vi "Multichannel Lockin--DELETINGSTATES.vi"() -> ()   [LabVIEW 2019, in "Instrument.Lockin.lvclass"]
uses:
  Instrument.Lockin/Instrument.Lockin.lvclass
  <vilib>/Utility/error.llb/DialogType.ctl
  <vilib>/measure/NI_MAPro.lvlib
  <vilib>/Utility/config.llb/NI_LVConfig.lvlib
  <vilib>/JKI/JKI SMO/SMO/SMO.lvclass
  <userlib>/LevyLab/Instrument Framework/SMOs/RemoteControl/RemoteControl.lvclass
  <userlib>/LevyLab/Instrument Framework/SMOs/RemoteControl/Typedefs/Message--Cluster.ctl
  <userlib>/LevyLab/Instrument Framework/SMOs/RemoteControl/Typedefs/PrivateEvents--RemoteControl.Configure.ctl
  Instrument.DAQ/Typedefs/Results--Cluster.ctl
  Instrument.DAQ/Instrument.DAQ.lvclass
  Instrument.DAQ/Typedefs/Set State-enum.ctl
  <vilib>/JKI/JKI SMO/SMO/Typedefs/Reserve State--Enum.ctl
  <vilib>/JKI/JKI SMO/SMO/Typedefs/Public Events.ctl
  <vilib>/JKI/JKI SMO/SMO/Typedefs/SMOState --Enum.ctl
  Instrument.DAQ/Typedefs/DAQ.Sample Mode--Ring.ctl
  Instrument.DAQ/Typedefs/Sweep.Configuration--Cluster.ctl
  Instrument UI.Lockin/Instrument UI.Lockin.lvclass
  Instrument.DAQ/Typedefs/PublicEvents--DAQ.getSweepWaveforms.ctl
  Instrument.DAQ/Typedefs/PrivateEvents--DAQ.setCalibration.ctl
  Instrument.DAQ/Typedefs/Sweep.Pattern--Enum.ctl
  Instrument.DAQ/Typedefs/Sweep.Channel--Cluster.ctl
  Instrument.DAQ/Typedefs/DAQ.Sampling--Cluster.ctl
  Instrument UI.Lockin/private/Set Legend (WFChart).vi
  Instrument UI.Lockin/private/Set Legend (WFGraph).vi
  Instrument UI.Lockin/private/Set Legend (WDTWFGraph).vi
  Instrument UI.Lockin/private/Set All Plot Visibility (WFGraph).vi
  Instrument UI.Lockin/private/Set All Plot Visibility (WFChart).vi
  <vilib>/Platform/browser.llb/Open URL in Default Browser (string).vi
  <userlib>/LevyLab/Instrument Framework/SMOs/Instrument/Instrument.lvclass
  Instrument UI.Lockin/private/Set Plot Visibility (WFGraph).vi
  Instrument UI.Lockin/private/Set Plot Visibility (WFChart).vi
  <userlib>/LevyLab/Instrument Framework/SMOs/Logger.Error/Logger.Error.lvclass
  C:/Program Files (x86)/National Instruments/LabVIEW 2019/vi.lib/JKI/JKI SMO/SMO/SMO.lvclass
  Instrument UI.Lockin/private/Set All Plot Visibility (XYGraph).vi
  Instrument UI.Lockin/private/Set Plot Visibility (XYGraph).vi
  <userlib>/_OpenG.lib/error/error.llb/Filter Error Codes (Array)__ogtk.vi
  <vilib>/Waveform/WDTOps.llb/WDT Waveform Duration DBL.vi
  Instrument.DAQ/Typedefs/Sweep.Channel--Cluster--Array.ctl
  <vilib>/measure/maspectr.llb/FFT Power Spectrum and PSD for N Chan.vi
  Instrument.DAQ/Typedefs/DAQ.Config.AI.Coupling--enum.ctl
  Instrument.DAQ/Typedefs/DAQ.Config.AI.Range--enum.ctl
  Instrument.DAQ/Typedefs/DAQ.Config.AO.Range--enum.ctl
  Instrument.DAQ/Typedefs/AO.Channel.Function--Enum.ctl
  Instrument.DAQ/Typedefs/DAQ.Calibration--Cluster.ctl
  Instrument.DAQ/Typedefs/DAQ.Type--enum.ctl
  Instrument UI.Lockin/Typedefs/Display-Enum.ctl
  Instrument.DAQ/Typedefs/Simulation Mode--enum.ctl
  Instrument.Lockin/Typedefs/Lockin.Auto Sample Mode--Enum.ctl
  Instrument.DAQ/Typedefs/DAQ.Configuration--Cluster.ctl
  Instrument.DAQ/Typedefs/REF.Channel--Cluster.ctl
  Instrument.Lockin/Typedefs/Results Type--Enum.ctl
panel:
  out "Results Plot Names":string[](array[string])
  out "Version":string="vDevelopment" caption="V"
  in  "Tab Control 4":T1(tab)
  in  "Disable all AI Ref":bool
  in  "Enable only AI Ref1":bool
  in  "Reset Phase":bool
  in  "AI Channels":T2(array[cluster]) {"References" items=["", "1"]}
  in  "AO freq link":dbl=13.0 format="%.3p"
  in  "AO Amp Limit":dbl=0.009999999 format="%.3p"
  in  "Limit Amplitudes":bool
  in  "Link Frequencies":bool
  in  "LP f (Hz)":dbl=100.0 format="%.3p"
  in  "Line":bool
  in  "Lowpass":bool
  in  "AO Channels":T4(array[cluster]) {"Phase" format="%.3g"; "Frequency" min=0.0001 max=10000.0 format="%.3g"; "Offset" format="%.3p"; "Amplitude" min=0.0 max=10.0 format="%.3p"}
  in  "REF Channels":T5[](array[typedef]) {"Roll-Off" min=1; "TC" min=0.0001 format="%#_3p"; "Phase" format="%.3g"; "Frequency" min=0.0001 max=10000.0 format="%.3g"; "Channel" min=1}
  in  "DAQ Config":T6[](array[typedef]) {"AI.Coupling" items=["AC"=10045, "DC"=10050, "GND"=10066]}
  in  "auto DAQ":bool
  in  "Max Fs Refresh Rate (Hz)":dbl=10.0 format="%#_13g"
  in  "Sampling Mode":T10
  in  "Sampling":T11={"Fs"=10000.0, "#s"=1000}
  in  "DAQ Type":T12=enum."PXI 446x"
  in  "Auto x*F1":dbl=5000.0 format="%#_13g"
  in  "Load Configuration":bool
  in  "Save Configuration":bool
  in  "AI Simulation mode":T13=enum."AI = noise*AO"
  in  "decimating factor":i32=1
  in  "Remove":bool
  in  "Measure":bool
  in  "Channels: Sweep":T15(array[cluster]) {"Channel" items=["AO1"=1, "AO2"=2, "AO3"=3, "AO4"=4, "AO5"=5, "AO6"=6, "AO7"=7, "AO8"=8]; "Start" format="%#_6p"; "End" format="%#_6p"}
  in  "Stop Sweep":bool caption="Stop"
  in  "Sweep Time (s)":dbl=20.0 format="%#_1f"
  in  "Start Sweep":bool caption="Start"
  in  "Initial Wait (s)":dbl=1.0
  out "Sweep Timer (s)":dbl caption="Timer (s)"
  in  "Return to Start?":bool
  out "Sampling Status":string="Good"
  in  "Output Gain":cluster{"AI.Ch":string, "Gain":dbl}[](array[cluster])=[{"AI.Ch"="AO1", "Gain"=1.0}, {"AI.Ch"="AO2", "Gain"=1.0}, {"AI.Ch"="AO3", "Gain"=1.0}, {"AI.Ch"="AO4", "Gain"=1.0}, {"AI.Ch"="AO5", "Gain"=1.0}, {"AI.Ch"="AO6", "Gain"=1.0}, {"AI.Ch"="AO7", "Gain"=1.0}, {"AI.Ch"="AO8", "Gain"=1.0}, {"AI.Ch"="AO9", "Gain"=1.0}, {"AI.Ch"="AO10", "Gain"=1.0}, {"AI.Ch"="AO11", "Gain"=1.0}, {"AI.Ch"="AO12", "Gain"=1.0}, {"AI.Ch"="AO13", "Gain"=1.0}, {"AI.Ch"="AO14", "Gain"=1.0}, {"AI.Ch"="AO15", "Gain"=1.0}, {"AI.Ch"="AO16", "Gain"=1.0}]
  in  "Input Gain":cluster{"AI.Ch":string, "Gain":dbl}[](array[cluster])=[{"AI.Ch"="AI1", "Gain"=1.0}, {"AI.Ch"="AI2", "Gain"=1.0}, {"AI.Ch"="AI3", "Gain"=1.0}, {"AI.Ch"="AI4", "Gain"=1.0}, {"AI.Ch"="AI5", "Gain"=1.0}, {"AI.Ch"="AI6", "Gain"=1.0}, {"AI.Ch"="AI7", "Gain"=1.0}, {"AI.Ch"="AI8", "Gain"=1.0}, {"AI.Ch"="AI9", "Gain"=1.0}, {"AI.Ch"="AI10", "Gain"=1.0}, {"AI.Ch"="AI11", "Gain"=1.0}, {"AI.Ch"="AI12", "Gain"=1.0}, {"AI.Ch"="AI13", "Gain"=1.0}, {"AI.Ch"="AI14", "Gain"=1.0}, {"AI.Ch"="AI15", "Gain"=1.0}, {"AI.Ch"="AI16", "Gain"=1.0}]
  out "State History":string=" Exit\r Data: Cleanup\r Events: Unregister\r UI: Cleanup\r UI: Disable Buttons\r Configuration: Write\r Error Logger: Destroy\r Lockin SMO: Stop\r Remote SMO: Stop\r Macro: Exit\r UI: Update Sweep Timer\r UI: Update Lockin Graphs\r UI: Update Waveform Graphs\r 4461: OUT\r UI: Update Sweep Timer\r UI: Update Lockin Graphs\r UI: Update Waveform Graphs\r 4461: OUT\r UI: Update Sweep Timer\r UI: Update Lockin Graphs\r UI: Update Waveform Graphs\r 4461: OUT"
  out "Refresh time (ms)":u32=103
  out "LockinDAQ SMO State":T16=enum."Stopped" caption="SMO State"
  out "RC SMO State":T16=enum."Stopped" caption="SMO State"
  in  "Update":bool
  in  "Enable Output":bool caption="Enable"
  in  "Output Channel":i32=1 min=1
  out "Output (V)":dbl
  in  "AI Channel":i32=1
  in  "Reference Channel":i32=1
  in  "Type":T17
  in  "Allowed remote system":string
  in  "Get Calibration":bool
  out "Cal Info":T18[](array[typedef]) {"SelfCal.LastDate/Time" format="%<%I:%M %p\n%m/%d/%Y>T"}
  in  "Self Calibrate":bool
  in  "Tab Control 3":enum32{"Page 1"}(tab)
  out "X":dbl=0.0014996100939563214 caption="X (V)" format="%#_3p"
  out "Y":dbl=-29.79492153733761 caption="Y (V)" format="%#_3p"
  in  "Channel":i32(ring)=1
  out "R":dbl=0.0014996100939563214 caption="R (V)" format="%#_3p"
  out "Theta":dbl=-29.79492153733761 caption="Theta (°)" format="%#_3p"
  in  "Display":T19=enum."R and Theta" caption="Enum"
  in  "Close":bool
  out "Status":string="Shutdown"
  in  "Pause":bool
  in  "Reset":bool
  in  "Start":bool
  in  "Help":bool
  in  "Trigger":bool
  in  "Tab Control 2":T20(tab)
  in  "AI Graph All":bool
  in  "AI Graph None":bool
  in  "Y Axis (Output)":enum16{"Analog Output", "Reference"}(ring) caption="Enum 3"
  in  "Y Axis (Input)":enum16{"Device", "ADC"}(ring) caption="Enum 3"
  in  "Decimate":enum16{"1", "10", "100", "1000"}(ring) caption="Enum 3"
  in  "X Axis":enum16{"Time", "Samples"}(ring) caption="Enum 3"
  out "AI Graph":waveform(dbl)[](graph)
  out "AO Graph":waveform(dbl)[](graph)
  in  "AO Graph All":bool
  in  "AO Graph None":bool
  in  "Y/Theta Range":dbl caption="Axis Range" format="%#_6p"
  in  "X/R Range":dbl caption="Axis Range" format="%#_6p"
  out "Lockin 2":waveform(dbl)[](graph) caption="Lockin Display 2"
  out "Lockin 1":waveform(dbl)[](graph)
  in  "Lockin 1 None":bool
  in  "Lockin 1 All":bool
  out "Results":string[][](table)
  out "XY Graph":cluster{"Wavenumber":dbl[], "Data":dbl[]}[](graph)
  in  "Numeric":dbl caption="Axis Range" format="%#_6p"
  out "Sweep Results Y":waveform(dbl)[](graph)
  out "Sweep Results X":waveform(dbl)[](graph)
  out "Sweep Results AI":waveform(dbl)[](graph)
  out "Sweep Results AO":waveform(dbl)[](graph)
  in  "# averages":u32=10 min=1
  in  "weighting mode":enum16{"Linear", "Exponential"}(ring)=enum."Exponential"
  in  "averaging mode":T21(ring)=enum."RMS averaging"
  in  "window":u16(ring) items=["Rectangle", "Hanning"]
  in  "export mode":u16(ring)=1 items=["Power Spectrum", "Power Spectral Density"]
  in  "restart":bool
  out "done?":bool=TRUE
  out "PS Chart":dbl[][](graph)
  out "PS WFGraph":cluster{"f0":dbl, "df":dbl, "magnitude":dbl[]}[](graph)
  out "averages":dbl=180.0
  # "Output"
  # "Input"
  # ">> DEVICE >>"
  # "Amp (V)"
  # "(*)"
  # "Ch"
  # "DC (V)"
  # "f (Hz)"
  # "Phase (°)"
  # "Function"
  # "Sweep"
  # "(*)"
  # "Ch"
  # "Ref1   2     3    4"
  # "Input: Pre-Filter"
  # "Output Settings"
  # "Reference"
  # "Reference Settings"
  # "Ch"
  # "f (Hz)"
  # "Phase (°)"
  # "TC (s)"
  # "Order"
  # "DAQ Channels"
  # "AI"
  # "Device"
  # "AO"
  # "Input: Offset"
  # "Ch"
  # "Range"
  # "Ch"
  # "Range"
  # "Coupling"
  # "Other Configuration"
  # "Sampling"
  # "Changing settings in this box will automatically\nreset the lockin and restart acquisition"
  # "Sweep"
  # "Channel"
  # "Start"
  # "End"
  # "Pattern"
  # "Status"
  # "Channel"
  # "Channel"
  # "Input Gain"
  # "Output Gain"
  # "Auxiliary Output"
  # "Configuration"
  # "- Use to control an auxiliiary card such as a multifunction DAQ (6115, 6120, etc)"
  # "Forward Lockin Input --> Lockin Output"
  # "- Choose an input lockin channel and value (X,Y, etc) and it will be written as a DC value to an output channel of your choosing.\n- Output is scaled by the input amplifier gain."
  # "Calibration"
  # "Self Cal\nLast Time"
  # "Self Cal\nLast Temp"
  # "Temp\nNow"
  # "Cal\nDue"
  # "Device"
  # "AI Graph"
  # "AO/Reference Graph"
  # "Lockin Results 1"
  # "Lockin Results 2"
  # "Lockin Results 2"
  # "Sweep Results"
  # "Sweep AO/AI"
  # "Power Spectra"
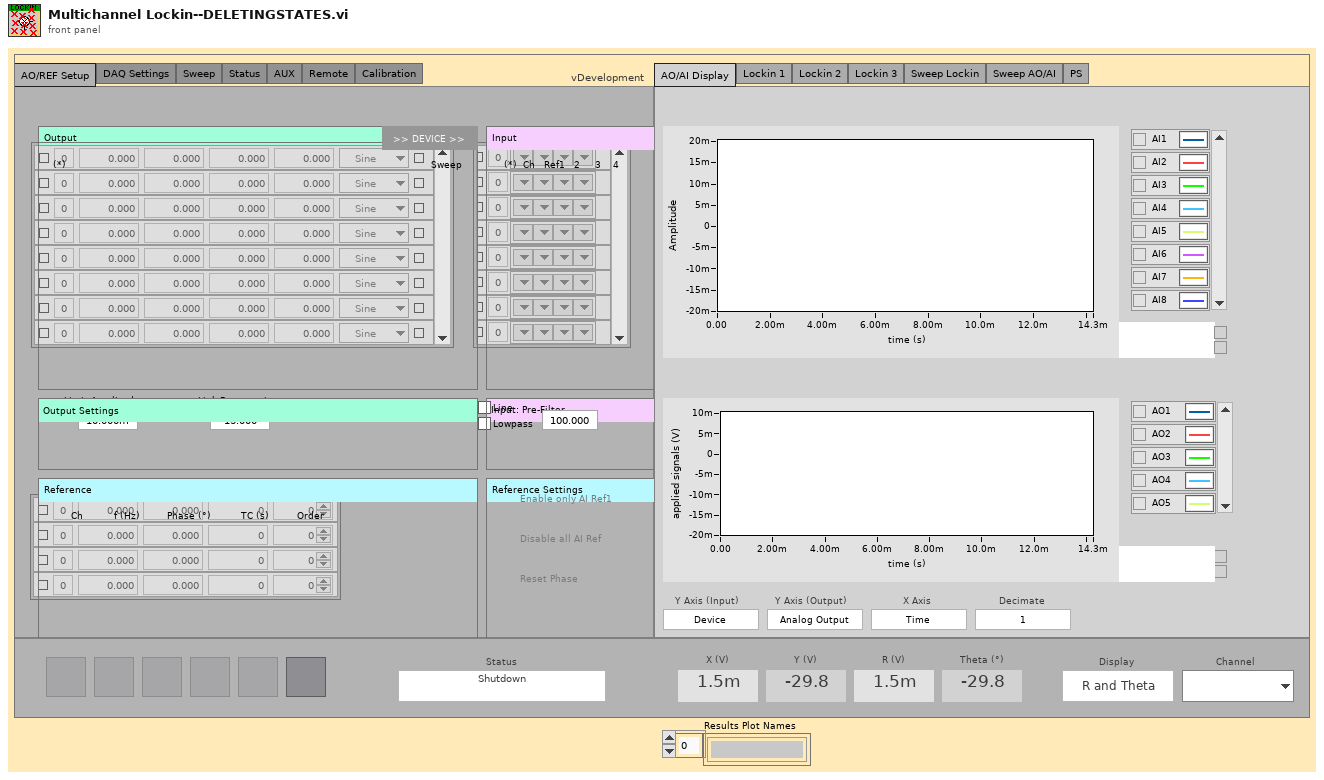
[diagram p1: front panel]
types:
  T1 = enum32{"AO/REF Setup", "DAQ Settings", "Sweep", "Status", "AUX", "Remote", "Calibration"}
  T2 = cluster{"Enable?":bool, "Channel":i32, "References":u16[]}[]
  T3 = typedef "Instrument.DAQ.lvclass/AO.Channel.Function--Enum.ctl" = enum16{"Sine", "Triangle", "Square"}
  T4 = cluster{"Enable?":bool, "Channel":i32, "Amplitude":dbl, "Offset":dbl, "Frequency":dbl, "Phase":dbl, "Function":T3, "Sweeping?":bool}[]
  T5 = typedef "Instrument.DAQ.lvclass/REF.Channel--Cluster.ctl" = cluster{"Enable?":bool, "Channel":i32, "Frequency":dbl, "Phase":dbl, "TC":dbl, "Roll-Off":i32}
  T6 = typedef "Instrument.DAQ.lvclass/DAQ.Configuration--Cluster.ctl" = cluster{"Device":string, "AO.Ch":string, "AO.Range":T7, "AI.Ch":string, "AI.Range":T8, "AI.Coupling":T9}
  T7 = typedef "Instrument.DAQ.lvclass/DAQ.Config.AO.Range--enum.ctl" = enum16{"±0.1", "±1.0", "±10.0"}
  T8 = typedef "Instrument.DAQ.lvclass/DAQ.Config.AI.Range--enum.ctl" = enum16{"±0.316", "±1.00", "±3.16", "±10.0", "±31.6", "±42.4"}
  T9 = typedef "Instrument.DAQ.lvclass/DAQ.Config.AI.Coupling--enum.ctl" = u16
  T10 = typedef "Instrument.Lockin.lvclass/Lockin.Auto Sample Mode--Enum.ctl" = enum16{"Manual", "Auto Fs", "Max Fs"}
  T11 = typedef "Instrument.DAQ.lvclass/DAQ.Sampling--Cluster.ctl" = cluster{"Fs":dbl, "#s":i32}
  T12 = typedef "Instrument.DAQ.lvclass/DAQ.Type--enum.ctl" = enum16{"None", "USB 4431", "PXI 446x"}
  T13 = typedef "Instrument.DAQ.lvclass/Simulation Mode--enum.ctl" = enum16{"AI = HW simulated", "AI = noise*AO", "AI = waveguide"}
  T14 = typedef "Instrument.DAQ.lvclass/Sweep.Pattern--Enum.ctl" = enum16{"Ramp /", "Ramp /\\", "Smooth Ramp _/", "Smooth Ramp _/\\_", "Frequency"}
  T15 = cluster{"Enable?":bool, "Channel":u16, "Start":dbl, "End":dbl, "Pattern":T14}[]
  T16 = typedef "SMO.lvclass/SMOState --Enum.ctl" = enum16{"unknown", "Created", "Started", "Stopped"}
  T17 = typedef "Instrument.Lockin.lvclass/Results Type--Enum.ctl" = enum16{"X", "Y", "R", "Theta", "Mean"}
  T18 = typedef "Instrument.DAQ.lvclass/DAQ.Calibration--Cluster.ctl" = cluster{"Active Device":string, "SelfCal.LastDate/Time":dbl, "SelfCal.LastTemp":dbl, "DevTemp":dbl, "calibration due?":bool}
  T19 = typedef "Instrument UI.Lockin.lvclass/Display-Enum.ctl" = enum16{"X and Y", "R and Theta", "Mean"}
  T20 = enum32{"AO/AI Display", "Lockin 1", "Lockin 2", "Lockin 3", "Sweep Lockin", "Sweep AO/AI", "PS"}
  T21 = enum16{"No averaging", "Vector averaging", "RMS averaging", "Peak hold"}
  T22 = typedef "Instrument.DAQ.lvclass/Set State-enum.ctl" = enum16{"start", "stop", "reset", "start sweep", "stop sweep"}
  T23 = typedef "Instrument.DAQ.lvclass/PrivateEvents--DAQ.setCalibration.ctl" = enum16{"Check", "Calibrate"}
  T24 = typedef "Instrument.DAQ.lvclass/Sweep.Configuration--Cluster.ctl" = cluster{"Sweep Time (s)":dbl, "Initial Wait (s)":dbl, "Return to Start":bool, "Channels":T25}
  T25 = typedef "Instrument.DAQ.lvclass/Sweep.Channel--Cluster--Array.ctl" = T26[]
  T26 = typedef "Instrument.DAQ.lvclass/Sweep.Channel--Cluster.ctl" = cluster{"Enable?":bool, "Channel":u16, "Start":dbl, "End":dbl, "Pattern":T14}
  T27 = enum32{"invalid app kind", "Development System", "Run Time System", "Student Edition", "Embedded LabVIEW", "Evaluation", "Custom"}
  T28 = enum32{"AO/REF Setup", "DAQ Settings", "Sweep", "Status", "AUX", "Remote", "Calibration", "Save"}
  T29 = enum8{"Enabled", "Disabled", "Disabled and Grayed Out"}
  T30 = enum32{"Invalid", "Standard", "Closed", "Hidden", "Minimized", "Maximized"}
  T31 = cluster{"averaging mode":enum16{"No averaging", "Vector averaging", "RMS averaging", "Peak hold"}, "weighting mode":enum16{"Linear", "Exponential"}, "number of averages":u32}
  T32 = typedef "Instrument.DAQ.lvclass/Get State-enum.ctl" = enum16{"idle", "created", "started", "stopped", "sweeping"}
  T33 = typedef "RemoteControl.lvclass/PrivateEvents--RemoteControl.Configure.ctl" = cluster{"address":string, "Port":u16, "AllowedRemote":string, "Commands":string[], "timeout":i32}
  T34 = typedef "RemoteControl.lvclass/Message--Cluster.ctl" = cluster{"Command":string, "Data":variant, "ID":string}
  T35 = typedef "Instrument.DAQ.lvclass/PublicEvents--DAQ.getSweepWaveforms.ctl" = cluster{"Sweep AO":waveform(dbl)[], "Sweep AI":waveform(dbl)[], "Sweep Results X":waveform(dbl)[], "Sweep Results Y":waveform(dbl)[]}
  T36 = cluster{"Core":cluster{"Current VI Reference":refnum<vi>, "Close Panel on Exit?":bool}, "to":i32, "Lockin":refnum<class "Instrument.Lockin.lvclass">, "RemoteControl":refnum<class "RemoteControl.lvclass">, "Lockin.DAQ":refnum<class "Instrument.DAQ.lvclass">, "Logger.Error":refnum<class "Logger.Error.lvclass">, "RemoteControl.Configure":T33, "Message":T34, "HandledMessage":T34, "SweepWaveforms":T35}
  T37 = typedef "Instrument.DAQ.lvclass/State-enum.ctl" = enum16{"idle", "created", "started", "stopped", "sweeping"}
  T38 = typedef "Instrument.DAQ.lvclass/REF.Channel--Cluster--Array.ctl" = T5[]
  T39 = typedef "Instrument.DAQ.lvclass/DAQ Configuration--Cluster--Array.ctl" = T40[]
  T40 = typedef "Instrument.DAQ.lvclass/DAQ Configuration--Cluster.ctl" = cluster{"Device":string, "AO.Ch":string, "AO.Range":T41, "AI.Ch":string, "AI.Range":T42, "AI.Coupling":T43}
  T41 = typedef "Instrument.DAQ.lvclass/446xAO-enum.ctl" = enum16{"±0.1", "±1.0", "±10.0"}
  T42 = typedef "Instrument.DAQ.lvclass/446xAI-enum.ctl" = enum16{"±0.316", "±1.00", "±3.16", "±10.0", "±31.6", "±42.4"}
  T43 = typedef "Instrument.DAQ.lvclass/AI.coupling-enum.ctl" = u16
  T44 = typedef "Instrument.DAQ.lvclass/DAQ.Config.AO--Cluster--Array.ctl" = T45[]
  T45 = typedef "Instrument.DAQ.lvclass/DAQ.Config.AO--Cluster.ctl" = cluster{"Channels":tag, "Range":T7, "output terminal configuration":i32, "Type":T12}
  T46 = typedef "Instrument.DAQ.lvclass/DAQ.Config.AI--Cluster--Array.ctl" = T47[]
  T47 = typedef "Instrument.DAQ.lvclass/DAQ.Config.AI--Cluster.ctl" = cluster{"Channels":tag, "Coupling":T9, "Range":T8, "input terminal configuration":i32, "Type":T12}
  T48 = typedef "Instrument.DAQ.lvclass/DAQ.Sample Mode--Ring.ctl" = i32
  T49 = typedef "DialogType.ctl" = u16
  T50 = typedef "Instrument.DAQ.lvclass/Results--Cluster.ctl" = cluster{"Time Stamp":timestamp, "Results (Dictionary)":cluster{"key":string, "value":dbl}[]}
  T51 = cluster{"Current VI Reference":refnum<vi>, "Close Panel on Exit?":bool}
  T52 = typedef "Instrument.DAQ.lvclass/AO.Channel--Cluster--Array.ctl" = T53[]
  T53 = typedef "Instrument.DAQ.lvclass/AO.Channel--Cluster.ctl" = cluster{"Enable?":bool, "Channel":i32, "Amplitude":dbl, "Offset":dbl, "Frequency":dbl, "Phase":dbl, "Function":T3, "Sweeping?":bool}
  T54 = typedef "SMO.lvclass/Public Events.ctl" = cluster{"Error":refnum<user-event>, "State":refnum<user-event>, "Reserve State":refnum<user-event>}
  T55 = typedef "RemoteControl.lvclass/PublicEvents--Cluster.ctl" = cluster{"SendMessageFromProcess":refnum<user-event>}
  T56 = typedef "Instrument.DAQ.lvclass/PublicEvents--Cluster.ctl" = cluster{"getAIChannels":refnum<user-event>, "getAOChannels":refnum<user-event>, "getREFChannels":refnum<user-event>, "getWaveforms":refnum<user-event>, "getResults":refnum<user-event>, "getSweepWaveforms":refnum<user-event>, "getCalibration":refnum<user-event>, "getDAQState":refnum<user-event>, "getDAQconfig":refnum<user-event>}
  T57 = typedef "Instrument.DAQ.lvclass/AI.Channel--Cluster--Array.ctl" = T58[]
  T58 = typedef "Instrument.DAQ.lvclass/AI.Channel--Cluster.ctl" = cluster{"Enable?":bool, "Channel":i32, "References":i32[]}
  T59 = typedef "Instrument.DAQ.lvclass/Configuration.Prefilter--Cluster.ctl" = cluster{"60 Hz":bool, "Low Pass":bool, "Low Pass Cutoff (Hz)":dbl}
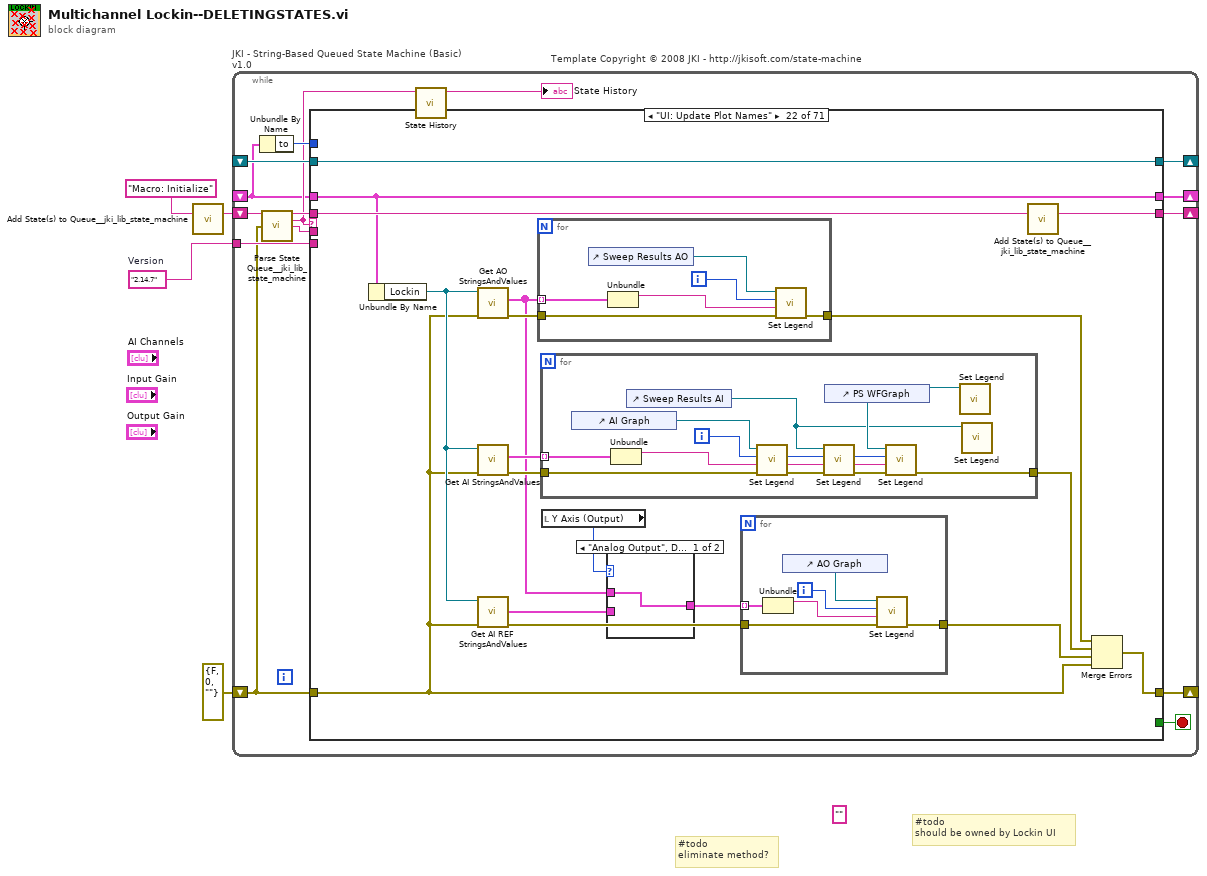
[diagram p0: block diagram]
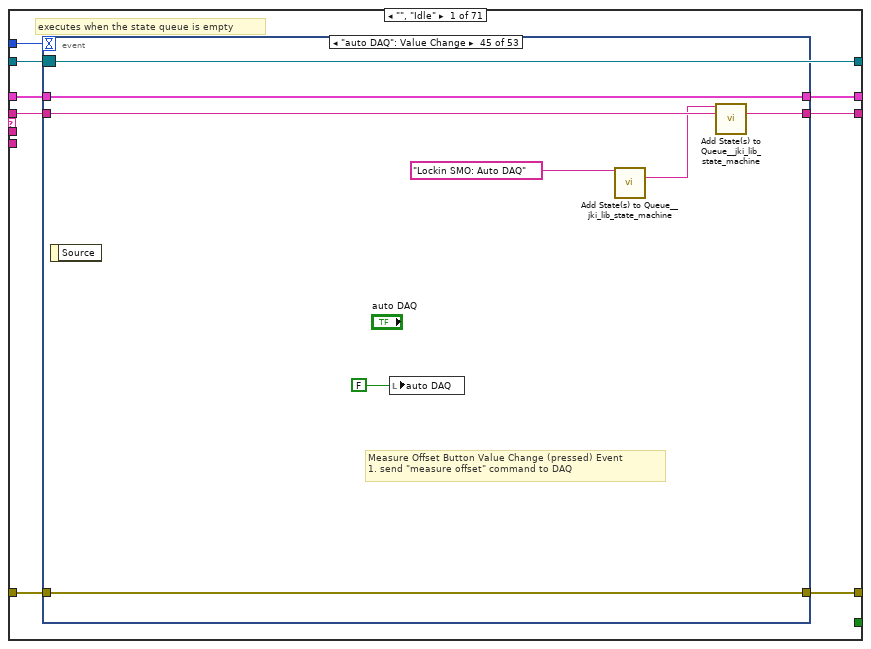
[diagram p2: hidden frame]
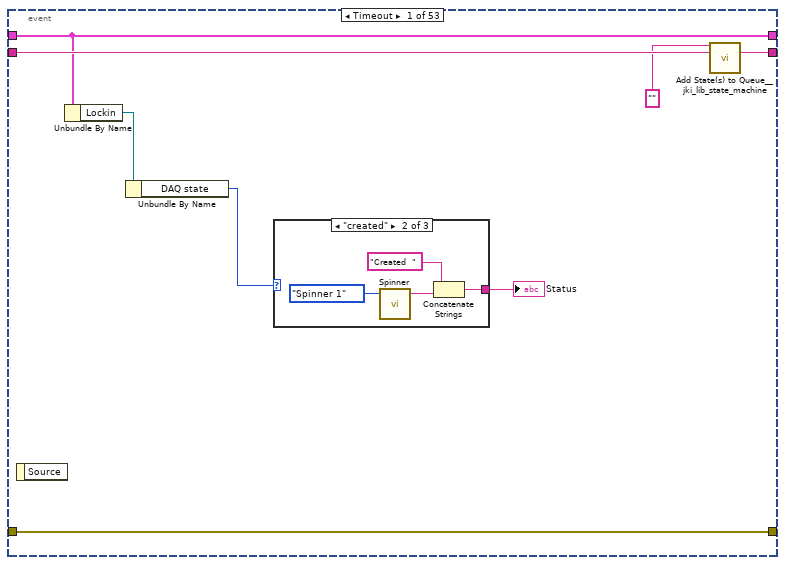
[diagram p3: hidden frame]
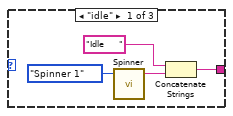
[diagram p4: hidden frame]
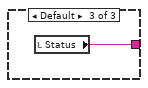
[diagram p5: hidden frame]
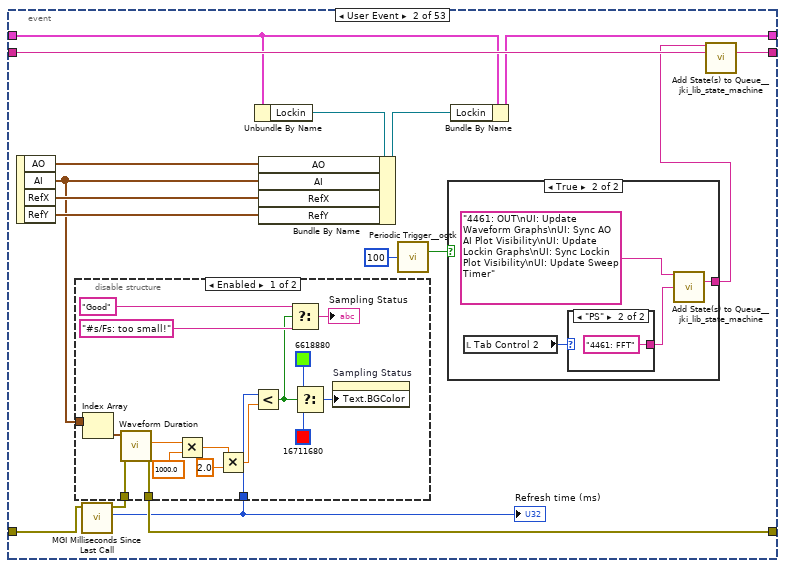
[diagram p6: hidden frame]
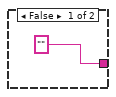
[diagram p7: hidden frame]
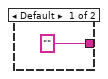
[diagram p8: hidden frame]
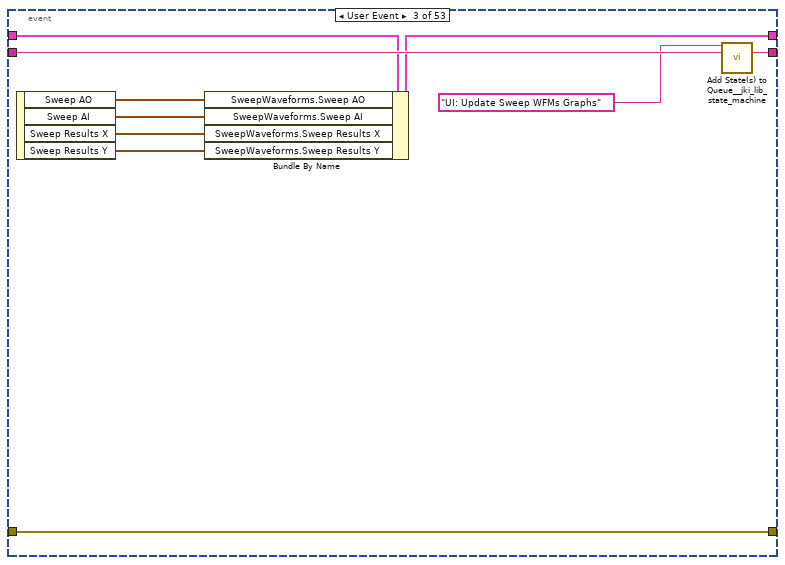
[diagram p10: hidden frame]
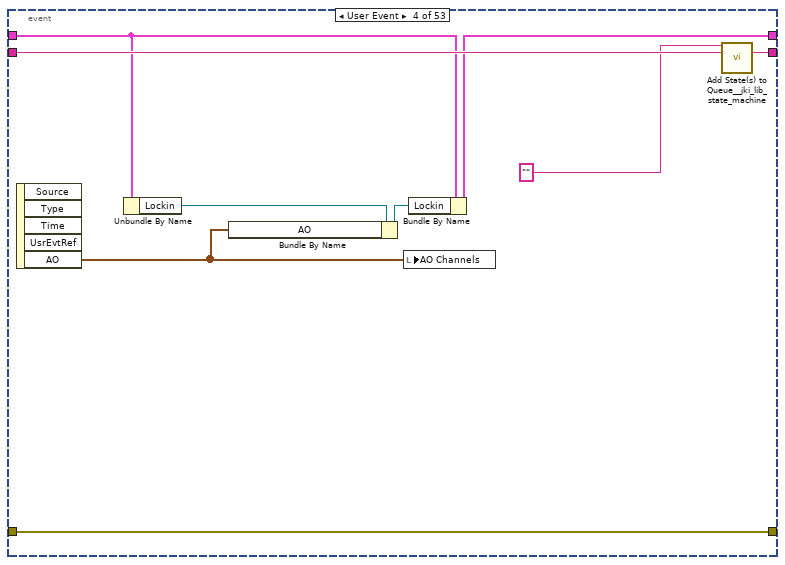
[diagram p11: hidden frame]
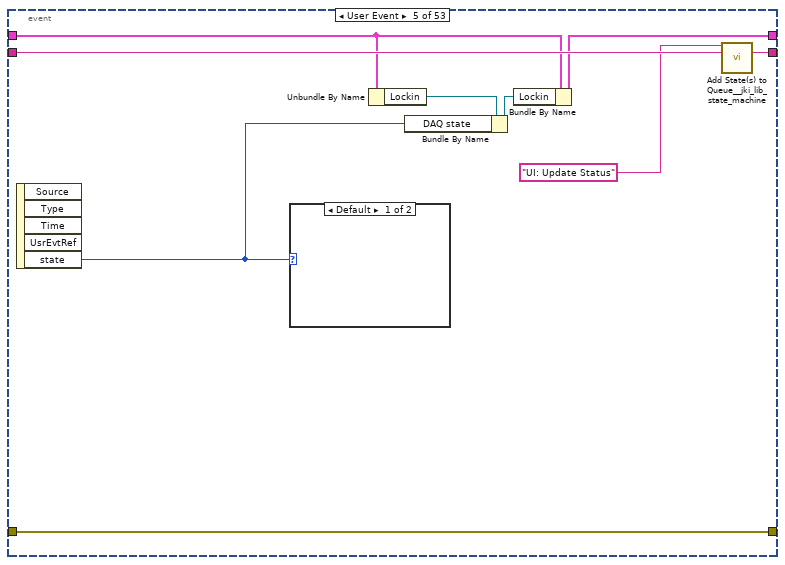
[diagram p12: hidden frame]
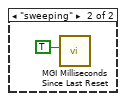
[diagram p13: hidden frame]
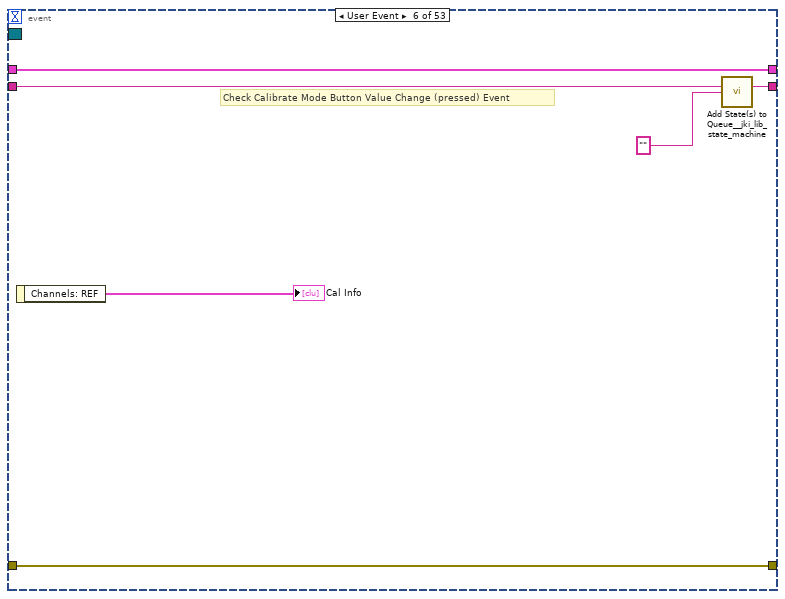
[diagram p14: hidden frame]
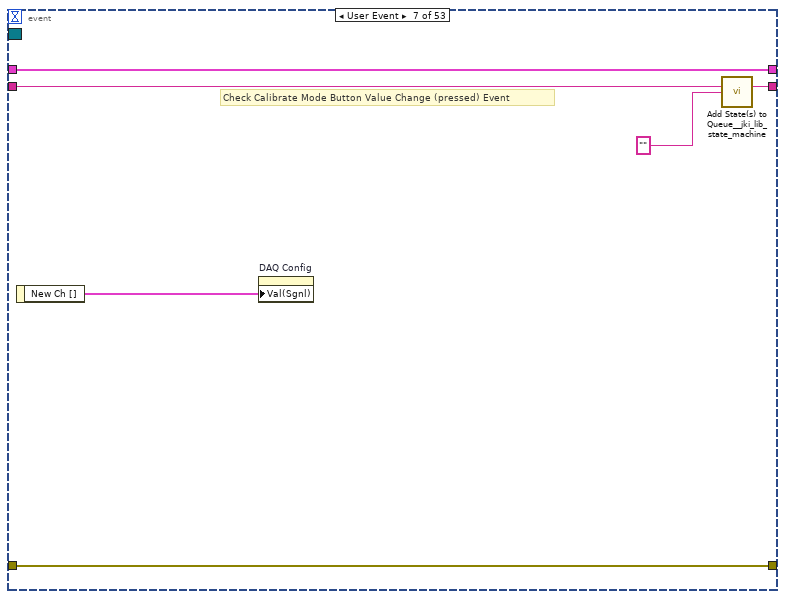
[diagram p15: hidden frame]
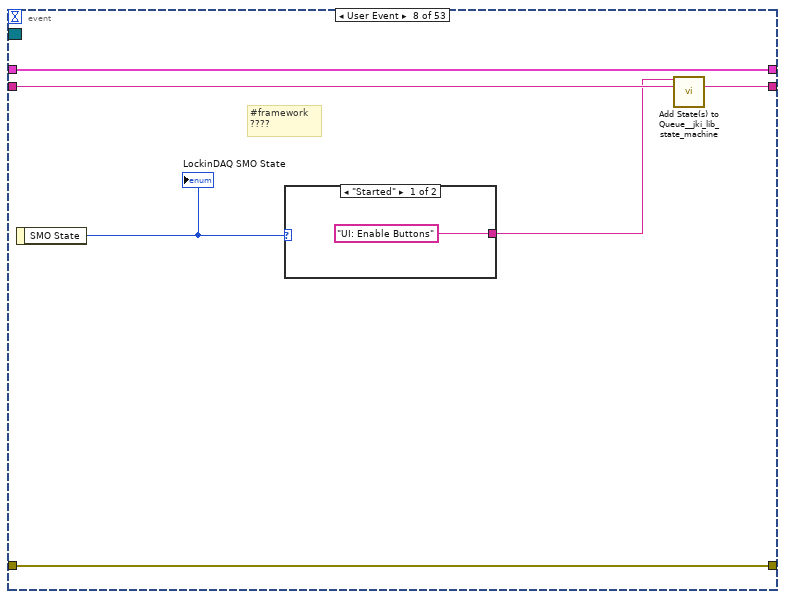
[diagram p16: hidden frame]
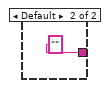
[diagram p17: hidden frame]
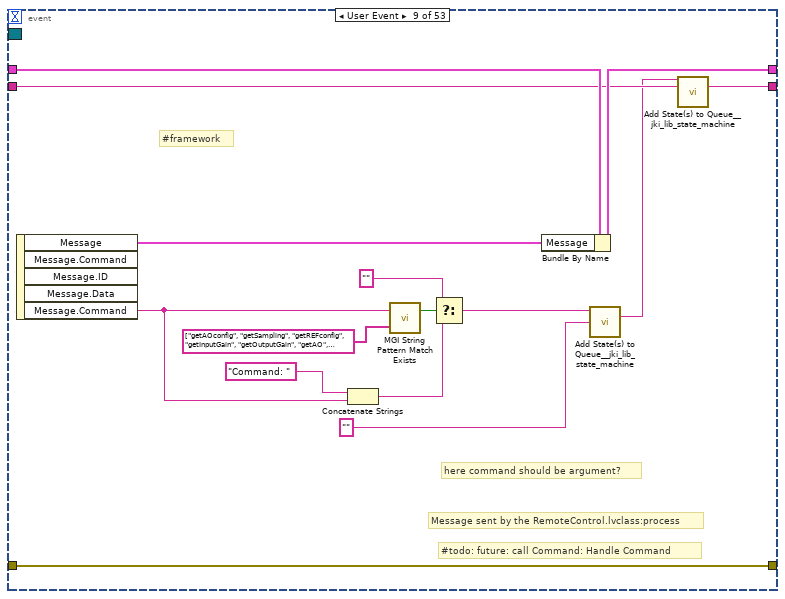
[diagram p18: hidden frame]
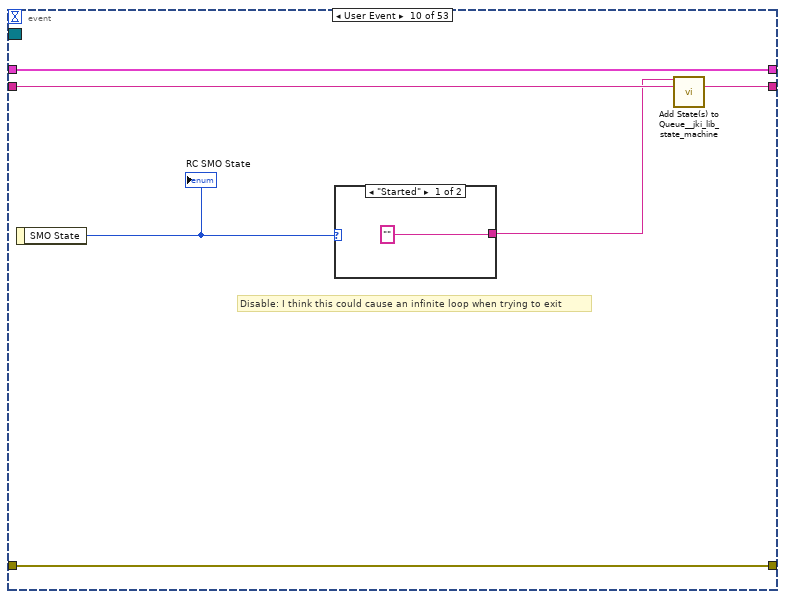
[diagram p19: hidden frame]
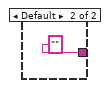
[diagram p20: hidden frame]
diagram:
  (unwired) "" ("State(s) in Front (\"\")")
  w2 = "2.14.7"  # Version
  # "#todo\nshould be owned by Lockin UI"
  # "#todo\neliminate method?"
  # "Template Copyright © 2008 JKI - http://jkisoft.com/state-machine"
  n1 = call <vilib>:"Add State(s) to Queue__jki_lib_state_machine.vi"("State(s) in (\"\")"="Macro: Initialize") -> ("States Out"=w4:string)  [unwired: 14 in]
  n2 = while "JKI - String-Based Queued State Machine (Basic) v1.0" {
    shift-right: [w11] -> _
    shift-left: _ -> [w5]
    shift-right: [w8] -> _
    shift-left: errorcluster {"status"=FALSE, "code"=0, "source"=""} ("error out") -> [w6]
    shift-right: [w18] -> _
    shift-left: w4 -> [w15]
    shift-right: [w12] -> _
    shift-left: _ -> [w13]
    tunnel: w2 -> [w7]
    stop <- w17 stop-if-true
    n3 = Unbundle By Name(w5) -> ("to"=w14:i32)
    n4 = call <vilib>:"Parse State Queue__jki_lib_state_machine.vi"("State Queue"=w15, "Error In (no error)"=w6) -> ("Remaining States"=w16:string, "Current State"=w9:string, "Arguments"=w19:string)  [unwired: 11 in]
    n5 = case shown="\"UI: Update Plot Names\"" w9 {
      selector: w9 -> [_ _ w594 _ _ _ _ _ _ _ _ _ _ _ _ _ _ _ _ _ _ _ _ _ _ _ _ _ _ _ _ _ _ _ _ _ _ _ _ _ _ _ _ _ _ _ _ _ _ _ _ _ _ _ _ _ _ _ _ _ _ _ _ _ _ _ _ _ _ _ _]
      tunnel: w19 -> [_ _ _ _ _ _ _ _ _ _ _ _ _ _ _ _ _ _ w780 _ _ _ _ _ _ _ w1000 w1014 w1033 _ _ _ _ _ _ _ _ _ w1195 w1205 _ _ _ _ _ _ _ _ w1334 _ _ w1374 _ _ _ _ _ _ _ w1461 _ _ _ _ _ _ _ _ _ _ _]
      tunnel: [w26 w590 w597 w615 w628 w640 w645 w660 w681 w688 w693 w718 w724 w729 w745 w756 w767 w778 w791 w811 w829 w850 w892 w949 w978 w991 w1004 w1017 w1036 w1067 w1097 w1110 w1121 w1129 w1145 w1152 w1160 w1180 w1196 w1208 w1240 w1245 w1252 w1257 w1265 w1303 w1325 w1330 w1340 w1360 w1369 w1381 w1392 w1409 w1421 w1430 w1439 w1448 w1457 w1468 w1475 w1482 w1489 w1496 w1501 w1515 w1543 w1583 w1592 w1597 w1602] -> w18
      tunnel: [_ _ _ _ _ TRUE _ _ _ _ _ _ _ _ _ _ _ _ _ _ _ _ _ _ _ _ _ _ _ _ _ _ _ _ _ _ _ _ _ _ _ _ _ _ _ _ _ _ _ _ _ _ _ _ _ _ _ _ _ _ _ _ _ _ _ _ _ _ _ _ _] -> w17
      tunnel: w14 -> [w21 _ _ _ _ _ _ _ _ _ _ _ _ _ _ _ _ _ _ _ _ _ _ _ _ _ _ _ _ _ _ _ _ _ _ _ _ _ _ _ _ _ _ _ _ _ _ _ _ _ _ _ _ _ _ _ _ _ _ _ _ _ _ _ _ _ _ _ _ _ _]
      tunnel: w16 -> [w27 w591 w598 w616 w629 w641 w646 w661 w682 w689 w694 w719 w725 w730 w746 w757 w768 w779 w792 w812 w830 w851 w893 w950 w979 w992 w1005 w1018 w1037 w1068 w1098 w1111 w1122 w1130 w1146 w1153 w1161 w1181 w1197 w1209 w1241 w1246 w1247 w1258 w1266 w1304 w1326 w1331 w1341 w1361 w1370 w1382 w1393 w1410 w1422 w1431 w1440 w1449 w1458 w1469 w1476 w1483 w1490 w1497 w1502 w1516 w1542 w1579 w1593 w1598 w1603]
      tunnel: w13 -> [w20 w588 w593 w604 w624 w637 w643 w658 w680 w687 w691 _ w721 w726 w743 w755 w766 w777 w790 w810 w828 w849 w890 w948 w975 w988 w1002 w1015 w1034 w1066 w1096 w1108 w1118 w1126 w1143 w1150 w1158 w1177 w1193 w1202 w1238 w1242 w1250 w1254 w1264 w1301 w1318 w1327 w1339 w1359 w1368 w1380 w1391 w1408 w1420 w1429 w1438 w1447 w1456 w1467 w1474 w1481 w1488 w1495 w1498 w1514 w1541 w1580 w1589 w1594 w1599]
      tunnel: [w20 w588 w593 w604 w624 w637 w643 w658 w680 w687 w691 w717 w721 w726 w743 w755 w766 w777 w790 w810 w828 w849 w890 w948 w975 w988 w1002 w1015 w1034 w1066 w1096 w1108 w1118 w1126 w1143 w1150 w1158 w1177 w1193 w1202 w1238 w1242 w1250 w1254 w1264 w1301 w1318 w1327 w1339 w1359 w1368 w1380 w1391 w1408 w1420 w1429 w1438 w1447 w1456 w1467 w1474 w1481 w1488 w1495 w1498 w1514 w1541 w1580 w1589 w1594 w1599] -> w12
      tunnel: [w23 w587 w596 w614 w621 w636 w642 w655 w667 w684 w690 w716 w723 w727 w744 w754 w765 w776 w789 w809 w827 w837 w891 w944 w976 w989 w1003 w1016 w1035 w1058 w1095 w1109 w1119 w1127 w1142 w1149 w1156 w1178 w1194 w1204 w1239 w1243 w1248 w1255 w1260 w1289 w1319 w1328 w1332 w1353 w1363 w1372 w1385 w1400 w1416 w1427 w1432 w1445 w1452 w1466 w1473 w1480 w1484 w1492 w1499 w1507 w1537 w1577 w1590 w1595 w1600] -> w11
      tunnel: [w25 w589 w600 w613 w622 w639 w644 w653 w663 w683 w692 w697 w720 w728 w742 w747 w758 w770 w787 w798 w814 w847 w881 w945 w977 w990 w995 w1008 w1021 w1046 w1083 w1104 w1120 w1128 w1144 w1151 w1159 w1179 w1191 w1203 w1236 w1244 w1251 w1256 w1259 w1302 w1324 w1329 w1336 w1356 w1365 w1377 w1388 w1401 w1418 w1424 w1436 w1441 w1450 w1463 w1470 w1477 w1485 w1491 w1500 w1503 w1538 w1560 w1591 w1596 w1601] -> w8
      tunnel: w7 -> [_ _ _ _ _ _ _ _ _ _ _ _ _ _ w733 _ _ _ _ _ _ _ _ _ _ _ _ _ _ _ _ _ _ _ _ _ _ _ _ _ _ _ _ _ _ _ _ _ _ _ _ _ _ _ _ _ _ _ _ _ _ _ _ _ _ _ _ _ _ _ _]
      tunnel: w6 -> [w24 w589 w599 w613 w618 w639 w644 w653 w670 w685 w692 w696 w720 w728 w740 w750 w761 w772 w782 w806 w824 w834 w882 w940 w977 w990 w999 w1013 w1031 w1050 w1090 w1105 w1120 w1128 w1144 w1151 w1159 w1179 w1192 w1207 w1236 w1244 w1251 w1256 w1262 w1302 w1324 w1329 w1337 w1357 w1366 w1378 w1389 w1406 w1415 w1425 w1433 w1443 w1451 w1464 w1471 w1478 w1486 w1493 w1500 w1503 w1536 w1565 w1591 w1596 w1601]
      tunnel: w5 -> [w22 w587 w596 w607 w621 w636 w642 _ w668 w684 w690 w716 w723 w727 w744 w753 w764 w775 w788 w808 w826 w837 w891 w944 w976 w989 w1003 w1016 w1035 w1058 w1095 w1109 w1119 w1127 w1142 w1149 w1156 w1178 w1194 w1204 w1239 w1243 w1248 w1255 w1260 w1289 w1319 w1328 w1332 w1353 w1363 w1372 w1385 w1400 w1416 w1427 w1432 w1445 w1452 w1466 w1473 w1480 w1484 w1492 w1499 w1508 w1537 w1577 w1590 w1595 w1600]
      frame "", "Idle" {
        # "executes when the state queue is empty"
        n6 = event shown="[44] \"auto DAQ\": Value Change" {
          selector: w20 -> [_ _ _ _ _ _ _ _ _ _ _ _ _ _ _ _ _ _ _ _ _ _ _ _ _ _ _ _ _ _ _ _ _ _ _ _ _ w398 _ _ _ _ _ _ _ _ _ _ _ _ _ _ _]
          dyn-events: _ -> [_ _ _ _ _ _ _ _ _ _ _ _ _ _ _ _ _ _ _ _ _ _ _ _ _ _ _ _ _ _ _ _ _ _ _ _ _ _ _ _ _ _ _ _ _ _ _ _ _ _ _ _ _]
          timeout: w21 -> [_ _ _ _ _ _ _ _ _ _ _ _ _ _ _ _ _ _ _ _ _ _ _ _ _ _ _ _ _ _ _ _ _ _ _ _ _ _ _ _ _ _ _ _ _ _ _ _ _ _ _ _ _]
          tunnel: w27 -> [w35 w61 w96 w105 w114 w121 w127 w133 w148 w155 w162 w175 w180 w190 w196 w204 w213 w228 w255 w270 w283 w285 w298 w307 w311 w316 w321 w326 w331 w336 w341 w346 w351 w356 w361 w366 w375 w405 w453 w465 w475 w482 w490 w498 w505 w512 w518 w538 w547 w556 w565 w571 w578]
          tunnel: [w33 w60 w95 w104 w113 w120 w126 w132 w147 w154 w163 w176 w181 w189 w195 w205 w214 w229 w254 w269 w282 w286 w297 w306 w312 w317 w322 w327 w332 w337 w342 w347 w352 w357 w362 w367 w374 w404 w452 w464 w474 w481 w489 w497 w504 w511 w517 w537 w546 w555 w564 w570 w582] -> w26
          tunnel: [w30 w46 w91 w100 w111 w118 w124 w130 w142 w151 w159 w167 w177 w182 w194 w198 w206 w218 w251 w263 w276 w287 w296 w305 w309 w314 w319 w324 w329 w334 w339 w344 w349 w354 w359 w364 w373 w399 w451 w462 w472 w479 w487 w495 w502 w509 w516 w523 w545 w553 w562 w567 w581] -> w25
          tunnel: w24 -> [w30 w48 w91 w100 w111 w118 w124 w130 w142 w151 w159 w167 w177 w182 w194 w198 w206 w218 w243 w258 w276 w287 w296 w305 w309 w314 w319 w324 w329 w334 w339 w344 w349 w354 w359 w364 w373 w400 w451 w462 w472 w479 w487 w495 w502 w509 w516 w536 w545 w553 w562 w568 w581]
          tunnel: [w34 w59 w93 w102 w106 w119 w125 w128 w149 w156 w160 w173 w178 w188 w193 w203 w212 w226 w253 w267 w280 w288 w294 w303 w310 w315 w320 w325 w330 w335 w340 w345 w350 w355 w360 w365 w372 w403 w450 w463 w473 w480 w488 w496 w503 w510 w515 w527 w544 w554 w563 w569 w580] -> w23
          tunnel: w22 -> [w34 w58 w92 w101 w107 w119 w125 w128 w150 w156 w160 w172 w178 w187 w193 w201 w210 w223 w252 w266 w279 w288 w294 w303 w310 w315 w320 w325 w330 w335 w340 w345 w350 w355 w360 w365 w371 w402 w450 w463 w473 w480 w488 w496 w503 w510 w515 w527 w544 w554 w563 w569 w580]
          event Timeout {
            n7 = event-data() -> ()  [unwired: 1 in, 1 out]
            n8 = Unbundle By Name(w34) -> ("Lockin"=w29:refnum<class "Instrument.Lockin.lvclass">)
            n9 = Unbundle By Name(w29) -> ("DAQ state"=w28:T32)
            n10 = case shown="\"created\"" w28 {
              tunnel: [w38 w42 w44] -> w32
              frame "idle" {
                n11 = call "Spinner.vi"("Enum"=enum16{"Spinner 1", "Spinner 2", "Spinner 3"}."Spinner 1") -> ("Spinner Out"=w36:string)  [unwired: 4 in]
                n12 = Concatenate Strings("Idle     " ("Status"), w36) -> (w38:string)
              }
              frame "created" {
                n13 = call "Spinner.vi"("Enum"=enum16{"Spinner 1", "Spinner 2", "Spinner 3"}."Spinner 1") -> ("Spinner Out"=w40:string)  [unwired: 4 in]
                n14 = Concatenate Strings("Created  " ("Status"), w40) -> (w42:string)
              }
              frame Default {
                n15 = local read "Status"() -> (w44:string)
              }
            }
            "Status" <- w32
            n16 = call <vilib>:"Add State(s) to Queue__jki_lib_state_machine.vi"("State(s) in Front (\"\")"="" ("t"), "State(s) in (\"\")"=w35) -> ("States Out"=w33:string)  [unwired: 13 in]
          }
          event User Event {
            n17 = event-data() -> ("AO"=w56:waveform(dbl)[], "AI"=w52:waveform(dbl)[], "RefX"=w55:waveform(dbl)[], "RefY"=w54:waveform(dbl)[])  [unwired: 1 in]
            n18 = call <userlib>:"MGI Milliseconds Since Last Call.vi"("Error In"=w48) -> ("ms"=w45:u32, "Error Out"=w47:errorcluster)  [unwired: 5 in]
            "Refresh time (ms)" <- w45
            n19 = disable-structure shown="Enabled" {
              disable-tunnel: w47 -> [w78 w86]
              disable-tunnel: [w77 w86] -> w46
              disable-tunnel: w52 -> [w70 _]
              disable-tunnel: w45 -> [w69 _]
              frame Enabled {
                n20 = Index Array(array=w70) -> (element=w85:waveform(dbl))  [unwired: 1 in]
                n21 = call-poly <vilib>:"Waveform Duration.vi"("error in (no error)"=w78, "waveform in"=w85) -> ("error out"=w77:errorcluster, "duration"=w84:dbl)  [unwired: 7 in, 1 out]
                n22 = Multiply(x=w84, y=1000.0) -> (x*y=w75:dbl)
                n23 = Multiply(x=w75, y=2.0) -> (x*y=w74:dbl)
                n24 = Less?(x=w69, y=w74) -> (x < y?=w72:bool)
                n25 = Select(t="Good", s=w72, f="#s/Fs: too small!") -> (s? t:f=→"Sampling Status":string)
                n26 = Select(t=u32 6618880, s=w72, f=u32 16711680) -> (s? t:f=w82:u32)
                n27 = property on="Sampling Status" class="Str"("Text.BGColor"=w82) -> ()  [unwired: 2 in, 2 out]
              }
              frame Disabled {
              }
            }
            n28 = Unbundle By Name(w58) -> ("Lockin"=w57:refnum<class "Instrument.Lockin.lvclass">)
            n29 = Bundle By Name(cluster=w57, "AO"=w56, "AI"=w52, "RefX"=w55, "RefY"=w54) -> (w53:refnum<class "Instrument.Lockin.lvclass">)
            n30 = call <userlib>:"Periodic Trigger__ogtk.vi"("time (ms)"=u32 100) -> ("Triggered"=w50:bool)  [unwired: 12 in, 2 out]
            n31 = case shown="True" w50 {
              tunnel: ["" ("State(s) in Front (\"\")") w65] -> w49
              frame False {
              }
              frame True {
                n32 = local read "Tab Control 2"() -> (w66:T20)
                n33 = case shown="\"PS\"" w66 {
                  tunnel: ["" ("State(s) in Front (\"\")") "4461: FFT" ("State(s) in Front (\"\")")] -> w64
                  frame Default {
                  }
                  frame "PS" {
                  }
                }
                n34 = call <vilib>:"Add State(s) to Queue__jki_lib_state_machine.vi"("State(s) in Front (\"\")"="4461: OUT\nUI: Update Waveform Graphs\nUI: Sync AO AI Plot Visibility\nUI: Update Lockin Graphs\nUI: Sync Lockin Plot Visibility\nUI: Update Sweep Timer" ("State(s) in Front (\"\")"), "State(s) at Back (\"\")"=w64) -> ("States Out"=w65:string)  [unwired: 13 in]
              }
            }
            n35 = Bundle By Name(cluster=w58, "Lockin"=w53) -> (w59:T36)
            n36 = call <vilib>:"Add State(s) to Queue__jki_lib_state_machine.vi"("State(s) in Front (\"\")"=w49, "State(s) in (\"\")"=w61) -> ("States Out"=w60:string)  [unwired: 13 in]
          }
          event User Event {
            n37 = event-data() -> ("Sweep AO"=w90:waveform(dbl)[], "Sweep AI"=w87:waveform(dbl)[], "Sweep Results X"=w88:waveform(dbl)[], "Sweep Results Y"=w89:waveform(dbl)[])  [unwired: 1 in]
            n38 = Bundle By Name(cluster=w92, "SweepWaveforms.Sweep AO"=w90, "SweepWaveforms.Sweep AI"=w87, "SweepWaveforms.Sweep Results X"=w88, "SweepWaveforms.Sweep Results Y"=w89) -> (w93:T36)
            n39 = call <vilib>:"Add State(s) to Queue__jki_lib_state_machine.vi"("State(s) in Front (\"\")"="UI: Update Sweep WFMs Graphs" ("State(s) in Front (\"\")"), "State(s) in (\"\")"=w96) -> ("States Out"=w95:string)  [unwired: 13 in]
          }
          event User Event {
            n40 = event-data() -> ("AO"=w97:waveform(dbl)[])  [unwired: 1 in, 4 out]
            n41 = Unbundle By Name(w101) -> ("Lockin"=w99:refnum<class "Instrument.Lockin.lvclass">)
            n42 = Bundle By Name(cluster=w99, "AO"=w97) -> (w98:refnum<class "Instrument.Lockin.lvclass">)
            n43 = local write "AO Channels"(w97) -> ()
            n44 = Bundle By Name(cluster=w101, "Lockin"=w98) -> (w102:T36)
            n45 = call <vilib>:"Add State(s) to Queue__jki_lib_state_machine.vi"("State(s) in Front (\"\")"="" ("State(s) in Front (\"\")"), "State(s) in (\"\")"=w105) -> ("States Out"=w104:string)  [unwired: 13 in]
          }
          event User Event {
            n46 = event-data() -> ("state"=w108:T37)  [unwired: 1 in, 4 out]
            n47 = case shown="Default" w108 {
              frame Default {
              }
              frame "sweeping" {
                n48 = call <userlib>:"MGI Milliseconds Since Last Reset.vi"("Reset (F)"=TRUE) -> ()  [unwired: 5 in, 2 out]
              }
            }
            n49 = Unbundle By Name(w107) -> ("Lockin"=w110:refnum<class "Instrument.Lockin.lvclass">)
            n50 = Bundle By Name(cluster=w110, "DAQ state"=w108) -> (w109:refnum<class "Instrument.Lockin.lvclass">)
            n51 = Bundle By Name(cluster=w107, "Lockin"=w109) -> (w106:T36)
            n52 = call <vilib>:"Add State(s) to Queue__jki_lib_state_machine.vi"("State(s) in Front (\"\")"="UI: Update Status" ("State(s) in Front (\"\")"), "State(s) in (\"\")"=w114) -> ("States Out"=w113:string)  [unwired: 13 in]
          }
          event User Event {
            # "Check Calibrate Mode Button Value Change (pressed) Event"
            n53 = event-data() -> ("Channels: REF"=→"Cal Info":T38)  [unwired: 1 in]
            n54 = call <vilib>:"Add State(s) to Queue__jki_lib_state_machine.vi"("State(s) in (\"\")"=w121, "State(s) at Back (\"\")"="" ("State(s) at Back (\"\")")) -> ("States Out"=w120:string)  [unwired: 13 in]
          }
          event User Event {
            # "Check Calibrate Mode Button Value Change (pressed) Event"
            n55 = event-data() -> ("New Ch []"=w122:T39)  [unwired: 1 in]
            n56 = property on="DAQ Config" class="Arr (strict)"("Val(Sgnl)"=w122) -> ()  [unwired: 2 in, 2 out]
            n57 = call <vilib>:"Add State(s) to Queue__jki_lib_state_machine.vi"("State(s) in (\"\")"=w127, "State(s) at Back (\"\")"="" ("State(s) at Back (\"\")")) -> ("States Out"=w126:string)  [unwired: 13 in]
          }
          event User Event {
            # "#framework\n????"
            n58 = event-data() -> ("SMO State"=w129:T16)  [unwired: 1 in]
            "LockinDAQ SMO State" <- w129
            n59 = case shown="\"Started\"" w129 {
              tunnel: ["UI: Enable Buttons" ("State Queue") "" ("State Queue")] -> w131
              frame "Started" {
              }
              frame Default {
              }
            }
            n60 = call <vilib>:"Add State(s) to Queue__jki_lib_state_machine.vi"("State(s) in Front (\"\")"=w131, "State(s) in (\"\")"=w133) -> ("States Out"=w132:string)  [unwired: 13 in]
          }
          event User Event {
            # "#framework"
            # "here command should be argument?"
            # "#todo: future: call Command: Handle Command"
            # "Message sent by the RemoteControl.lvclass:process"
            n61 = event-data() -> ("Message"=w143:T34, "Message.Command"=w139:string)  [unwired: 1 in, 3 out]
            n62 = Concatenate Strings("Command: ", w139) -> (w138:string)
            n63 = call <userlib>:"MGI String Pattern Match Exists.vi"("Patterns to Try"=string[] ["getAOconfig", "getSampling", "getREFconfig", "getInputGain", "getOutputGain", "getAO", "getAI", "getResults", "getStatus", "getSweepResults", "getSweepWaveforms", "getAutoSampling", "getState", "setAO", "setAO_Amplitude", "setAO_DC", "setAO_Frequency", "setAO_Phase", "setAO_Function", "setREF", "setREF_Frequency", "setREF_Phase", "setREF_TC", "setREF_RollOff", "setSweepConfiguration", "setState", "setSampling", "setSamplingMode", "setInputGain", "setOutputGain", "setDAQ", "HELP", "ACK", "getAll"] ("Array"), "String"=w139) -> ("Match Found"=w141:bool)  [unwired: 1 out]
            n64 = Select(t="" ("State(s) in Front (\"\")"), s=w141, f=w138) -> (s? t:f=w136:string)
            n65 = Bundle By Name(cluster=w150, "Message"=w143) -> (w149:T36)
            n66 = call <vilib>:"Add State(s) to Queue__jki_lib_state_machine.vi"("State(s) in Front (\"\")"=w136, "State(s) at Back (\"\")"="") -> ("States Out"=w145:string)  [unwired: 13 in]
            n67 = call <vilib>:"Add State(s) to Queue__jki_lib_state_machine.vi"("State(s) in Front (\"\")"=w145, "State(s) in (\"\")"=w148) -> ("States Out"=w147:string)  [unwired: 13 in]
          }
          event User Event {
            # "Disable: I think this could cause an infinite loop when trying to exit"
            n68 = event-data() -> ("SMO State"=w152:T16)  [unwired: 1 in]
            "RC SMO State" <- w152
            n69 = case shown="\"Started\"" w152 {
              tunnel: ["" ("State Queue") "" ("State Queue")] -> w153
              frame "Started" {
              }
              frame Default {
              }
            }
            n70 = call <vilib>:"Add State(s) to Queue__jki_lib_state_machine.vi"("State(s) in Front (\"\")"=w153, "State(s) in (\"\")"=w155) -> ("States Out"=w154:string)  [unwired: 13 in]
          }
          event Value Change {
            n71 = event-data() -> ()  [unwired: 1 in, 6 out]
            n72 = call <vilib>:"Add State(s) to Queue__jki_lib_state_machine.vi"("State(s) in Front (\"\")"="" ("State(s) in Front (\"\")"), "State(s) in (\"\")"=w162) -> ("States Out"=w163:string)  [unwired: 13 in]
          }
          event "DAQ Config": Value Change {
            w170 = -1 items=["Default"=-1, "RSE"=10083, "Differential"=10106, "Pseudodifferential"=12529] ("output terminal configuration")
            w171 = -1 items=["Default"=-1, "RSE"=10083, "NRSE"=10078, "Differential"=10106, "Pseudodifferential"=12529] ("input terminal configuration")
            n73 = event-data() -> ("NewVal"=w169:T6[])  [unwired: 1 in]
            n74 = Unbundle By Name(w172) -> ("Lockin"=w168:refnum<class "Instrument.Lockin.lvclass">)
            n75 = call "config UI to not UI (AO and AI).vi"("output terminal configuration"=w170, "input terminal configuration"=w171, "New Ch []"=w169) -> ("AO Config"=w164:T44, "AI Config"=w165:T46)  [unwired: 7 in]
            n76 = Bundle By Name(cluster=w168, "AI"=w165, "AO"=w164) -> (w166:refnum<class "Instrument.Lockin.lvclass">)
            n77 = Bundle By Name(cluster=w172, "Lockin"=w166) -> (w173:T36)
            n78 = call <vilib>:"Add State(s) to Queue__jki_lib_state_machine.vi"("State(s) in Front (\"\")"="Lockin SMO: Set AO Config\nLockin SMO: Set AI Config\nUI: Initialize REF Ch\nUI: Initialize AO Ch\nUI: Update AI Ch\nUI: Initialize Gains\nUI: Update Plot Names" ("State(s) in Front (\"\")"), "State(s) in (\"\")"=w175) -> ("States Out"=w176:string)  [unwired: 13 in]
          }
          event Value Change {
            n79 = event-data() -> ()  [unwired: 1 in, 1 out]
            n80 = call <vilib>:"Add State(s) to Queue__jki_lib_state_machine.vi"("State(s) in Front (\"\")"="Lockin SMO: Set AI Config" ("State(s) in Front (\"\")"), "State(s) in (\"\")"=w180) -> ("States Out"=w181:string)  [unwired: 13 in]
          }
          event Value Change {
            n81 = event-data() -> ("NewVal"=w183:T11)  [unwired: 1 in, 1 out]
            n82 = Unbundle By Name(w187) -> ("Lockin"=w185:refnum<class "Instrument.Lockin.lvclass">)
            n83 = Bundle By Name(cluster=w185, "Sampling"=w183) -> (w184:refnum<class "Instrument.Lockin.lvclass">)
            n84 = Bundle By Name(cluster=w187, "Lockin"=w184) -> (w188:T36)
            n85 = call <vilib>:"Add State(s) to Queue__jki_lib_state_machine.vi"("State(s) in Front (\"\")"="Macro: Update Sampling" ("State(s) in Front (\"\")"), "State(s) in (\"\")"=w190) -> ("States Out"=w189:string)  [unwired: 13 in]
          }
          event "Auto x*F1", "Max Fs Refresh Rate (Hz)", "decimating factor": Value Change {
            n86 = event-data() -> ()  [unwired: 1 in, 6 out]
            n87 = call <vilib>:"Add State(s) to Queue__jki_lib_state_machine.vi"("State(s) in Front (\"\")"="Macro: Update Sampling" ("State(s) in Front (\"\")")) -> ("States Out"=w192:string)  [unwired: 14 in]
            n88 = call <vilib>:"Add State(s) to Queue__jki_lib_state_machine.vi"("State(s) in Front (\"\")"=w192, "State(s) in (\"\")"=w196) -> ("States Out"=w195:string)  [unwired: 13 in]
          }
          event "AO Channels": Value Change {
            n89 = event-data() -> ("NewVal"=w197:T4)  [unwired: 1 in, 5 out]
            n90 = Unbundle By Name(w201) -> ("Lockin"=w200:refnum<class "Instrument.Lockin.lvclass">)
            n91 = Bundle By Name(cluster=w200, "AO"=w197) -> (w199:refnum<class "Instrument.Lockin.lvclass">)
            n92 = Bundle By Name(cluster=w201, "Lockin"=w199) -> (w203:T36)
            n93 = call <vilib>:"Add State(s) to Queue__jki_lib_state_machine.vi"("State(s) in Front (\"\")"="Data: Adjust Channels\nUI: Update Rings\nLockin SMO: Set AO" ("f"), "State(s) in (\"\")"=w204) -> ("States Out"=w205:string)  [unwired: 13 in]
          }
          event "AI Channels": Value Change {
            n94 = event-data() -> ("NewVal"=w207:T2)  [unwired: 1 in]
            n95 = Unbundle By Name(w210) -> ("Lockin"=w209:refnum<class "Instrument.Lockin.lvclass">)
            n96 = Bundle By Name(cluster=w209, "AI"=w207) -> (w208:refnum<class "Instrument.Lockin.lvclass">)
            n97 = Bundle By Name(cluster=w210, "Lockin"=w208) -> (w212:T36)
            n98 = call <vilib>:"Add State(s) to Queue__jki_lib_state_machine.vi"("State(s) in Front (\"\")"="UI: Update Rings\nLockin SMO: Set AI" ("f"), "State(s) in (\"\")"=w213) -> ("States Out"=w214:string)  [unwired: 13 in]
          }
          event "REF Channels": Value Change {
            # "#todo\nthis \"macro\" needs to\nbe handled by Lockin.DAQ\nor Handle Command"
            # "if number of lockin channels is not the same as before reset the lockin\nupdate: no, just reset phase...?"
            n99 = event-data() -> ("NewVal"=w215:T5[], "OldVal"=w220:T5[])  [unwired: 1 in]
            n100 = Unbundle By Name(w223) -> ("Lockin"=w217:refnum<class "Instrument.Lockin.lvclass">)
            n101 = Bundle By Name(cluster=w217, "REF"=w215) -> (w216:refnum<class "Instrument.Lockin.lvclass">)
            n102 = Not Equal?(x=w215, y=w220) -> (x != y?=w221:bool)
            n103 = Unbundle By Name(w216) -> ("DAQ state"=w219:T32)
            n104 = case shown="\"created\"" w219 {
              tunnel: ["" ("f") w237] -> _
              tunnel: w221 -> [_ w236]
              frame "idle", Default {
              }
              frame "created" {
                n105 = Format Into String(Set_State-enum."start" ("State")) -> (resulting string=w239:string)  [unwired: 3 in, 1 out]
                n106 = call <vilib>:"Build State String with Arguments__JKI_lib_State_Machine.vi"("Arguments (\"\")"=w239, "State"="Lockin SMO: Set State" ("f")) -> ("State with Arguments"=w242:string)  [unwired: 4 in]
                n107 = Select(t=w242, s=w236, f="") -> (s? t:f=w237:string)
              }
            }
            n108 = case shown="\"created\"" w219 {
              tunnel: ["" ("State with Arguments") w231] -> w224
              frame "idle", Default {
              }
              frame "created" {
                n109 = Format Into String(Set_State-enum."stop" ("State")) -> (resulting string=w234:string)  [unwired: 3 in, 1 out]
                n110 = call <vilib>:"Build State String with Arguments__JKI_lib_State_Machine.vi"("Arguments (\"\")"=w234, "State"="Lockin SMO: Set State" ("f")) -> ("State with Arguments"=w231:string)  [unwired: 4 in]
              }
            }
            n111 = Bundle By Name(cluster=w223, "Lockin"=w216) -> (w226:T36)
            n112 = Select(t=w224, s=w221, f="") -> ()  [unwired: 1 out]
            n113 = call <vilib>:"Add State(s) to Queue__jki_lib_state_machine.vi"("State(s) in (\"\")"="Data: Adjust Channels\nUI: Update Rings\nUI: Update Plot Names\nLockin SMO: Set REF\nLockin SMO: Reset Phase" ("f")) -> ("States Out"=w225:string)  [unwired: 14 in]
            n114 = call <vilib>:"Add State(s) to Queue__jki_lib_state_machine.vi"("State(s) in Front (\"\")"=w225, "State(s) in (\"\")"=w228) -> ("States Out"=w229:string)  [unwired: 13 in]
          }
          event "Input Gain": Value Change {
            n115 = event-data() -> ("NewVal"=w249:cluster{"AI.Ch":string, "Gain":dbl}[])  [unwired: 1 in, 5 out]
            n116 = for {
              tunnel: w249 -> [w257] mode=indexing
              tunnel: [w256] -> w246 mode=indexing
              n117 = Unbundle(w257) -> ("Gain"=w256:dbl)  [unwired: 1 out]
            }
            n118 = Unbundle By Name(w252) -> ("Lockin"=w245:refnum<class "Instrument.Lockin.lvclass">)
            n119 = Bundle By Name(cluster=w245, "Input Gain"=w246) -> (w244:refnum<class "Instrument.Lockin.lvclass">)
            n120 = call "Initialize Input Gain.vi"("error in (no error)"=w243, "Instrument.Lockin"=w244) -> ("error out"=w251:errorcluster, "Input Gain"=w248:cluster{string, "Gain":dbl}[], "Instrument.Lockin out"=w250:refnum<class "Instrument.Lockin.lvclass">)  [unwired: 7 in]
            n121 = local write "Input Gain"(w248) -> ()
            n122 = Bundle By Name(cluster=w252, "Lockin"=w250) -> (w253:T36)
            n123 = call <vilib>:"Add State(s) to Queue__jki_lib_state_machine.vi"("State(s) in Front (\"\")"="Lockin SMO: Set Input Gain" ("State(s) in Front (\"\")"), "State(s) in (\"\")"=w255) -> ("States Out"=w254:string)  [unwired: 13 in]
          }
          event "Output Gain": Value Change {
            n124 = event-data() -> ("NewVal"=w265:cluster{"AI.Ch":string, "Gain":dbl}[])  [unwired: 1 in, 5 out]
            n125 = for {
              tunnel: w265 -> [w272] mode=indexing
              tunnel: [w271] -> w260 mode=indexing
              n126 = Unbundle(w272) -> ("Gain"=w271:dbl)  [unwired: 1 out]
            }
            n127 = Unbundle By Name(w266) -> ("Lockin"=w261:refnum<class "Instrument.Lockin.lvclass">)
            n128 = Bundle By Name(cluster=w261, "Output Gain"=w260) -> (w259:refnum<class "Instrument.Lockin.lvclass">)
            n129 = call "Initialize Ouput Gain.vi"("error in (no error)"=w258, "Instrument.Lockin"=w259) -> ("error out"=w263:errorcluster, "Ouput Gain"=w262:cluster{string, "Gain":dbl}[], "Instrument.Lockin out"=w264:refnum<class "Instrument.Lockin.lvclass">)  [unwired: 7 in]
            n130 = local write "Output Gain"(w262) -> ()
            n131 = Bundle By Name(cluster=w266, "Lockin"=w264) -> (w267:T36)
            n132 = call <vilib>:"Add State(s) to Queue__jki_lib_state_machine.vi"("State(s) in Front (\"\")"="Lockin SMO: Set Output Gain" ("State(s) in Front (\"\")"), "State(s) in (\"\")"=w270) -> ("States Out"=w269:string)  [unwired: 13 in]
          }
          event "Line", "Lowpass", "LP f (Hz)": Value Change {
            n133 = event-data() -> ()  [unwired: 1 in, 6 out]
            n134 = Unbundle By Name(w279) -> ("Lockin"=w278:refnum<class "Instrument.Lockin.lvclass">)
            n135 = Bundle By Name(cluster=w278, "60 Hz"="Line", "Low Pass"="Lowpass", "Low Pass Cutoff (Hz)"="LP f (Hz)") -> (w277:refnum<class "Instrument.Lockin.lvclass">)
            n136 = Bundle By Name(cluster=w279, "Lockin"=w277) -> (w280:T36)
            n137 = call <vilib>:"Add State(s) to Queue__jki_lib_state_machine.vi"("State(s) in Front (\"\")"="Lockin SMO: Set Prefilter" ("State(s) in Front (\"\")"), "State(s) in (\"\")"=w283) -> ("States Out"=w282:string)  [unwired: 13 in]
          }
          event "Allowed remote system": Value Change {
            n138 = event-data() -> ()  [unwired: 1 in, 6 out]
            n139 = call <vilib>:"Add State(s) to Queue__jki_lib_state_machine.vi"("State(s) in Front (\"\")"="" ("State(s) in Front (\"\")"), "State(s) in (\"\")"=w285) -> ("States Out"=w286:string)  [unwired: 13 in]
          }
          event "Self Calibrate": Value Change {
            # "Self Calibrate Mode Button Value Change (pressed) Event"
            n140 = event-data() -> ()  [unwired: 1 in, 2 out]
            n141 = local write "Self Calibrate"(FALSE ("Self Calibrate")) -> ()
            n142 = property on="Pause" class="Bool (strict)"("Val(Sgnl)"=TRUE ("Value (Signaling)")) -> ()  [unwired: 2 in, 2 out]
            n143 = Format Into String(PrivateEvents--DAQ.setCalibration."Calibrate" ("setCalibration")) -> (resulting string=w289:string)  [unwired: 3 in, 1 out]
            n144 = call <vilib>:"Build State String with Arguments__JKI_lib_State_Machine.vi"("Arguments (\"\")"=w289, "State"="Lockin SMO: Calibration" ("f")) -> ("State with Arguments"=w291:string)  [unwired: 4 in]
            n145 = call <vilib>:"Add State(s) to Queue__jki_lib_state_machine.vi"("State(s) in Front (\"\")"=w291, "State(s) in (\"\")"=w298) -> ("States Out"=w297:string)  [unwired: 13 in]
          }
          event "Get Calibration": Value Change {
            # "Self Calibrate Mode Button Value Change (pressed) Event"
            n146 = event-data() -> ()  [unwired: 1 in, 2 out]
            n147 = local write "Get Calibration"(FALSE ("Self Calibrate")) -> ()
            n148 = Format Into String(PrivateEvents--DAQ.setCalibration."Check" ("setCalibration")) -> (resulting string=w301:string)  [unwired: 3 in, 1 out]
            n149 = call <vilib>:"Build State String with Arguments__JKI_lib_State_Machine.vi"("Arguments (\"\")"=w301, "State"="Lockin SMO: Calibration" ("f")) -> ("State with Arguments"=w299:string)  [unwired: 4 in]
            n150 = call <vilib>:"Add State(s) to Queue__jki_lib_state_machine.vi"("State(s) in Front (\"\")"=w299, "State(s) in (\"\")"=w307) -> ("States Out"=w306:string)  [unwired: 13 in]
          }
          event "X Axis": Value Change {
            # "X Axis, Y Axis Out Value Change (pressed) Event\ncall: UI: Update Waveform Graph Labels"
            n151 = event-data() -> ()  [unwired: 1 in, 6 out]
            n152 = call <vilib>:"Add State(s) to Queue__jki_lib_state_machine.vi"("State(s) in Front (\"\")"="UI: Update Waveform Graph Labels" ("State(s) in Front (\"\")"), "State(s) in (\"\")"=w311) -> ("States Out"=w312:string)  [unwired: 13 in]
          }
          event "Y Axis (Output)": Value Change {
            # "X Axis, Y Axis Out Value Change (pressed) Event\ncall: UI: Update Waveform Graph Labels"
            n153 = event-data() -> ()  [unwired: 1 in, 6 out]
            n154 = call <vilib>:"Add State(s) to Queue__jki_lib_state_machine.vi"("State(s) in Front (\"\")"="UI: Update Plot Names" ("State(s) in Front (\"\")"), "State(s) in (\"\")"=w316) -> ("States Out"=w317:string)  [unwired: 13 in]
          }
          event "AI Graph All": Value Change {
            # "X Axis, Y Axis Out Value Change (pressed) Event\ncall: UI: Update Waveform Graph Labels"
            n155 = event-data() -> ()  [unwired: 1 in, 6 out]
            n156 = call <vilib>:"Add State(s) to Queue__jki_lib_state_machine.vi"("State(s) in Front (\"\")"="UI: AI Graph Plot Visible >> All" ("State(s) in Front (\"\")"), "State(s) in (\"\")"=w321) -> ("States Out"=w322:string)  [unwired: 13 in]
          }
          event "AI Graph None": Value Change {
            # "X Axis, Y Axis Out Value Change (pressed) Event\ncall: UI: Update Waveform Graph Labels"
            n157 = event-data() -> ()  [unwired: 1 in, 6 out]
            n158 = call <vilib>:"Add State(s) to Queue__jki_lib_state_machine.vi"("State(s) in Front (\"\")"="UI: AI Graph Plot Visible >> None" ("State(s) in Front (\"\")"), "State(s) in (\"\")"=w326) -> ("States Out"=w327:string)  [unwired: 13 in]
          }
          event "AO Graph All": Value Change {
            # "X Axis, Y Axis Out Value Change (pressed) Event\ncall: UI: Update Waveform Graph Labels"
            n159 = event-data() -> ()  [unwired: 1 in, 6 out]
            n160 = call <vilib>:"Add State(s) to Queue__jki_lib_state_machine.vi"("State(s) in Front (\"\")"="UI: AO Graph Plot Visible >> All" ("State(s) in Front (\"\")"), "State(s) in (\"\")"=w331) -> ("States Out"=w332:string)  [unwired: 13 in]
          }
          event "AO Graph None": Value Change {
            # "X Axis, Y Axis Out Value Change (pressed) Event\ncall: UI: Update Waveform Graph Labels"
            n161 = event-data() -> ()  [unwired: 1 in, 6 out]
            n162 = call <vilib>:"Add State(s) to Queue__jki_lib_state_machine.vi"("State(s) in Front (\"\")"="UI: AO Graph Plot Visible >> None" ("State(s) in Front (\"\")"), "State(s) in (\"\")"=w336) -> ("States Out"=w337:string)  [unwired: 13 in]
          }
          event "Lockin 1 All": Value Change {
            # "X Axis, Y Axis Out Value Change (pressed) Event\ncall: UI: Update Waveform Graph Labels"
            n163 = event-data() -> ()  [unwired: 1 in, 6 out]
            n164 = call <vilib>:"Add State(s) to Queue__jki_lib_state_machine.vi"("State(s) in Front (\"\")"="UI: Lockin 1 Plot Visible >> All" ("State(s) in Front (\"\")"), "State(s) in (\"\")"=w341) -> ("States Out"=w342:string)  [unwired: 13 in]
          }
          event "Lockin 1 None": Value Change {
            # "X Axis, Y Axis Out Value Change (pressed) Event\ncall: UI: Update Waveform Graph Labels"
            n165 = event-data() -> ()  [unwired: 1 in, 6 out]
            n166 = call <vilib>:"Add State(s) to Queue__jki_lib_state_machine.vi"("State(s) in Front (\"\")"="UI: Lockin 1 Plot Visible >> None" ("State(s) in Front (\"\")"), "State(s) in (\"\")"=w346) -> ("States Out"=w347:string)  [unwired: 13 in]
          }
          event "Update": Value Change {
            # "Update Value Change (pressed) Event\ncall: AUX: Set AUX"
            n167 = event-data() -> ()  [unwired: 1 in, 6 out]
            n168 = call <vilib>:"Add State(s) to Queue__jki_lib_state_machine.vi"("State(s) in Front (\"\")"="" ("State(s) in Front (\"\")"), "State(s) in (\"\")"=w351) -> ("States Out"=w352:string)  [unwired: 13 in]
          }
          event "Numeric", "X/R Range", "Y/Theta Range": Value Change {
            # "X&Y Axis Range\", \"XorR Axis Range\", \"YorTheta Axis Range\" Value Change (pressed) Event\ncall: UI: Update Lockin Graph Range"
            n169 = event-data() -> ()  [unwired: 1 in, 6 out]
            n170 = call <vilib>:"Add State(s) to Queue__jki_lib_state_machine.vi"("State(s) in Front (\"\")"="UI: Update Lockin Graph Range" ("State(s) in Front (\"\")"), "State(s) in (\"\")"=w356) -> ("States Out"=w357:string)  [unwired: 13 in]
          }
          event "Link Frequencies", "Limit Amplitudes", "AO freq link": Value Change {
            # "Same f\", \"Limit Amp\", \"AO freq link\": Value Change Value Change (pressed) Event\ncall:\nData: Adjust Channels\nConfiguration: Write\nLockin SMO: Set AO\nLockin SMO: Set REF"
            n171 = event-data() -> ()  [unwired: 1 in, 6 out]
            n172 = call <vilib>:"Add State(s) to Queue__jki_lib_state_machine.vi"("State(s) in Front (\"\")"="Data: Adjust Channels\nUI: Update Rings\nLockin SMO: Set AO\nLockin SMO: Set REF" ("f"), "State(s) in (\"\")"=w361) -> ("States Out"=w362:string)  [unwired: 13 in]
          }
          event Value Change {
            # "Display Value Change Value Change (pressed) Event\ncall:\nUI: Update Displays"
            n173 = event-data() -> ()  [unwired: 1 in, 6 out]
            n174 = call <vilib>:"Add State(s) to Queue__jki_lib_state_machine.vi"("State(s) in Front (\"\")"="UI: Update Displays" ("f"), "State(s) in (\"\")"=w366) -> ("States Out"=w367:string)  [unwired: 13 in]
          }
          event "Start": Value Change {
            # "Start Button Value Change (pressed) Event\nIf DAQ=idle:\n1. Set Sampling to Continuous Samples\n2. Start acquisition\n3. Set Pause=False\n4. Set timout=10\n\nIf DAQ=running:\n1. Do nothing"
            n175 = event-data() -> ()  [unwired: 1 in, 2 out]
            n176 = Unbundle By Name(w371) -> ("Lockin"=w369:refnum<class "Instrument.Lockin.lvclass">)
            n177 = Unbundle By Name(w369) -> ("DAQ state"=w368:T32)
            n178 = case shown="\"idle\", Default" w368 {
              tunnel: [w382 "" ("State with Arguments")] -> w370
              tunnel: w371 -> [w388 w394]
              tunnel: [w387 w394] -> w372
              frame "idle", Default {
                w383 = T48 10123 items=["Finite Samples"=10178, "Continuous Samples"=10123] ("Sample Mode")
                n179 = local write "Pause"(FALSE ("Pause")) -> ()
                n180 = Format Into String(w383) -> (resulting string=w384:string)  [unwired: 3 in, 1 out]
                n181 = Format Into String(Set_State-enum."start" ("State")) -> (resulting string=w392:string)  [unwired: 3 in, 1 out]
                n182 = First Call?() -> (First Call?: T/F=w379:bool)
                n183 = call <vilib>:"Build State String with Arguments__JKI_lib_State_Machine.vi"("Arguments (\"\")"=w384, "State"="Lockin SMO: Set Sampling" ("f")) -> ("State with Arguments"=w381:string)  [unwired: 4 in]
                n184 = call <vilib>:"Build State String with Arguments__JKI_lib_State_Machine.vi"("Arguments (\"\")"=w392, "State"="Lockin SMO: Set State" ("f")) -> ("State with Arguments"=w380:string)  [unwired: 4 in]
                n185 = Select(t="Macro: Update Sampling" ("f"), s=w379, f="") -> (s? t:f=w377:string)
                n186 = call <vilib>:"Add State(s) to Queue__jki_lib_state_machine.vi"("State(s) in Front (\"\")"=w377, "State(s) in (\"\")"=w381, "State(s) at Back (\"\")"=w380) -> ("States Out"=w382:string)  [unwired: 12 in]
                n187 = Bundle By Name(cluster=w388, "to"=-1) -> (w387:T36)
              }
              frame "created" {
              }
            }
            n188 = call <vilib>:"Add State(s) to Queue__jki_lib_state_machine.vi"("State(s) in (\"\")"=w375, "State(s) at Back (\"\")"=w370) -> ("States Out"=w374:string)  [unwired: 13 in]
          }
          event "Pause": Value Change {
            # "Pause Button Value Change (pressed) Event\nPause=True & DAQ=running:\n1. Set Sampling to Finite Samples\n2. STOP acquisition\n3. Set timeout=-1 (wait forever)\nPause=True & DAQ=idle\n1. Set timeout=-1\n2. Set Sampling to Finite\nPause=False:\n1. send T=Val(Sgnl) to Start"
            n189 = event-data() -> ("NewVal"=w401:bool)  [unwired: 1 in]
            n190 = Unbundle By Name(w402) -> ("Lockin"=w396:refnum<class "Instrument.Lockin.lvclass">)
            n191 = Unbundle By Name(w396) -> ("DAQ state"=w395:T32)
            n192 = Flush Event Queue(0:w398, 3:w400) -> (11:w399:errorcluster)  [unwired: 4 in, 2 out]
            n193 = case shown="True" w401 {
              tunnel: [w407 "" ("States Out")] -> w397
              tunnel: w402 -> [w409 w435]
              tunnel: [w408 w435] -> w403
              tunnel: w395 -> [w406 _]
              frame True {
                n194 = case shown="\"started\"" w406 {
                  tunnel: w409 -> [w414 w430]
                  tunnel: [w413 w429] -> w408
                  tunnel: [w410 w420] -> w407
                  frame "idle", Default {
                    w416 = T48 10178 items=["Finite Samples"=10178, "Continuous Samples"=10123] ("Sample Mode")
                    n195 = Format Into String(w416) -> (resulting string=w417:string)  [unwired: 3 in, 1 out]
                    n196 = call <vilib>:"Build State String with Arguments__JKI_lib_State_Machine.vi"("Arguments (\"\")"=w417, "State"="Lockin SMO: Set Sampling" ("f")) -> ("State with Arguments"=w411:string)  [unwired: 4 in]
                    n197 = call <vilib>:"Add State(s) to Queue__jki_lib_state_machine.vi"("State(s) at Back (\"\")"=w411) -> ("States Out"=w410:string)  [unwired: 14 in]
                    n198 = Bundle By Name(cluster=w414, "to"=100) -> (w413:T36)
                  }
                  frame "started" {
                    w425 = T48 10178 items=["Finite Samples"=10178, "Continuous Samples"=10123] ("Sample Mode")
                    n199 = Format Into String(Set_State-enum."stop" ("State")) -> (resulting string=w433:string)  [unwired: 3 in, 1 out]
                    n200 = Format Into String(w425) -> (resulting string=w426:string)  [unwired: 3 in, 1 out]
                    n201 = call <vilib>:"Build State String with Arguments__JKI_lib_State_Machine.vi"("Arguments (\"\")"=w433, "State"="Lockin SMO: Set State" ("f")) -> ("State with Arguments"=w418:string)  [unwired: 4 in]
                    n202 = call <vilib>:"Build State String with Arguments__JKI_lib_State_Machine.vi"("Arguments (\"\")"=w426, "State"="Lockin SMO: Set Sampling" ("f")) -> ("State with Arguments"=w419:string)  [unwired: 4 in]
                    n203 = local write "Status"("Finite Acquisition" ("Status")) -> ()
                    n204 = call <vilib>:"Add State(s) to Queue__jki_lib_state_machine.vi"("State(s) in Front (\"\")"="Lockin SMO: Set AO Zero Amplitude" ("f"), "State(s) in (\"\")"=w419, "State(s) at Back (\"\")"=w418) -> ("States Out"=w422:string)  [unwired: 12 in]
                    n205 = Bundle By Name(cluster=w430, "to"=100) -> (w429:T36)
                    n206 = call <vilib>:"Add State(s) to Queue__jki_lib_state_machine.vi"("State(s) in Front (\"\")"=w422, "State(s) at Back (\"\")"="Lockin SMO: Set AO" ("f")) -> ("States Out"=w420:string)  [unwired: 13 in]
                  }
                }
              }
              frame False {
                n207 = property on="Start" class="Bool (strict)"("Val(Sgnl)"=TRUE ("Value (Signaling)")) -> ()  [unwired: 2 in, 2 out]
              }
            }
            n208 = call <vilib>:"Add State(s) to Queue__jki_lib_state_machine.vi"("State(s) in Front (\"\")"=w397, "State(s) in (\"\")"=w405) -> ("States Out"=w404:string)  [unwired: 13 in]
          }
          event "Trigger": Value Change {
            w449 = T48 10178 items=["Finite Samples"=10178, "Continuous Samples"=10123] ("Sample Mode")
            # "Trigger Button Value Change (pressed) Event\nIf DAQ=idle:\n1. put into finite sample mode\n2. start (one) acquisition)\nIf DAQ=running:\n1. Stop current acquisition\n2. put into finite sample mode\n3. start (one) acquisition)"
            n209 = event-data() -> ()  [unwired: 1 in, 2 out]
            n210 = disable-structure shown="Disabled" {
              frame Disabled {
                n211 = local write "Trigger"(FALSE ("Trigger")) -> ()
              }
              frame Enabled {
              }
            }
            n212 = Unbundle By Name(w450) -> ("Lockin"=w437:refnum<class "Instrument.Lockin.lvclass">)
            n213 = Unbundle By Name(w437) -> ("DAQ state"=w438:T32)
            n214 = case shown="\"created\"" w438 {
              tunnel: ["" ("State with Arguments") w456] -> w441
              frame "idle", Default {
              }
              frame "created" {
                n215 = Format Into String(Set_State-enum."stop" ("State")) -> (resulting string=w459:string)  [unwired: 3 in, 1 out]
                n216 = call <vilib>:"Build State String with Arguments__JKI_lib_State_Machine.vi"("Arguments (\"\")"=w459, "State"="Lockin SMO: Set State" ("f")) -> ("State with Arguments"=w456:string)  [unwired: 4 in]
              }
            }
            n217 = local write "Pause"(TRUE ("Pause")) -> ()
            n218 = Format Into String(w449) -> (resulting string=w448:string)  [unwired: 3 in, 1 out]
            n219 = Format Into String(Set_State-enum."start" ("State")) -> (resulting string=w444:string)  [unwired: 3 in, 1 out]
            n220 = call <vilib>:"Build State String with Arguments__JKI_lib_State_Machine.vi"("Arguments (\"\")"=w448, "State"="Lockin SMO: Set Sampling" ("f")) -> ("State with Arguments"=w443:string)  [unwired: 4 in]
            n221 = call <vilib>:"Build State String with Arguments__JKI_lib_State_Machine.vi"("Arguments (\"\")"=w444, "State"="Lockin SMO: Set State" ("f")) -> ("State with Arguments"=w442:string)  [unwired: 4 in]
            n222 = call <vilib>:"Add State(s) to Queue__jki_lib_state_machine.vi"("State(s) in Front (\"\")"=w441, "State(s) in (\"\")"=w443, "State(s) at Back (\"\")"=w442) -> ("States Out"=w440:string)  [unwired: 12 in]
            n223 = call <vilib>:"Add State(s) to Queue__jki_lib_state_machine.vi"("State(s) in Front (\"\")"=w440, "State(s) in (\"\")"=w453) -> ("States Out"=w452:string)  [unwired: 13 in]
          }
          event "Reset": Value Change {
            # "RESET Button Value Change (pressed) Event\n1. Call 4461: SETUP State to calculate new Sampling\ninformation\n2. If sampling information changes, \"Sampling: value\nchange event will be triggered.\n3. Sampling: Value Change will call Stop, Set Sampling, Start"
            n224 = event-data() -> ()  [unwired: 1 in, 1 out]
            n225 = disable-structure shown="Disabled" {
              frame Disabled {
                n226 = Format Into String(Set_State-enum."reset" ("State")) -> (resulting string=w468:string)  [unwired: 3 in, 1 out]
                n227 = call <vilib>:"Build State String with Arguments__JKI_lib_State_Machine.vi"("Arguments (\"\")"=w468, "State"="Lockin SMO: Set State" ("f")) -> ()  [unwired: 4 in, 1 out]
              }
              frame Enabled {
              }
            }
            n228 = local write "Reset"(FALSE ("Reset")) -> ()
            n229 = call <vilib>:"Add State(s) to Queue__jki_lib_state_machine.vi"("State(s) in Front (\"\")"="Macro: Initialize UI\nMacro: Initialize DAQ SMO\n//UI: Update Plot Names >>Reset" ("State(s) in Front (\"\")"), "State(s) in (\"\")"=w465) -> ("States Out"=w464:string)  [unwired: 13 in]
          }
          event "Measure": Value Change {
            # "Measure Offset Button Value Change (pressed) Event\n1. send \"measure offset\" command to DAQ"
            n230 = event-data() -> ()  [unwired: 1 in, 1 out]
            n231 = local write "Measure"(FALSE ("Measure\nOffset")) -> ()
            n232 = call <vilib>:"Add State(s) to Queue__jki_lib_state_machine.vi"("State(s) in Front (\"\")"="Lockin SMO: Measure Offset" ("State(s) in Front (\"\")")) -> ("States Out"=w471:string)  [unwired: 14 in]
            n233 = call <vilib>:"Add State(s) to Queue__jki_lib_state_machine.vi"("State(s) in Front (\"\")"=w471, "State(s) in (\"\")"=w475) -> ("States Out"=w474:string)  [unwired: 13 in]
          }
          event "Reset Phase": Value Change {
            # "Measure Offset Button Value Change (pressed) Event\n1. send \"measure offset\" command to DAQ"
            n234 = event-data() -> ()  [unwired: 1 in, 1 out]
            n235 = local write "Reset Phase"(FALSE ("Measure\nOffset")) -> ()
            n236 = call <vilib>:"Add State(s) to Queue__jki_lib_state_machine.vi"("State(s) in Front (\"\")"="Lockin SMO: Reset Phase" ("State(s) in Front (\"\")")) -> ("States Out"=w478:string)  [unwired: 14 in]
            n237 = call <vilib>:"Add State(s) to Queue__jki_lib_state_machine.vi"("State(s) in Front (\"\")"=w478, "State(s) in (\"\")"=w482) -> ("States Out"=w481:string)  [unwired: 13 in]
          }
          event "Disable all AI Ref": Value Change {
            # "Measure Offset Button Value Change (pressed) Event\n1. send \"measure offset\" command to DAQ"
            n238 = event-data() -> ()  [unwired: 1 in, 1 out]
            n239 = local write "Disable all AI Ref"(FALSE ("Measure\nOffset")) -> ()
            n240 = call <vilib>:"Build State String with Arguments__JKI_lib_State_Machine.vi"("Arguments (\"\")"="Disable" ("Arguments (\"\")"), "State"="UI: Update AI Reference Channels" ("State(s) in Front (\"\")")) -> ("State with Arguments"=w486:string)  [unwired: 4 in]
            n241 = call <vilib>:"Add State(s) to Queue__jki_lib_state_machine.vi"("State(s) in Front (\"\")"=w486, "State(s) in (\"\")"=w490) -> ("States Out"=w489:string)  [unwired: 13 in]
          }
          event "Enable only AI Ref1": Value Change {
            # "Measure Offset Button Value Change (pressed) Event\n1. send \"measure offset\" command to DAQ"
            n242 = event-data() -> ()  [unwired: 1 in, 1 out]
            n243 = local write "Enable only AI Ref1"(FALSE ("Measure\nOffset")) -> ()
            n244 = call <vilib>:"Build State String with Arguments__JKI_lib_State_Machine.vi"("Arguments (\"\")"="All 1" ("Arguments (\"\")"), "State"="UI: Update AI Reference Channels" ("State(s) in Front (\"\")")) -> ("State with Arguments"=w494:string)  [unwired: 4 in]
            n245 = call <vilib>:"Add State(s) to Queue__jki_lib_state_machine.vi"("State(s) in Front (\"\")"=w494, "State(s) in (\"\")"=w498) -> ("States Out"=w497:string)  [unwired: 13 in]
          }
          event "auto DAQ": Value Change {
            # "Measure Offset Button Value Change (pressed) Event\n1. send \"measure offset\" command to DAQ"
            n246 = event-data() -> ()  [unwired: 1 in, 1 out]
            n247 = local write "auto DAQ"(FALSE ("Measure\nOffset")) -> ()
            n248 = call <vilib>:"Add State(s) to Queue__jki_lib_state_machine.vi"("State(s) in Front (\"\")"="Lockin SMO: Auto DAQ" ("State(s) in Front (\"\")")) -> ("States Out"=w501:string)  [unwired: 14 in]
            n249 = call <vilib>:"Add State(s) to Queue__jki_lib_state_machine.vi"("State(s) in Front (\"\")"=w501, "State(s) in (\"\")"=w505) -> ("States Out"=w504:string)  [unwired: 13 in]
          }
          event "Remove": Value Change {
            # "Zero Offset Button Value Change (pressed) Event\n1. send \"zero offset\" command to DAQ"
            n250 = event-data() -> ()  [unwired: 1 in, 1 out]
            n251 = local write "Remove"(FALSE ("Zero\nOffset")) -> ()
            n252 = call <vilib>:"Add State(s) to Queue__jki_lib_state_machine.vi"("State(s) in Front (\"\")"="Lockin SMO: Remove Offset" ("State(s) in Front (\"\")")) -> ("States Out"=w508:string)  [unwired: 14 in]
            n253 = call <vilib>:"Add State(s) to Queue__jki_lib_state_machine.vi"("State(s) in Front (\"\")"=w508, "State(s) in (\"\")"=w512) -> ("States Out"=w511:string)  [unwired: 13 in]
          }
          event "Close": Value Change {
            w513 = "Macro: Exit"
            # "Stop Button Value Change (pressed) Event\n(this executes Macro: Exit to terminate the VI)"
            n254 = event-data() -> ("OldVal"=w514:bool)  [unwired: 1 in]
            n255 = local write "Close"(w514) -> ()
            n256 = disable-structure shown="Disabled" {
              disable-tunnel: w513 -> [w519 _]
              frame Disabled {
                n257 = Two Button Dialog(message="Are you sure you want to exit?") -> (T button?=w521:bool)  [unwired: 2 in]
                n258 = Select(t=w519, s=w521, f="") -> ()  [unwired: 1 out]
              }
              frame Enabled {
              }
            }
            n259 = call <vilib>:"Add State(s) to Queue__jki_lib_state_machine.vi"("State(s) in Front (\"\")"=w513, "State(s) in (\"\")"=w518) -> ("States Out"=w517:string)  [unwired: 13 in]
          }
          event "Start Sweep": Value Change {
            # "New Start Button Value Change (pressed) Event"
            n260 = event-data() -> ()  [unwired: 1 in, 1 out]
            n261 = Unbundle By Name(w527) -> ("Lockin.DAQ"=w525:refnum<class "Instrument.DAQ.lvclass">)
            n262 = Bundle By Name(cluster=T24 {"Sweep Time (s)"=0.0, "Initial Wait (s)"=0.0, "Return to Start"=FALSE, "Channels"=[]} ("Configure Sweep"), "Channels"="Channels: Sweep", "Sweep Time (s)"="Sweep Time (s)", "Initial Wait (s)"="Initial Wait (s)", "Return to Start"="Return to Start?") -> (w534:T24)
            n263 = call "DAQ.setSweep.vi"("error in (no error)"=w536, "setSweep"=w534, "Instrument.DAQ"=w525) -> ("error out"=w523:errorcluster)  [unwired: 7 in, 1 out]
            n264 = Format Into String(Set_State-enum."start sweep" ("State")) -> (resulting string=w533:string)  [unwired: 3 in, 1 out]
            n265 = call <vilib>:"Build State String with Arguments__JKI_lib_State_Machine.vi"("Arguments (\"\")"=w533, "State"="Lockin SMO: Set State" ("f")) -> ("State with Arguments"=w530:string)  [unwired: 4 in]
            n266 = call <vilib>:"Add State(s) to Queue__jki_lib_state_machine.vi"("State(s) in Front (\"\")"=w530, "State(s) in (\"\")"=w538) -> ("States Out"=w537:string)  [unwired: 13 in]
          }
          event "Stop Sweep": Value Change {
            # "New Start Button Value Change (pressed) Event"
            n267 = event-data() -> ()  [unwired: 1 in, 6 out]
            n268 = local write "Stop Sweep"(FALSE ("Sweep Start")) -> ()
            n269 = Format Into String(Set_State-enum."stop sweep" ("State")) -> (resulting string=w542:string)  [unwired: 3 in, 1 out]
            n270 = call <vilib>:"Build State String with Arguments__JKI_lib_State_Machine.vi"("Arguments (\"\")"=w542, "State"="Lockin SMO: Set State" ("f")) -> ("State with Arguments"=w539:string)  [unwired: 4 in]
            n271 = call <vilib>:"Add State(s) to Queue__jki_lib_state_machine.vi"("State(s) in Front (\"\")"=w539, "State(s) in (\"\")"=w547) -> ("States Out"=w546:string)  [unwired: 13 in]
          }
          event "Load Configuration": Value Change {
            # "LOAD CONFIG Button Value Change (pressed) Event"
            n272 = event-data() -> ("NewVal"=w552:bool)  [unwired: 1 in, 1 out]
            n273 = local write "Load Configuration"(FALSE ("load config")) -> ()
            n274 = Select(t="" ("State(s) at Back (\"\")"), s=w552, f="") -> (s? t:f=w549:string)
            n275 = call <vilib>:"Add State(s) to Queue__jki_lib_state_machine.vi"("State(s) in Front (\"\")"=w549, "State(s) in (\"\")"=w556) -> ("States Out"=w555:string)  [unwired: 13 in]
          }
          event "Save Configuration": Value Change {
            # "save config Button Value Change (pressed) Event"
            n276 = event-data() -> ("NewVal"=w559:bool)  [unwired: 1 in]
            n277 = local write "Save Configuration"(FALSE ("save config")) -> ()
            n278 = Select(t="" ("State(s) at Back (\"\")"), s=w559, f="") -> (s? t:f=w560:string)
            n279 = call <vilib>:"Add State(s) to Queue__jki_lib_state_machine.vi"("State(s) in Front (\"\")"=w560, "State(s) in (\"\")"=w565) -> ("States Out"=w564:string)  [unwired: 13 in]
          }
          event "Help": Value Change {
            # "Help Button Value Change (pressed) Event\nIf Help = True: Send user to help webpage; Set Help=False\nIf Help=Fale, Do nothing"
            n280 = event-data() -> ("NewVal"=w566:bool)  [unwired: 1 in]
            n281 = case shown="False" w566 {
              tunnel: w568 -> [w572 w576]
              tunnel: [w572 w574] -> w567
              frame False {
              }
              frame True {
                n282 = local write "Help"(FALSE ("Help")) -> ()
                n283 = call-poly <vilib>:"Open URL in Default Browser.vi"("error in (no error)"=w576, "URL"="https://app.asana.com/0/205665857037275/list") -> ("error out"=w574:errorcluster)  [unwired: 4 in, 1 out]
              }
            }
            n284 = call <vilib>:"Add State(s) to Queue__jki_lib_state_machine.vi"("State(s) in (\"\")"=w571) -> ("States Out"=w570:string)  [unwired: 14 in]
          }
          event Panel Close? {
            w577 = "Macro: Exit"
            # "Discard the event because we'll close the front panel ourselves in Macro: Exit"
            # "Close Panel button (pressed) Event\n(this executes Macro: Exit to terminate the VI)"
            n285 = event-data() -> ()  [unwired: 1 in, 1 out]
            n286 = disable-structure shown="Disabled" {
              disable-tunnel: w577 -> [w583 _]
              frame Disabled {
                n287 = Two Button Dialog(message="Are you sure you want to exit?") -> (T button?=w585:bool)  [unwired: 2 in]
                n288 = Select(t=w583, s=w585, f="") -> ()  [unwired: 1 out]
              }
              frame Enabled {
              }
            }
            n289 = call <vilib>:"Add State(s) to Queue__jki_lib_state_machine.vi"("State(s) in Front (\"\")"=w577, "State(s) in (\"\")"=w578) -> ("States Out"=w582:string)  [unwired: 13 in]
            n290 = event-data("Discard?"=TRUE) -> ()  [unwired: 1 in, 1 out]
          }
        }
      }
      frame "---------- Core ----------" {
        # "Do not put any code in this frame.\n(it is a separator no-op)"
        n291 = call <vilib>:"Add State(s) to Queue__jki_lib_state_machine.vi"("State(s) in (\"\")"=w591) -> ("States Out"=w590:string)  [unwired: 14 in]
      }
      frame Default {
        w603 = 42 items=["No error", "Argument error", "Memory is full", "Out of zone", "End of file", "File already open", "Generic file I/O error", "File not found", "File permission error", "Disk is full", "Duplicate path", "Too many files open", "System feature not enabled", "Resource file not found", "Cannot add resource", "Resource not found", "Image not found", "Image memory error", "Pen does not exist", "Config type invalid", "Config token not found", "Config parse error", "Config memory error", "Bad external code format", "Bad external code offset", "External code not present", "Null window", "Destroy window error", "Null menu", "Print aborted", "Bad print record", "Print driver error", "Windows error during printing", "Memory error during printing", "Print dialog error", "Generic print error", "Invalid device refnum", "Device not found", "Device parameter error", "Device unit error", "Cannot open device", "Device call aborted", "Generic error", "Cancelled by user", "Object ID too low", "Object ID too high", "Object not in heap", "Unknown heap", "Unknown object (invalid DefProc)", "Unknown object (DefProc not in table)", "Message out of range", "Invalid (null) method", "Unknown message", "Manager call not supported", "Bad address", "Network operation in progress", "Network operation timed out", "Connection is busy", "Network attribute not supported", "Network error", "Address in use", "System out of memory", "Connection aborted", "Connection refused", "Not connected", "Already connected", "Connection closed", "Initialization error (interapplication manager)", "Bad occurrence", "Wait on unbound occurrence handler", "Occurrence queue overflow", "Datalog type conflict", "Unused", "Unrecognized type (interapplication manager)", "Memory corrupt", "Failed to make temporary DLL", "Old CIN version", "Drag socket not found", "Failed to load drop-object", "Failed to register OLE object", "Failed to release OLE object", "Format specifier type mismatch", "Unknown format specifier", "Too few format specifiers", "Too many format specifiers", "Scan failed", "Newer CIN version", "Error converting to variant", "Runtime menu error", "Password tampered", "Variant attribute not found", "Incompatible variant data type", "Event data is not available", "Event Store is not present", "Occurrence is not found", "Event Queue is not created", "Event info is not available", "Refnum passed is NULL", "Error retrieving Class GUID", "Error retrieving CoClass GUID", "Error retrieving TypeLib GUID.", "Bad built application magic bytes.", "Specific driver is different from the specific driver associated with the Logical Name.", "There is no session opened to the class driver.", "Max Error", "MAX - Error with config objects", "MAX - Error loading configuration", "MAX - Group not supported"]
        # "Current State"
        # "Do not delete, rename, or modify this frame.\n(this is used to capture unhandled states and typos)"
        # "Handle mistyped state name (developer tool)"
        n292 = Format Into String(format string="Software Exception: Unhandled State \"%s\"." ("message"), error in=w599, w594) -> (resulting string=w602:string, error out=w601:errorcluster)  [unwired: 1 in]
        n293 = call <vilib>:"Error Cluster From Error Code.vi"("show call chain? (False)"=TRUE, "error in (no error)"=w601, "error message (\"\")"=w602, "error code (0)"=w603) -> ("error out"=w600:errorcluster)  [unwired: 5 in]
        n294 = call <vilib>:"Add State(s) to Queue__jki_lib_state_machine.vi"("State(s) in (\"\")"=w598) -> ("States Out"=w597:string)  [unwired: 14 in]
      }
      frame "Initialize Core Data" {
        # "Do not delete, rename, or modify this frame.\n(this is used to determine panel behavior on exit)"
        # "originally closed?"
        # "exe?"
        # "If panel starts closed or is an EXE, then close it when we exit"
        n295 = property class="VI"() -> ("Front Panel.Open"=w612:bool)  [unwired: 2 in, 2 out]
        n296 = property class="App"() -> ("App.Kind"=w611:T27)  [unwired: 2 in, 2 out]
        n297 = control-ref of="Current VI Reference"() -> (w605:refnum<vi>)
        n298 = Not(x=w612) -> (.not. x?=w609:bool)
        n299 = Equal?(x=w611, y=T27."Run Time System" ("Application:Kind")) -> (x = y?=w608:bool)
        n300 = Or(x=w609, y=w608) -> (x .or. y?=w606:bool)
        n301 = Bundle By Name(cluster=w607, "Core.Current VI Reference"=w605, "Core.Close Panel on Exit?"=w606) -> (w614:T36)
        n302 = call <vilib>:"Add State(s) to Queue__jki_lib_state_machine.vi"("State(s) in (\"\")"=w616) -> ("States Out"=w615:string)  [unwired: 14 in]
      }
      frame "Error Handler" {
        # "Handle any errors here.\nYou can also output any states to clean-up after errors occur"
        # "Clear error"
        n303 = Unbundle By Name(w621) -> ("Lockin"=w620:refnum<class "Instrument.Lockin.lvclass">)
        n304 = call-dynamic "Handle Error.vi"("Stop on Unhandled Error (T)"=FALSE, "error in"=w618, "SMO"=w620) -> ("handling error"=w617:errorcluster)  [unwired: 6 in, 2 out]
        n305 = call-poly <userlib>:"Filter Error Codes__ogtk.vi"("Error In"=w617, "Error Codes to Filter"=i32[] [-200077, -200462, -200245, -200279]) -> ("Error Out"=w625:errorcluster)  [unwired: 7 in, 2 out]
        n306 = case shown="Error" w625 {
          selector: w625 -> [w630 w635]
          tunnel: ["" "Macro: Exit"] -> w627
          tunnel: [w630 w632] -> w623
          frame No Error {
          }
          frame Error {
            w633 = T49 1 items=["no dialog", "OK message", "continue or stop message", "OK message + warnings", "continue/stop + warnings"] ("type of dialog (OK msg:1)")
            # "Unhandled Error -- Display it"
            n307 = call <vilib>:"General Error Handler.vi"("type of dialog (OK msg:1)"=w633, "error in (no error)"=w635) -> ("error out"=w632:errorcluster)  [unwired: 9 in, 4 out]
          }
        }
        n308 = call <userlib>:"Clear All Errors__ogtk.vi"("Error In"=w623) -> ("Error Out"=w622:errorcluster)  [unwired: 3 in]
        n309 = call <vilib>:"Add State(s) to Queue__jki_lib_state_machine.vi"("State(s) in Front (\"\")"=w627, "State(s) in (\"\")"=w629) -> ("States Out"=w628:string)  [unwired: 13 in]
      }
      frame "Exit" {
        # "Do not put any code in this frame.\n(No errors that occur here will be handled.)"
        n310 = call <vilib>:"Add State(s) to Queue__jki_lib_state_machine.vi"("State(s) in (\"\")"=w641) -> ("States Out"=w640:string)  [unwired: 14 in]
      }
      frame "---------- Data ----------" {
        # "Do not put any code in this frame.\n(It is a separator no-op. You can make a copy of this frame to create a new Data frame)"
        n311 = call <vilib>:"Add State(s) to Queue__jki_lib_state_machine.vi"("State(s) in (\"\")"=w646) -> ("States Out"=w645:string)  [unwired: 14 in]
      }
      frame "Data: Initialize" {
        w648 = T34 {"Command"="", "Data"=variant, "ID"=""}  # Message
        w649 = refnum<class "Logger.Error.lvclass"> refnum  # Logger.Error
        w651 = refnum<class "Instrument.DAQ.lvclass"> refnum  # Lockin.DAQ
        w654 = T35 {"Sweep AO"=[], "Sweep AI"=[], "Sweep Results X"=[], "Sweep Results Y"=[]}  # SweepWaveforms
        w656 = T33 {"address"="", "Port"=0, "AllowedRemote"="", "Commands"=[], "timeout"=0}  # RemoteControl.Configure
        (unwired) T50 {"Time Stamp"=timestamp(0 s since 1904-01-01), "Results (Dictionary)"=[]}  # Results
        w657 = T34 {"Command"="", "Data"=variant, "ID"=""}  # HandledMessage
        w647 = refnum<class "Instrument.Lockin.lvclass"> refnum  # Lockin
        w650 = refnum<class "RemoteControl.lvclass"> refnum  # RemoteControl
        (unwired) waveform(dbl)[] []  # AI WFM
        w652 = 100  # to
        (unwired) waveform(dbl)[] []  # AO WFM
        (unwired) waveform(dbl)[] []  # REF WFM
        w659 = T51 {"Current VI Reference"=refnum, "Close Panel on Exit?"=FALSE}  # Core
        # "#todo\nPut all of this stuff on the class wire\nso I can use Handle Command.vi..."
        # "is sent to RC:process"
        # "comes from RC:process"
        # "do not delete - used by framework"
        # "Initialize the shift-register data, here.\n(data names are defined by what you wire into the bundle function)"
        n312 = call <vilib>:"Add State(s) to Queue__jki_lib_state_machine.vi"("State(s) in (\"\")"=w661) -> ("States Out"=w660:string)  [unwired: 14 in]
        n313 = Bundle("Core"=w659, "to"=w652, "Lockin"=w647, "RemoteControl"=w650, "Lockin.DAQ"=w651, "Logger.Error"=w649, "RemoteControl.Configure"=w656, "Message"=w648, "HandledMessage"=w657, "SweepWaveforms"=w654) -> (w655:T36)  [unwired: 1 in]
      }
      frame "Data: Adjust Channels" {
        # "#todo\nshould some of these methods be owned by Lockin.DAQ?"
        n314 = Unbundle By Name(w668) -> ("Lockin"=w669:refnum<class "Instrument.Lockin.lvclass">)
        n315 = call "Initialize REF Channels.vi"("error in (no error)"=w670, "Instrument.Lockin"=w669) -> ("error out"=w671:errorcluster, "Instrument.Lockin out"=w672:refnum<class "Instrument.Lockin.lvclass">)  [unwired: 7 in, 1 out]
        n316 = call "Initialize AO Channels.vi"("error in (no error)"=w671, "Instrument.Lockin"=w672) -> ("error out"=w676:errorcluster, "Instrument.Lockin out"=w678:refnum<class "Instrument.Lockin.lvclass">)  [unwired: 7 in, 1 out]
        n317 = call "Limit AO Amplitude.vi"("error in (no error)"=w676, "Limit Amplitudes"="Limit Amplitudes", "AO Amp Limit"="AO Amp Limit", "Instrument.Lockin in"=w678) -> ("error out"=w675:errorcluster, "Instrument.Lockin out"=w677:refnum<class "Instrument.Lockin.lvclass">)  [unwired: 6 in]
        n318 = call "Set all f same.vi"("error in (no error)"=w675, "Link Frequencies"="Link Frequencies", "AO f"="AO freq link", "Instrument.Lockin"=w677) -> ("error out"=w663:errorcluster, "Instrument.Lockin out"=w673:refnum<class "Instrument.Lockin.lvclass">)  [unwired: 6 in]
        n319 = Unbundle By Name(w673) -> ("AO"=w662:T52, "REF"=w679:T38)
        n320 = Bundle By Name(cluster=w668, "Lockin"=w673) -> (w667:T36)
        n321 = local write "REF Channels"(w679) -> ()
        n322 = local write "AO Channels"(w662) -> ()
        n323 = call <vilib>:"Add State(s) to Queue__jki_lib_state_machine.vi"("State(s) in (\"\")"=w682) -> ("States Out"=w681:string)  [unwired: 14 in]
      }
      frame "Data: Cleanup" {
        # "Cleanup any data and references, here.\n(this is called automatically, by the Macro: Exit)"
        n324 = Unbundle By Name(w684) -> ("Core.Current VI Reference"=w686:refnum<vi>)
        n325 = Close Reference(reference=w686, error in (no error)=w685) -> (error out=w683:errorcluster)
        n326 = call <vilib>:"Add State(s) to Queue__jki_lib_state_machine.vi"("State(s) in (\"\")"=w689) -> ("States Out"=w688:string)  [unwired: 14 in]
      }
      frame "---------- Events ----------" {
        # "Template Separator\n(You can make a copy of, or modify, this frame)"
        n327 = call <vilib>:"Add State(s) to Queue__jki_lib_state_machine.vi"("State(s) in (\"\")"=w694) -> ("States Out"=w693:string)  [unwired: 14 in]
      }
      frame "Events: Register" {
        w703 = T54 {"Error"=refnum, "State"=refnum, "Reserve State"=refnum}  # LockinDAQ SMO Public Events
        w712 = T54 {"Error"=refnum, "State"=refnum, "Reserve State"=refnum}  # RC SMO Public Events
        n328 = Unbundle By Name(w716) -> ("RemoteControl"=w708:refnum<class "RemoteControl.lvclass">, "Lockin.DAQ"=w695:refnum<class "Instrument.DAQ.lvclass">)
        n329 = call <vilib>:"GetPublicEvents.vi"("SMO"=w708) -> ("error out"=w707:errorcluster, "Public Events"=w711:T54, "SMO out"=w705:refnum<class "RemoteControl.lvclass">)  [unwired: 8 in]
        n330 = Variant To Data(error in=w707, type=w712, Variant=w711) -> (data=w710:T54, error out=w706:errorcluster)
        n331 = call <vilib>:"GetPublicEvents.vi"("SMO"=w695) -> ("error out"=w700:errorcluster, "Public Events"=w702:T54, "SMO out"=w698:refnum<class "Instrument.DAQ.lvclass">)  [unwired: 8 in]
        n332 = call <userlib>:"RemoteControl.GetPublicEvents.vi"("RemoteControl"=w705) -> ("error out"=w704:errorcluster, "RC Public Events"=w715:T55)  [unwired: 8 in, 1 out]
        n333 = Variant To Data(error in=w700, type=w703, Variant=w702) -> (data=w701:T54, error out=w699:errorcluster)
        n334 = call "DAQ.GetPublicEvents.vi"("Instrument.DAQ"=w698) -> ("error out"=w713:errorcluster, "DAQ Public Events"=w709:T56)  [unwired: 8 in, 1 out]
        n335 = register-events(w710, w715, w701, w709) -> (reference out=w717:refnum<event-registration>, error out=w714:errorcluster)  [unwired: 2 in]
        n336 = Merge Errors(w714, w713, w704, w699, w706, w696) -> (w697:errorcluster)
        n337 = call <vilib>:"Add State(s) to Queue__jki_lib_state_machine.vi"("State(s) in (\"\")"=w719) -> ("States Out"=w718:string)  [unwired: 14 in]
      }
      frame "Events: Unregister" {
        n338 = Unregister For Events(event registration refnum=w721, error in=w720) -> (error out=w722:errorcluster)
        n339 = call <vilib>:"Clear Errors.vi"("error in (no error)"=w722) -> ()  [unwired: 5 in, 2 out]
        n340 = call <vilib>:"Add State(s) to Queue__jki_lib_state_machine.vi"("State(s) in (\"\")"=w725) -> ("States Out"=w724:string)  [unwired: 14 in]
      }
      frame "---------- UI ----------" {
        # "Do not put any code in this frame.\n(It is a separator no-op. You can make a copy of this frame to create a new UI frame)"
        n341 = call <vilib>:"Add State(s) to Queue__jki_lib_state_machine.vi"("State(s) in (\"\")"=w730) -> ("States Out"=w729:string)  [unwired: 14 in]
      }
      frame "UI: Initialize" {
        w731 = waveform(dbl)[][] [] ("History Data")
        # "#done"
        # "Initialize the User Interface, here.\n(this is called automatically, by the Macro: Init)"
        n342 = call <userlib>:"MGI Get Executable Version.vi"() -> ("Version"=w736:string)  [unwired: 7 in]
        n343 = Empty String/Path?(string/path=w736) -> (empty?=w737:bool)
        n344 = invoke on="Start" class="Bool (strict)" method="Reinit To Default"() -> ()  [unwired: 3 in, 3 out]
        n345 = invoke on="Start Sweep" class="Bool (strict)" method="Reinit To Default"() -> ()  [unwired: 3 in, 3 out]
        n346 = Select(t=w733, s=w737, f=w736) -> (s? t:f=w735:string)
        n347 = Format Into String(format string="v%s", w735) -> (resulting string=→"Version":string)  [unwired: 2 in, 1 out]
        n348 = invoke on="Reset" class="Bool (strict)" method="Reinit To Default"() -> ()  [unwired: 3 in, 3 out]
        n349 = invoke on="Close" class="Bool (strict)" method="Reinit To Default"() -> ()  [unwired: 3 in, 3 out]
        n350 = property on="Lockin 1" class="WFChart (strict)"("History Data"=w731) -> ()  [unwired: 2 in, 2 out]
        n351 = local write "Tab Control 2"(T20."AO/AI Display" ("Tab Control 2")) -> ()
        n352 = local write "Tab Control 4"(T28."AO/REF Setup" ("Tab Control 4")) -> ()
        n353 = property on="Lockin 2" class="WFChart (strict)"("History Data"=w731) -> ()  [unwired: 2 in, 2 out]
        n354 = local write "Status"("Starting" ("Status")) -> ()
        n355 = invoke on="Trigger" class="Bool (strict)" method="Reinit To Default"() -> ()  [unwired: 3 in, 3 out]
        n356 = invoke on="Help" class="Bool (strict)" method="Reinit To Default"() -> ()  [unwired: 3 in, 3 out]
        n357 = call <userlib>:"Fit VI window to Largest Dec__ogtk.vi"("error in (no error)"=w740) -> ("error out"=w742:errorcluster)  [unwired: 5 in, 1 out]
        n358 = call <vilib>:"Add State(s) to Queue__jki_lib_state_machine.vi"("State(s) in (\"\")"=w746) -> ("States Out"=w745:string)  [unwired: 14 in]
      }
      frame "UI: Initialize REF Ch" {
        # "#done"
        n359 = Unbundle By Name(w753) -> ("Lockin"=w752:refnum<class "Instrument.Lockin.lvclass">)
        n360 = call "Initialize REF Channels.vi"("error in (no error)"=w750, "Instrument.Lockin"=w752) -> ("error out"=w748:errorcluster, "REF Channels out"=w749:T38, "Instrument.Lockin out"=w751:refnum<class "Instrument.Lockin.lvclass">)  [unwired: 7 in]
        n361 = property on="REF Channels" class="Arr (strict)"(error in=w748, "Val(Sgnl)"=w749) -> (error out=w747:errorcluster)  [unwired: 1 in, 1 out]
        n362 = Bundle By Name(cluster=w753, "Lockin"=w751) -> (w754:T36)
        n363 = call <vilib>:"Add State(s) to Queue__jki_lib_state_machine.vi"("State(s) in (\"\")"=w757) -> ("States Out"=w756:string)  [unwired: 14 in]
      }
      frame "UI: Initialize AO Ch" {
        # "#done"
        n364 = Unbundle By Name(w764) -> ("Lockin"=w763:refnum<class "Instrument.Lockin.lvclass">)
        n365 = call "Initialize AO Channels.vi"("error in (no error)"=w761, "Instrument.Lockin"=w763) -> ("error out"=w760:errorcluster, "Channels: AO"=w759:T52, "Instrument.Lockin out"=w762:refnum<class "Instrument.Lockin.lvclass">)  [unwired: 7 in]
        n366 = property on="AO Channels" class="Arr (strict)"(error in=w760, "Val(Sgnl)"=w759) -> (error out=w758:errorcluster)  [unwired: 1 in, 1 out]
        n367 = Bundle By Name(cluster=w764, "Lockin"=w762) -> (w765:T36)
        n368 = call <vilib>:"Add State(s) to Queue__jki_lib_state_machine.vi"("State(s) in (\"\")"=w768) -> ("States Out"=w767:string)  [unwired: 14 in]
      }
      frame "UI: Update AI Ch" {
        # "Add or remove AI channels"
        n369 = Unbundle By Name(w775) -> ("Lockin"=w773:refnum<class "Instrument.Lockin.lvclass">)
        n370 = call "Initialize AI Channels.vi"("error in (no error)"=w772, "Instrument.Lockin"=w773) -> ("error out"=w771:errorcluster, "Configuration.Channels.AI"=w774:T57, "Instrument.Lockin out"=w769:refnum<class "Instrument.Lockin.lvclass">)  [unwired: 7 in]
        n371 = property on="AI Channels" class="Arr (strict)"(error in=w771, "Val(Sgnl)"=w774) -> (error out=w770:errorcluster)  [unwired: 1 in, 1 out]
        n372 = Bundle By Name(cluster=w775, "Lockin"=w769) -> (w776:T36)
        n373 = call <vilib>:"Add State(s) to Queue__jki_lib_state_machine.vi"("State(s) in (\"\")"=w779) -> ("States Out"=w778:string)  [unwired: 14 in]
      }
      frame "UI: Update AI Reference Channels" {
        # "Add or remove AI channels"
        n374 = Unbundle By Name(w788) -> ("Lockin"=w785:refnum<class "Instrument.Lockin.lvclass">)
        n375 = case shown="\"All 1\"" w780 {
          tunnel: [u16[] [1] ("References") u16[] [0] ("References")] -> w781
          frame "All 1" {
          }
          frame "Disable", Default {
          }
        }
        n376 = Unbundle By Name(w785) -> ("AI"=w786:T57)
        n377 = for {
          tunnel: w786 -> [w797] mode=indexing
          tunnel: [w796] -> w784 mode=indexing
          tunnel: w781 -> [w795]
          n378 = Bundle By Name(cluster=w797, "References"=w795) -> (w796:T58)
        }
        n379 = Bundle By Name(cluster=w785, "AI"=w784) -> (w783:refnum<class "Instrument.Lockin.lvclass">)
        n380 = property on="AI Channels" class="Arr (strict)"(error in=w782, "Val(Sgnl)"=w784) -> (error out=w787:errorcluster)  [unwired: 1 in, 1 out]
        n381 = Bundle By Name(cluster=w788, "Lockin"=w783) -> (w789:T36)
        n382 = call <vilib>:"Add State(s) to Queue__jki_lib_state_machine.vi"("State(s) in (\"\")"=w792) -> ("States Out"=w791:string)  [unwired: 14 in]
      }
      frame "UI: Initialize Gains" {
        n383 = Unbundle By Name(w808) -> ("Lockin"=w807:refnum<class "Instrument.Lockin.lvclass">)
        n384 = call "Initialize Input Gain.vi"("error in (no error)"=w806, "Instrument.Lockin"=w807) -> ("error out"=w804:errorcluster, "Input Gain"=w802:cluster{string, "Gain":dbl}[], "Instrument.Lockin out"=w805:refnum<class "Instrument.Lockin.lvclass">)  [unwired: 7 in]
        n385 = property on="Input Gain" class="Arr (strict)"(error in=w804, "Val(Sgnl)"=w802) -> (error out=w803:errorcluster)  [unwired: 1 in, 1 out]
        n386 = call "Initialize Ouput Gain.vi"("error in (no error)"=w803, "Instrument.Lockin"=w805) -> ("error out"=w799:errorcluster, "Ouput Gain"=w801:cluster{string, "Gain":dbl}[], "Instrument.Lockin out"=w800:refnum<class "Instrument.Lockin.lvclass">)  [unwired: 7 in]
        n387 = property on="Output Gain" class="Arr (strict)"(error in=w799, "Val(Sgnl)"=w801) -> (error out=w798:errorcluster)  [unwired: 1 in, 1 out]
        n388 = Bundle By Name(cluster=w808, "Lockin"=w800) -> (w809:T36)
        n389 = call <vilib>:"Add State(s) to Queue__jki_lib_state_machine.vi"("State(s) in (\"\")"=w812) -> ("States Out"=w811:string)  [unwired: 14 in]
      }
      frame "UI: Update Rings" {
        # "update Sweep Channel ring"
        n390 = Unbundle By Name(w826) -> ("Lockin"=w825:refnum<class "Instrument.Lockin.lvclass">)
        n391 = disable-structure shown="Disabled" {
          frame Disabled {
            n392 = call "Get AI REF (f) StringsAndValues.vi"() -> ("error out"=w833:errorcluster, "AI REF (f) StringsAndValues"=w832:cluster{string, i32}[], "Instrument.Lockin out"=w831:refnum<class "Instrument.Lockin.lvclass">)  [unwired: 9 in]
            n393 = property on="Channel" class="Ring (strict)"(error in=w833, "StringsAndValues[]"=w832) -> ()  [unwired: 1 in, 2 out]
          }
          frame Enabled {
          }
        }
        n394 = call "Get AO StringsAndValues.vi"("error in (no error)"=w824, "Instrument.Lockin in"=w825) -> ("error out"=w822:errorcluster, "AO Strings and Values"=w823:cluster{string, i32}[], "Instrument.Lockin out"=w820:refnum<class "Instrument.Lockin.lvclass">)  [unwired: 7 in]
        n395 = property on="Channel" class="Ring (strict)"(error in=w822, "StringsAndValues[]"=w823) -> (error out=w819:errorcluster)  [unwired: 1 in, 1 out]
        n396 = call "Get REF StringsAndValues.vi"("error in (no error)"=w819, "Instrument.Lockin in"=w820) -> ("error out"=w821:errorcluster, "REF Strings and Values"=w818:cluster{string, i32}[], "Instrument.Lockin out"=w817:refnum<class "Instrument.Lockin.lvclass">)  [unwired: 7 in]
        n397 = property on="Reference" class="Ring (strict)"(error in=w821, "StringsAndValues[]"=w818) -> (error out=w815:errorcluster)  [unwired: 1 in, 1 out]
        n398 = call "Remote Unused References.vi"("error in (no error)"=w815, "Instrument.Lockin in"=w817) -> ("error out"=w814:errorcluster, "Array"=w813:T58[], "Instrument.Lockin out"=w816:refnum<class "Instrument.Lockin.lvclass">)  [unwired: 7 in]
        n399 = Bundle By Name(cluster=w826, "Lockin"=w816) -> (w827:T36)
        n400 = local write "AI Channels"(w813) -> ()
        n401 = call <vilib>:"Add State(s) to Queue__jki_lib_state_machine.vi"("State(s) in (\"\")"=w830) -> ("States Out"=w829:string)  [unwired: 14 in]
      }
      frame "UI: Update Plot Names" {
        n402 = Unbundle By Name(w837) -> ("Lockin"=w842:refnum<class "Instrument.Lockin.lvclass">)
        n403 = call "Get AO StringsAndValues.vi"("error in (no error)"=w834, "Instrument.Lockin in"=w842) -> ("error out"=w844:errorcluster, "AO Strings and Values"=w839:cluster{string, i32}[])  [unwired: 7 in, 1 out]
        n404 = call "Get AI StringsAndValues.vi"("error in (no error)"=w834, "Instrument.Lockin in"=w842) -> ("error out"=w845:errorcluster, "AI StringsAndValues"=w846:cluster{string, i32}[])  [unwired: 7 in, 1 out]
        n405 = call "Get AI REF StringsAndValues.vi"("error in (no error)"=w834, "Instrument.Lockin in"=w842) -> ("error out"=w835:errorcluster, "REF StringsAndValues"=w836:cluster{string, i32}[])  [unwired: 7 in, 1 out]
        n406 = for {
          tunnel: w839 -> [w863] mode=indexing
          tunnel: w844 -> [w864]
          tunnel: [w861] -> w843
          i -> [w865]
          n407 = control-ref of="Sweep Results AO"() -> (w862:refnum<vi>)
          n408 = Unbundle(w863) -> (w866:string)  [unwired: 1 out]
          n409 = call-poly "Set Legend.vi"("error in (no error)"=w864, "Plot.Plot Name"=w866, "Active Plot"=w865, "WFGraph in"=w862) -> ("error out"=w861:errorcluster)  [unwired: 4 in, 3 out]
        }
        n410 = for {
          tunnel: w846 -> [w876] mode=indexing
          tunnel: w845 -> [w877]
          tunnel: [w871] -> w848
          i -> [w878]
          n411 = control-ref of="AI Graph"() -> (w879:refnum<vi>)
          n412 = Unbundle(w876) -> (w880:string)  [unwired: 1 out]
          n413 = control-ref of="Sweep Results AI"() -> (w867:refnum<vi>)
          n414 = call-poly "Set Legend.vi"("error in (no error)"=w877, "Plot.Plot Name"=w880, "Active Plot"=w878, "WFGraph in"=w879) -> ("error out"=w875:errorcluster, "Plot.Plot Name"=w874:string, "Active Plot"=w873:i32)  [unwired: 4 in, 1 out]
          n415 = call-poly "Set Legend.vi"("error in (no error)"=w875, "Plot.Plot Name"=w874, "Active Plot"=w873, "WFGraph in"=w867) -> ("error out"=w872:errorcluster, "Plot.Plot Name"=w870:string, "Active Plot"=w869:i32)  [unwired: 4 in, 1 out]
          n416 = control-ref of="PS WFGraph"() -> (w868:refnum<vi>)
          n417 = call-poly "Set Legend.vi"("error in (no error)"=w872, "Plot.Plot Name"=w870, "Active Plot"=w869, "WFGraph (WDT) in"=w868) -> ("error out"=w871:errorcluster)  [unwired: 4 in, 3 out]
          n418 = call-poly "Set Legend.vi"("WFGraph (WDT) in"=w868) -> ()  [unwired: 7 in, 4 out]
          n419 = call-poly "Set Legend.vi"("WFGraph in"=w867) -> ()  [unwired: 7 in, 4 out]
        }
        n420 = local read "Y Axis (Output)"() -> (w838:enum16{"Analog Output", "Reference"})
        n421 = case shown="\"Analog Output\", Default" w838 {
          tunnel: [w852 w854] -> w841
          tunnel: w836 -> [_ w853]
          tunnel: w839 -> [w852 _]
          frame "Analog Output", Default {
          }
          frame "Reference" {
            n422 = Interleave 1D Arrays(w853, w853) -> (w854:cluster{string, i32}[])
          }
        }
        n423 = for {
          tunnel: w841 -> [w859] mode=indexing
          tunnel: w835 -> [w857]
          tunnel: [w856] -> w840
          i -> [w858]
          n424 = Unbundle(w859) -> (w855:string)  [unwired: 1 out]
          n425 = control-ref of="AO Graph"() -> (w860:refnum<vi>)
          n426 = call-poly "Set Legend.vi"("error in (no error)"=w857, "Plot.Plot Name"=w855, "Active Plot"=w858, "WFGraph in"=w860) -> ("error out"=w856:errorcluster)  [unwired: 4 in, 3 out]
        }
        n427 = call <vilib>:"Add State(s) to Queue__jki_lib_state_machine.vi"("State(s) in (\"\")"=w851) -> ("States Out"=w850:string)  [unwired: 14 in]
        n428 = Merge Errors(w843, w848, w840, w834) -> (w847:errorcluster)
      }
      frame "UI: Sync Lockin Plot Visibility" {
        # "#todo"
        # "#done"
        # "number of results"
        # "Do not put any code in this frame.\n(It is a separator no-op. You can make a copy of this frame to create a new UI frame)"
        n429 = local read "Results Plot Names"() -> (w883:string[])
        n430 = Array Size(array=w883) -> (size(s)=w884:i32)
        n431 = feedback #1() -> (w886:string[])  [unwired: 1 in]
        n432 = feedback-in #1(w883) -> ()
        n433 = Not Equal?(x=w886, y=w883) -> (x != y?=w888:bool)
        n434 = First Call?() -> (First Call?: T/F=w889:bool)
        n435 = Or(x=w889, y=w888) -> (x .or. y?=w887:bool)
        n436 = case shown="True" w887 {
          tunnel: w882 -> [w911 w915]
          tunnel: w883 -> [_ w916]
          tunnel: [w911 w912] -> w885
          frame False {
          }
          frame True {
            n437 = for {
              tunnel: w915 -> [w937]
              tunnel: [w922] -> w913
              tunnel: w916 -> [w917] mode=indexing
              i -> [w932]
              n438 = control-ref of="XY Graph"() -> (w927:refnum<vi>)
              n439 = control-ref of="Lockin 2"() -> (w928:refnum<vi>)
              n440 = control-ref of="Lockin 1"() -> (w929:refnum<vi>)
              n441 = call-poly "Set Legend.vi"("error in (no error)"=w937, "Plot.Plot Name"=w917, "Active Plot"=w932, "WaveformChart in"=w929) -> ("error out"=w933:errorcluster, "Plot.Plot Name"=w931:string, "Active Plot"=w936:i32)  [unwired: 4 in, 1 out]
              n442 = control-ref of="Sweep Results Y"() -> (w925:refnum<vi>)
              n443 = control-ref of="Sweep Results X"() -> (w926:refnum<vi>)
              n444 = call-poly "Set Legend.vi"("error in (no error)"=w933, "Plot.Plot Name"=w931, "Active Plot"=w936, "WaveformChart in"=w928) -> ("error out"=w934:errorcluster, "Plot.Plot Name"=w930:string, "Active Plot"=w935:i32)  [unwired: 4 in, 1 out]
              n445 = call "Set Legend (XYGraph).vi"("error in (no error)"=w934, "Plot.Plot Name"=w930, "Active Plot"=w935, "XYGraph in"=w927) -> ("error out"=w924:errorcluster, "Plot.Plot Name"=w918:string, "Active Plot"=w921:i32)  [unwired: 4 in, 1 out]
              n446 = call-poly "Set Legend.vi"("error in (no error)"=w924, "Plot.Plot Name"=w918, "Active Plot"=w921, "WFGraph in"=w926) -> ("error out"=w923:errorcluster, "Plot.Plot Name"=w919:string, "Active Plot"=w920:i32)  [unwired: 4 in, 1 out]
              n447 = call-poly "Set Legend.vi"("error in (no error)"=w923, "Plot.Plot Name"=w919, "Active Plot"=w920, "WFGraph in"=w925) -> ("error out"=w922:errorcluster)  [unwired: 4 in, 3 out]
            }
            n448 = property on="Channel" class="Ring (strict)"(error in=w915, "Strings []"=w916) -> (error out=w914:errorcluster)  [unwired: 1 in, 1 out]
            n449 = Merge Errors(w914, w913) -> (w912:errorcluster)
          }
        }
        n450 = for {
          N: w884 -> [_]
          tunnel: w885 -> [w900]
          tunnel: [w895] -> w881
          i -> [w909]
          n451 = control-ref of="Lockin 1"() -> (w910:refnum<vi>)
          n452 = call "Get Plot Visibility (WFChart).vi"("error in (no error)"=w900, "ActPlot"=w909, "WaveformChart in"=w910) -> ("error out"=w899:errorcluster, "Plot.Visible?"=w894:bool, "Active Plot"=w904:i32)  [unwired: 6 in]
          n453 = control-ref of="Lockin 2"() -> (w908:refnum<vi>)
          n454 = call-poly "Set Plot Visibility.vi"("error in (no error)"=w899, "Plot.Visible?"=w894, "ActPlot"=w904, "WaveformChart in"=w908) -> ("error out"=w898:errorcluster, "Active Plot"=w903:i32)  [unwired: 6 in]
          n455 = control-ref of="XY Graph"() -> (w907:refnum<vi>)
          n456 = call-poly "Set Plot Visibility.vi"("error in (no error)"=w898, "Plot.Visible?"=w894, "ActPlot"=w903, "XYGraph in"=w907) -> ("error out"=w897:errorcluster, "Active Plot"=w902:i32)  [unwired: 6 in]
          n457 = control-ref of="Sweep Results Y"() -> (w906:refnum<vi>)
          n458 = control-ref of="Sweep Results X"() -> (w905:refnum<vi>)
          n459 = call-poly "Set Plot Visibility.vi"("error in (no error)"=w897, "Plot.Visible?"=w894, "ActPlot"=w902, "WFGraph in"=w906) -> ("error out"=w896:errorcluster, "Active Plot"=w901:i32)  [unwired: 6 in]
          n460 = call-poly "Set Plot Visibility.vi"("error in (no error)"=w896, "Plot.Visible?"=w894, "ActPlot"=w901, "WFGraph in"=w905) -> ("error out"=w895:errorcluster)  [unwired: 6 in, 1 out]
        }
        n461 = call <vilib>:"Add State(s) to Queue__jki_lib_state_machine.vi"("State(s) in (\"\")"=w893) -> ("States Out"=w892:string)  [unwired: 14 in]
      }
      frame "UI: Sync AO AI Plot Visibility" {
        # "#done"
        # "Do not put any code in this frame.\n(It is a separator no-op. You can make a copy of this frame to create a new UI frame)"
        n462 = Unbundle By Name(w944) -> ("Lockin"=w942:refnum<class "Instrument.Lockin.lvclass">)
        n463 = call "Get AO StringsAndValues.vi"("error in (no error)"=w940, "Instrument.Lockin in"=w942) -> ("error out"=w938:errorcluster, "AO Strings and Values"=w941:cluster{string, i32}[])  [unwired: 7 in, 1 out]
        n464 = call "Get AI StringsAndValues.vi"("error in (no error)"=w940, "Instrument.Lockin in"=w942) -> ("error out"=w939:errorcluster, "AI StringsAndValues"=w943:cluster{string, i32}[])  [unwired: 7 in, 1 out]
        n465 = for {
          tunnel: w939 -> [w964]
          tunnel: [w960] -> w946
          tunnel: w943 -> [_] mode=indexing
          i -> [w967]
          n466 = control-ref of="AI Graph"() -> (w963:refnum<vi>)
          n467 = property on="Property Node" class="WFGraph (strict)"(reference=w963, error in=w964, "Active Plot"=w967) -> (error out=w968:errorcluster, "Plot.Visible?"=w966:bool)  [unwired: 1 out]
          n468 = control-ref of="Sweep Results AI"() -> (w965:refnum<vi>)
          n469 = property on="Property Node" class="WFGraph (strict)"(reference=w965, error in=w968, "Active Plot"=w967, "Plot.Visible?"=w966) -> (error out=w961:errorcluster)  [unwired: 1 out]
          n470 = call <vilib>:"Clear Errors.vi"("error in (no error)"=w961, "specific error code to clear (0: all)"=1077) -> ("error out"=w960:errorcluster)  [unwired: 4 in, 1 out]
        }
        n471 = for {
          tunnel: w938 -> [w954]
          tunnel: [w951] -> w947
          tunnel: w941 -> [_] mode=indexing
          i -> [w958]
          n472 = control-ref of="AO Graph"() -> (w955:refnum<vi>)
          n473 = property on="Property Node" class="WFGraph (strict)"(reference=w955, error in=w954, "Active Plot"=w958) -> (error out=w959:errorcluster, "Plot.Visible?"=w957:bool)  [unwired: 1 out]
          n474 = control-ref of="Sweep Results AO"() -> (w956:refnum<vi>)
          n475 = property on="Property Node" class="WFGraph (strict)"(reference=w956, error in=w959, "Active Plot"=w958, "Plot.Visible?"=w957) -> (error out=w952:errorcluster)  [unwired: 1 out]
          n476 = call <vilib>:"Clear Errors.vi"("error in (no error)"=w952, "specific error code to clear (0: all)"=1077) -> ("error out"=w951:errorcluster)  [unwired: 4 in, 1 out]
        }
        n477 = Merge Errors(w946, w947) -> (w945:errorcluster)
        n478 = call <vilib>:"Add State(s) to Queue__jki_lib_state_machine.vi"("State(s) in (\"\")"=w950) -> ("States Out"=w949:string)  [unwired: 14 in]
      }
      frame "UI: Disable Buttons" {
        # "#done"
        n479 = control-ref of="Start"() -> (w974:refnum<vi>)
        n480 = control-ref of="Pause"() -> (w973:refnum<vi>)
        n481 = control-ref of="Trigger"() -> (w972:refnum<vi>)
        n482 = control-ref of="Reset"() -> (w971:refnum<vi>)
        n483 = control-ref of="Help"() -> (w970:refnum<vi>)
        n484 = Build Array(w974, w973, w972, w971, w970) -> (w969:refnum<vi>[])
        n485 = for {
          tunnel: w969 -> [w981] mode=indexing
          n486 = property class="Bool (strict)"(reference=w981, "DisabledEnum"=T29."Disabled and Grayed Out" ("Disabled")) -> ()  [unwired: 1 in, 2 out]
        }
        n487 = call <vilib>:"Add State(s) to Queue__jki_lib_state_machine.vi"("State(s) in (\"\")"=w979) -> ("States Out"=w978:string)  [unwired: 14 in]
      }
      frame "UI: Enable Buttons" {
        # "#done"
        n488 = control-ref of="Start"() -> (w987:refnum<vi>)
        n489 = control-ref of="Pause"() -> (w986:refnum<vi>)
        n490 = control-ref of="Trigger"() -> (w985:refnum<vi>)
        n491 = control-ref of="Reset"() -> (w984:refnum<vi>)
        n492 = control-ref of="Help"() -> (w983:refnum<vi>)
        n493 = Build Array(w987, w986, w985, w984, w983) -> (w982:refnum<vi>[])
        n494 = for {
          tunnel: w982 -> [w994] mode=indexing
          n495 = property class="Bool (strict)"(reference=w994, "DisabledEnum"=T29."Enabled" ("Disabled")) -> ()  [unwired: 1 in, 2 out]
        }
        n496 = call <vilib>:"Add State(s) to Queue__jki_lib_state_machine.vi"("State(s) in (\"\")"=w992) -> ("States Out"=w991:string)  [unwired: 14 in]
      }
      frame "UI: AI Graph Plot Visible" {
        # "#done"
        # "Do not put any code in this frame.\n(It is a separator no-op. You can make a copy of this frame to create a new UI frame)"
        n497 = case shown="\"None\", Default" w1000 {
          tunnel: [FALSE TRUE] -> w997
          frame "None", Default {
          }
          frame "ALL" {
          }
        }
        n498 = control-ref of="AI Graph"() -> (w1001:refnum<vi>)
        n499 = control-ref of="Sweep Results AI"() -> (w998:refnum<vi>)
        n500 = call-poly "Set All Plot Visibility.vi"("error in (no error)"=w999, "All Visible?"=w997, "WFGraph in"=w1001) -> ("error out"=w996:errorcluster)  [unwired: 7 in, 1 out]
        n501 = call-poly "Set All Plot Visibility.vi"("error in (no error)"=w996, "All Visible?"=w997, "WFGraph in"=w998) -> ("error out"=w995:errorcluster)  [unwired: 7 in, 1 out]
        n502 = call <vilib>:"Add State(s) to Queue__jki_lib_state_machine.vi"("State(s) in (\"\")"=w1005) -> ("States Out"=w1004:string)  [unwired: 14 in]
      }
      frame "UI: AO Graph Plot Visible" {
        # "#done"
        # "Do not put any code in this frame.\n(It is a separator no-op. You can make a copy of this frame to create a new UI frame)"
        n503 = case shown="\"ALL\"" w1014 {
          tunnel: [FALSE TRUE] -> w1010
          frame "None", Default {
          }
          frame "ALL" {
          }
        }
        n504 = control-ref of="AO Graph"() -> (w1012:refnum<vi>)
        n505 = call-poly "Set All Plot Visibility.vi"("error in (no error)"=w1013, "All Visible?"=w1010, "WFGraph in"=w1012) -> ("error out"=w1009:errorcluster)  [unwired: 7 in, 1 out]
        n506 = control-ref of="Sweep Results AO"() -> (w1011:refnum<vi>)
        n507 = call-poly "Set All Plot Visibility.vi"("error in (no error)"=w1009, "All Visible?"=w1010, "WFGraph in"=w1011) -> ("error out"=w1008:errorcluster)  [unwired: 7 in, 1 out]
        n508 = call <vilib>:"Add State(s) to Queue__jki_lib_state_machine.vi"("State(s) in (\"\")"=w1018) -> ("States Out"=w1017:string)  [unwired: 14 in]
      }
      frame "UI: Lockin 1 Plot Visible" {
        # "#done"
        # "Do not put any code in this frame.\n(It is a separator no-op. You can make a copy of this frame to create a new UI frame)"
        n509 = case shown="\"ALL\"" w1033 {
          tunnel: [FALSE TRUE] -> w1029
          frame "None", Default {
          }
          frame "ALL" {
          }
        }
        n510 = control-ref of="Lockin 1"() -> (w1032:refnum<vi>)
        n511 = control-ref of="Lockin 2"() -> (w1030:refnum<vi>)
        n512 = control-ref of="Sweep Results X"() -> (w1028:refnum<vi>)
        n513 = control-ref of="Sweep Results Y"() -> (w1027:refnum<vi>)
        n514 = call-poly "Set All Plot Visibility.vi"("error in (no error)"=w1031, "All Visible?"=w1029, "WaveformChart in"=w1032) -> ("error out"=w1025:errorcluster)  [unwired: 7 in, 1 out]
        n515 = call-poly "Set All Plot Visibility.vi"("error in (no error)"=w1025, "All Visible?"=w1029, "WaveformChart in"=w1030) -> ("error out"=w1024:errorcluster)  [unwired: 7 in, 1 out]
        n516 = call-poly "Set All Plot Visibility.vi"("error in (no error)"=w1024, "All Visible?"=w1029, "WFGraph in"=w1028) -> ("error out"=w1023:errorcluster)  [unwired: 7 in, 1 out]
        n517 = control-ref of="XY Graph"() -> (w1026:refnum<vi>)
        n518 = call-poly "Set All Plot Visibility.vi"("error in (no error)"=w1023, "All Visible?"=w1029, "WFGraph in"=w1027) -> ("error out"=w1022:errorcluster)  [unwired: 7 in, 1 out]
        n519 = call-poly "Set All Plot Visibility.vi"("error in (no error)"=w1022, "All Visible?"=w1029, "XYGraph in"=w1026) -> ("error out"=w1021:errorcluster)  [unwired: 7 in, 1 out]
        n520 = call <vilib>:"Add State(s) to Queue__jki_lib_state_machine.vi"("State(s) in (\"\")"=w1037) -> ("States Out"=w1036:string)  [unwired: 14 in]
      }
      frame "UI: Update Waveform Graphs" {
        # "#todo\nshould be owned by Lockin UI"
        # "private"
        # "private"
        n521 = Unbundle By Name(w1058) -> ("Lockin"=w1051:refnum<class "Instrument.Lockin.lvclass">)
        n522 = Unbundle By Name(w1051) -> ("Input Gain"=w1047:dbl[], "AI"=w1061:waveform(dbl)[], "AO"=w1041:waveform(dbl)[], "RefX"=w1043:waveform(dbl)[], "RefY"=w1042:waveform(dbl)[])
        n523 = local read "Y Axis (Output)"() -> (w1044:enum16{"Analog Output", "Reference"})
        n524 = Interleave 1D Arrays(w1043, w1042) -> (w1040:waveform(dbl)[])
        n525 = case shown="\"Analog Output\", Default" w1044 {
          tunnel: w1041 -> [w1069 _]
          tunnel: w1040 -> [_ w1070]
          tunnel: [w1069 w1070] -> w1052
          frame "Analog Output", Default {
          }
          frame "Reference" {
          }
        }
        n526 = local read "X Axis"() -> (w1049:enum16{"Time", "Samples"})
        n527 = Power Of 10(x="Decimate") -> (10^x=w1053:dbl)
        n528 = call "Display n or dt.vi"("error in (no error)"=w1050, "X Axis"=w1049, "Input Waveforms"=w1061) -> ("error out"=w1060:errorcluster, "Output Waveforms"=w1048:waveform(dbl)[])  [unwired: 7 in]
        n529 = call "Display n or dt.vi"("error in (no error)"=w1050, "X Axis"=w1049, "Input Waveforms"=w1052) -> ("error out"=w1059:errorcluster, "Output Waveforms"=w1064:waveform(dbl)[])  [unwired: 7 in]
        n530 = call "decimate_waveforms.vi"("WFM"=w1064, "averaging"=FALSE, "decimating factor"=w1053, "error in (no error)"=w1059) -> ("WFM out"=→"AO Graph":waveform(dbl)[])  [unwired: 5 in, 1 out]
        n531 = call "decimate_waveforms.vi"("WFM"=w1048, "averaging"=FALSE, "decimating factor"=w1053, "error in (no error)"=w1060) -> ("WFM out"=w1057:waveform(dbl)[], "error out"=w1055:errorcluster)  [unwired: 5 in]
        n532 = case shown="\"ADC\"" "Y Axis (Input)" {
          tunnel: w1057 -> [w1072 w1077]
          tunnel: w1047 -> [_ w1075]
          tunnel: [w1072 w1076] -> w1056
          tunnel: w1055 -> [w1071 w1074]
          tunnel: [w1071 w1073] -> w1046
          frame "Device", Default {
          }
          frame "ADC" {
            n533 = call "Multiply by Gain.vi"("error in (no error)"=w1074, "Gain"=w1075, "WFM in"=w1077) -> ("error out"=w1073:errorcluster, "WFM out"=w1076:waveform(dbl)[])  [unwired: 7 in]
          }
        }
        "AI Graph" <- w1056
        n534 = call <vilib>:"Add State(s) to Queue__jki_lib_state_machine.vi"("State(s) in (\"\")"=w1068) -> ("States Out"=w1067:string)  [unwired: 14 in]
      }
      frame "UI: Update Lockin Graphs" {
        # "#todo\nshould be owned by Lockin UI"
        # "#todo\nshould be owned by Lockin UI"
        # "#todo\nshould be owned by Lockin UI"
        n535 = Unbundle By Name(w1095) -> ("Lockin"=w1085:refnum<class "Instrument.Lockin.lvclass">)
        n536 = call "Parse Results (table).vi"("error in (no error)"=w1090, "Instrument.Lockin"=w1085) -> ("error out"=w1089:errorcluster, "Table"=→"Results":string[][], "Results (Dictionary)"=w1084:cluster{"key":string, "value":dbl}[])  [unwired: 6 in, 1 out]
        n537 = call "Dictionary to Chart.vi"("error in (no error)"=w1089, "Display"="Display", "Results.Results (Dictionary)"=w1084) -> ("error out"=w1091:errorcluster, "XY Graph"=→"XY Graph":cluster{dbl[], dbl[]}[], "Y/Theta Array"=→"Lockin 2":waveform(dbl)[], "X/R Array"=→"Lockin 1":waveform(dbl)[], "Plot Names"=→"Results Plot Names":string[])  [unwired: 4 in]
        n538 = call "Dictionary to Indicator.vi"("Results.Results (Dictionary)"=w1084, "AI Channel"="Channel", "error in (no error)"=w1091) -> ("X"=→"X":dbl, "Y"=→"Y":dbl, "R"=→"R":dbl, "Theta"=→"Theta":dbl, "error out"=w1083:errorcluster)  [unwired: 8 in]
        n539 = call <vilib>:"Add State(s) to Queue__jki_lib_state_machine.vi"("State(s) in (\"\")"=w1098) -> ("States Out"=w1097:string)  [unwired: 14 in]
      }
      frame "UI: Update Waveform Graph Labels" {
        n540 = control-ref of="AI Graph"() -> (w1103:refnum<vi>)
        n541 = control-ref of="AO Graph"() -> (w1100:refnum<vi>)
        n542 = call "Set AO AI Graph X Axis (WFGraph).vi"("error in (no error)"=w1105, "X Axis"="X Axis", "WaveformGraph in"=w1103) -> ("error out"=w1107:errorcluster)  [unwired: 8 in]
        n543 = call "Set AO AI Graph X Axis (WFGraph).vi"("error in (no error)"=w1107, "X Axis"="X Axis", "WaveformGraph in"=w1100) -> ("error out"=w1106:errorcluster)  [unwired: 8 in]
        n544 = control-ref of="AO Graph"() -> (w1101:refnum<vi>)
        n545 = call "Set AO Graph Y Axis (WFGraph).vi"("error in (no error)"=w1106, "Y Axis (Output)"="Y Axis (Output)", "WaveformGraph in"=w1101) -> ("error out"=w1104:errorcluster)  [unwired: 8 in]
        n546 = call <vilib>:"Add State(s) to Queue__jki_lib_state_machine.vi"("State(s) in (\"\")"=w1111) -> ("States Out"=w1110:string)  [unwired: 14 in]
      }
      frame "UI: Update Lockin Graph Range" {
        n547 = Negate(x="Numeric") -> (-x=w1114:dbl)
        n548 = Negate(x="X/R Range") -> (-x=w1116:dbl)
        n549 = Negate(x="Y/Theta Range") -> (-x=w1117:dbl)
        n550 = property on="Lockin 1" class="WFChart (strict)"("YScale.Maximum"="X/R Range", "YScale.Minimum"=w1116) -> ()  [unwired: 2 in, 2 out]
        n551 = property on="Lockin 2" class="WFChart (strict)"("YScale.Maximum"="Y/Theta Range", "YScale.Minimum"=w1117) -> ()  [unwired: 2 in, 2 out]
        n552 = property on="XY Graph" class="XYGraph (strict)"("XScale.Maximum"="Numeric", "XScale.Minimum"=w1114, "YScale.Maximum"="Numeric", "YScale.Minimum"=w1114) -> ()  [unwired: 2 in, 2 out]
        n553 = call <vilib>:"Add State(s) to Queue__jki_lib_state_machine.vi"("State(s) in (\"\")"=w1122) -> ("States Out"=w1121:string)  [unwired: 14 in]
      }
      frame "UI: Update Displays" {
        n554 = local read "Display"() -> (w1125:T19)
        n555 = case shown="\"R and Theta\"" w1125 {
          tunnel: ["X (V)" "R (V)"] -> _
          tunnel: ["Y (V)" "Theta (°)"] -> _
          tunnel: ["Lockin X (V)" "R (V)"] -> w1124
          tunnel: ["Lockin Y (V)" "Theta (°)"] -> w1123
          frame "X and Y", Default {
          }
          frame "R and Theta" {
          }
        }
        n556 = property on="Lockin 1" class="WFChart (strict)"("YScale.NameLbl.Text"=w1124) -> ()  [unwired: 2 in, 2 out]
        n557 = property on="Lockin 2" class="WFChart (strict)"("YScale.NameLbl.Text"=w1123) -> ()  [unwired: 2 in, 2 out]
        n558 = call <vilib>:"Add State(s) to Queue__jki_lib_state_machine.vi"("State(s) in (\"\")"=w1130) -> ("States Out"=w1129:string)  [unwired: 14 in]
      }
      frame "UI: Update Sweep Results Graphs" {
        n559 = Unbundle By Name(w1142) -> ("Lockin"=w1141:refnum<class "Instrument.Lockin.lvclass">)
        n560 = Unbundle By Name(w1141) -> ("Sweep Results X"=→"Sweep Results X":waveform(dbl)[], "Sweep Results Y"=→"Sweep Results Y":waveform(dbl)[])
        n561 = call <vilib>:"Add State(s) to Queue__jki_lib_state_machine.vi"("State(s) in (\"\")"=w1146) -> ("States Out"=w1145:string)  [unwired: 14 in]
      }
      frame "UI: Update Sweep WFMs Graphs" {
        n562 = Unbundle By Name(w1149) -> ("SweepWaveforms.Sweep AO"=→"Sweep Results AO":waveform(dbl)[], "SweepWaveforms.Sweep AI"=→"Sweep Results AI":waveform(dbl)[])
        n563 = call <vilib>:"Add State(s) to Queue__jki_lib_state_machine.vi"("State(s) in (\"\")"=w1153) -> ("States Out"=w1152:string)  [unwired: 14 in]
      }
      frame "UI: Update Status" {
        n564 = Unbundle By Name(w1156) -> ("Lockin"=w1155:refnum<class "Instrument.Lockin.lvclass">)
        n565 = Unbundle By Name(w1155) -> ("DAQ state"=w1154:T32)
        n566 = case shown="\"idle\", Default" w1154 {
          tunnel: ["Idle" ("Status") "Started" ("Status") "Stopped" ("Status") "Running" ("Status") "Sweeping" ("Status")] -> w1157
          frame "idle", Default {
            w1163 = FALSE ("Trigger")
            n567 = local write "Reset"(w1163) -> ()
            n568 = local write "Trigger"(w1163) -> ()
            n569 = local write "Start"(w1163) -> ()
          }
          frame "started" {
            w1164 = FALSE ("Trigger")
            n570 = local write "Start Sweep"(w1164) -> ()
            n571 = local write "Reset"(w1164) -> ()
            n572 = local write "Stop Sweep"(w1164) -> ()
            n573 = disable-structure shown="Disabled" {
              frame Disabled {
                n574 = local read "Trigger"() -> ()  [unwired: 1 in]
              }
              frame Enabled {
              }
            }
            n575 = local write "Start"(TRUE ("Trigger")) -> ()
          }
          frame "stopped" {
            w1169 = FALSE ("Trigger")
            n576 = local write "Reset"(w1169) -> ()
            n577 = local write "Trigger"(w1169) -> ()
            n578 = local write "Start"(FALSE ("Trigger")) -> ()
          }
          frame "created" {
            n579 = local write "Start"(TRUE ("Start")) -> ()
            n580 = local write "Reset"(FALSE ("Reset")) -> ()
          }
          frame "sweeping" {
            n581 = call <userlib>:"MGI Milliseconds Since Last Reset.vi"("Reset (F)"=TRUE) -> ()  [unwired: 5 in, 2 out]
          }
        }
        n582 = local write "Status"(w1157) -> ()
        n583 = call <vilib>:"Add State(s) to Queue__jki_lib_state_machine.vi"("State(s) in (\"\")"=w1161) -> ("States Out"=w1160:string)  [unwired: 14 in]
      }
      frame "UI: Update Sweep Timer" {
        n584 = local read "Status"() -> (w1176:string)
        n585 = case shown="Default" w1176 {
          tunnel: [0.0 w1184] -> w1175
          frame Default {
          }
          frame "Sweeping" {
            # "some overhead"
            n586 = call <userlib>:"MGI Milliseconds Since Last Reset.vi"() -> ("ms"=w1190:u32)  [unwired: 6 in, 1 out]
            n587 = local read "Sweep Time (s)"() -> (w1186:dbl)
            n588 = local read "Initial Wait (s)"() -> (w1187:dbl)
            n589 = Divide(x=w1190, y=u32 1000) -> (x/y=w1188:dbl)
            n590 = Negate(x=w1188) -> (-x=w1185:dbl)
            n591 = Compound Arithmetic op=ADD(2.0 ("value"), w1187, w1186, w1185) -> (w1184:dbl)
          }
        }
        "Sweep Timer (s)" <- w1175
        n592 = call <vilib>:"Add State(s) to Queue__jki_lib_state_machine.vi"("State(s) in (\"\")"=w1181) -> ("States Out"=w1180:string)  [unwired: 14 in]
      }
      frame "UI: Cursor Set" {
        # "Argument"
        # "Set and Unset Cursor Busy.\n(Usage: \"UI: Cursor Set >> Busy|Idle\")"
        n593 = case shown="\"Busy\"" w1195 {
          tunnel: w1192 -> [w1199 w1201]
          tunnel: [w1198 w1200] -> w1191
          frame "Idle", Default {
            n594 = call <vilib>:"Unset Busy.vi"("error in (no error)"=w1199) -> ("error out"=w1198:errorcluster)  [unwired: 10 in]
          }
          frame "Busy" {
            n595 = call <vilib>:"Set Busy.vi"("error in (no error)"=w1201) -> ("error out"=w1200:errorcluster)  [unwired: 9 in, 1 out]
          }
        }
        n596 = call <vilib>:"Add State(s) to Queue__jki_lib_state_machine.vi"("State(s) in (\"\")"=w1197) -> ("States Out"=w1196:string)  [unwired: 14 in]
      }
      frame "UI: Front Panel State" {
        # "Argument"
        n597 = Unbundle By Name(w1204) -> ("Core.Current VI Reference"=w1206:refnum<vi>)
        n598 = case shown="\"Open\", Default" w1205 {
          tunnel: w1207 -> [w1213 w1226]
          tunnel: [w1215 w1227] -> w1203
          tunnel: w1206 -> [w1214 w1224]
          frame "Open", Default {
            n599 = property class="VI"(reference=w1214, error in=w1213) -> (reference out=w1211:refnum<vi>, error out=w1212:errorcluster, "Front Panel.Open"=w1210:bool)
            n600 = case shown="True" w1210 {
              tunnel: [w1218 w1221] -> w1215
              tunnel: w1212 -> [w1217 w1221]
              tunnel: w1211 -> [w1216 _]
              frame False {
                n601 = invoke class="VI" method="FP.Open"(reference=w1216, error in=w1217, "Activate"=TRUE, "State"=T30."Standard") -> (error out=w1218:errorcluster)  [unwired: 1 in, 4 out]
              }
              frame True {
              }
            }
          }
          frame "Close" {
            n602 = property class="VI"(reference=w1224, error in=w1226) -> (reference out=w1223:refnum<vi>, error out=w1225:errorcluster, "Front Panel.Open"=w1222:bool)
            n603 = case shown="True" w1222 {
              tunnel: [w1228 w1231] -> w1227
              tunnel: w1225 -> [w1228 w1230]
              tunnel: w1223 -> [_ w1229]
              frame False {
              }
              frame True {
                n604 = invoke class="VI" method="FP.Close"(reference=w1229, error in=w1230) -> (error out=w1231:errorcluster)  [unwired: 1 in, 2 out]
              }
            }
          }
        }
        n605 = call <vilib>:"Add State(s) to Queue__jki_lib_state_machine.vi"("State(s) in (\"\")"=w1209) -> ("States Out"=w1208:string)  [unwired: 14 in]
      }
      frame "UI: Cleanup" {
        w1233 = FALSE ("Close")
        w1232 = waveform(dbl)[] [] ("Signals Graph")
        w1235 = waveform(dbl)[][] [] ("History Data")
        # "Initialize the User Interface, here.\n(this is called automatically, by the Macro: Exit)"
        n606 = property on="Lockin 1" class="WFChart (strict)"("History Data"=w1235) -> ()  [unwired: 2 in, 2 out]
        n607 = local write "Sweep Results X"(w1232) -> ()
        n608 = local write "Sweep Results Y"(w1232) -> ()
        n609 = property on="AI Graph" class="WFGraph (strict)"("Value"=w1232) -> (error out=w1234:errorcluster)  [unwired: 2 in, 1 out]
        n610 = property on="Lockin 2" class="WFChart (strict)"("History Data"=w1235) -> ()  [unwired: 2 in, 2 out]
        n611 = property on="AO Graph" class="WFGraph (strict)"(error in=w1234, "Value"=w1232) -> ()  [unwired: 1 in, 2 out]
        n612 = local write "Self Calibrate"(w1233) -> ()
        n613 = local write "Trigger"(w1233) -> ()
        n614 = local write "Close"(w1233) -> ()
        n615 = local write "Pause"(w1233) -> ()
        n616 = local write "Reset"(w1233) -> ()
        n617 = local write "Start"(w1233) -> ()
        n618 = local write "Status"("Shutdown" ("Status")) -> ()
        n619 = call <vilib>:"Add State(s) to Queue__jki_lib_state_machine.vi"("State(s) in (\"\")"=w1241) -> ("States Out"=w1240:string)  [unwired: 14 in]
      }
      frame "---------- Macro ----------" {
        # "Do not put any code in this frame.\n(It is a separator no-op. You can make a copy of this frame to create a new Macro frame)"
        n620 = call <vilib>:"Add State(s) to Queue__jki_lib_state_machine.vi"("State(s) in (\"\")"=w1246) -> ("States Out"=w1245:string)  [unwired: 14 in]
      }
      frame "Macro: Initialize" {
        n621 = call <vilib>:"Add State(s) to Queue__jki_lib_state_machine.vi"("State(s) in Front (\"\")"="Data: Initialize\nInitialize Core Data\n\nUI: Initialize\n\nEvents: Register\n\n\nUI: Front Panel State >> Open\n\n\nMacro: Initialize UI\nUI: Update Sweep WFMs Graphs\nUI: Disable Buttons\n\n\nMacro: Initialize DAQ SMO", "State(s) in (\"\")"=w1247) -> ("States Out"=w1252:string)  [unwired: 13 in]
      }
      frame "Macro: Initialize UI" {
        n622 = call <vilib>:"Add State(s) to Queue__jki_lib_state_machine.vi"("State(s) in Front (\"\")"="UI: Initialize REF Ch\nUI: Initialize AO Ch\nUI: Initialize Gains\nUI: Update AI Ch\nUI: Update Plot Names\nUI: Update Waveform Graph Labels\nUI: Update Displays" ("State(s) in Front (\"\")"), "State(s) in (\"\")"=w1258) -> ("States Out"=w1257:string)  [unwired: 13 in]
      }
      frame "Macro: Initialize DAQ SMO" {
        n623 = Unbundle By Name(w1260) -> ("Lockin.DAQ"=w1263:refnum<class "Instrument.DAQ.lvclass">)
        n624 = while {
          tunnel: [w1278] -> w1261
          tunnel: w1263 -> [w1277]
          tunnel: w1262 -> [w1276]
          tunnel: [w1274] -> w1259
          i -> [w1271]
          stop <- w1268 stop-if-true
          n625 = call <vilib>:"GetState.vi"("error in (no error)"=w1276, "SMO"=w1277) -> ("error out"=w1275:errorcluster, "SMO State"=w1273:T16)  [unwired: 7 in, 1 out]
          n626 = case shown="Default" w1273 {
            tunnel: ["" "Lockin SMO: Set AI Config\nLockin SMO: Set AO Config\nLockin SMO: Set AI\nLockin SMO: Set AO\nLockin SMO: Set REF\nLockin SMO: Set Input Gain\nLockin SMO: Set Output Gain\nMacro: Update Sampling\n//Lockin SMO: Set Sampling"] -> w1278
            tunnel: w1275 -> [w1280 w1283]
            tunnel: [w1279 w1283] -> w1274
            frame Default {
              n627 = call <userlib>:"Wait (ms)__ogtk.vi"("error in (no error)"=w1280, "milliseconds to wait"=u32 100) -> ("error out"=w1279:errorcluster)  [unwired: 8 in, 1 out]
            }
            frame "Started" {
              # "send all stuff to the Lockin.DAQ"
            }
          }
          n628 = Equal?(x=w1273, y=SMOState_--Enum."Started") -> (x = y?=w1269:bool)
          n629 = Greater?(x=w1271, y=10) -> (0:w1267:bool)
          n630 = Or(x=w1269, y=w1267) -> (x .or. y?=w1268:bool)
        }
        n631 = call <vilib>:"Add State(s) to Queue__jki_lib_state_machine.vi"("State(s) in Front (\"\")"=w1261, "State(s) in (\"\")"=w1266) -> ("States Out"=w1265:string)  [unwired: 13 in]
      }
      frame "Macro: Update Sampling" {
        w1299 = T48 10123 items=["Finite Samples"=10178, "Continuous Samples"=10123] ("Sample Mode")
        w1298 = T48 10178 items=["Finite Samples"=10178, "Continuous Samples"=10123] ("Sample Mode")
        # "#todo\nthis \"macro\" needs to\nbe handled by Lockin.DAQ\nor Handle Command"
        n632 = Unbundle By Name(w1289) -> ("Lockin"=w1286:refnum<class "Instrument.Lockin.lvclass">)
        n633 = Unbundle By Name(w1286) -> ("DAQ state"=w1285:T32)
        n634 = local read "Start"() -> (w1287:bool)
        n635 = case shown="\"created\", Default" w1285 {
          tunnel: ["" ("State with Arguments") w1311] -> w1293
          frame "idle" {
          }
          frame "created", Default {
            n636 = Format Into String(Set_State-enum."start" ("State")) -> (resulting string=w1312:string)  [unwired: 3 in, 1 out]
            n637 = call <vilib>:"Build State String with Arguments__JKI_lib_State_Machine.vi"("Arguments (\"\")"=w1312, "State"="Lockin SMO: Set State" ("f")) -> ("State with Arguments"=w1311:string)  [unwired: 4 in]
          }
        }
        n638 = case shown="\"created\", Default" w1285 {
          tunnel: ["" ("State with Arguments") w1306] -> w1295
          frame "idle" {
          }
          frame "created", Default {
            n639 = Format Into String(Set_State-enum."stop" ("State")) -> (resulting string=w1309:string)  [unwired: 3 in, 1 out]
            n640 = call <vilib>:"Build State String with Arguments__JKI_lib_State_Machine.vi"("Arguments (\"\")"=w1309, "State"="Lockin SMO: Set State" ("f")) -> ("State with Arguments"=w1306:string)  [unwired: 4 in]
          }
        }
        n641 = Select(t=w1299, s=w1287, f=w1298) -> (s? t:f=w1297:T48)
        n642 = Format Into String(w1297) -> (resulting string=w1296:string)  [unwired: 3 in, 1 out]
        n643 = call <vilib>:"Build State String with Arguments__JKI_lib_State_Machine.vi"("Arguments (\"\")"=w1296, "State"="Lockin SMO: Set Sampling") -> ("State with Arguments"=w1294:string)  [unwired: 4 in]
        n644 = call <vilib>:"Add State(s) to Queue__jki_lib_state_machine.vi"("State(s) in Front (\"\")"=w1295, "State(s) in (\"\")"=w1294, "State(s) at Back (\"\")"=w1293) -> ("States Out"=w1288:string)  [unwired: 12 in]
        n645 = call <vilib>:"Add State(s) to Queue__jki_lib_state_machine.vi"("State(s) in Front (\"\")"="4461: SAMPLING SETUP" ("State(s) in Front (\"\")"), "State(s) in (\"\")"="" ("State(s) in Front (\"\")"), "State(s) at Back (\"\")"=w1288) -> ("States Out"=w1290:string)  [unwired: 12 in]
        n646 = call <vilib>:"Add State(s) to Queue__jki_lib_state_machine.vi"("State(s) in Front (\"\")"=w1290, "State(s) in (\"\")"=w1304) -> ("States Out"=w1303:string)  [unwired: 13 in]
      }
      frame "Macro: Exit" {
        # "Exit Macro\n(This is called once, when the VI exits)"
        n647 = Unbundle By Name(w1319) -> ("Core.Close Panel on Exit?"=w1323:bool)
        n648 = Select(t="UI: Front Panel State >> Close", s=w1323, f="") -> (s? t:f=w1322:string)
        n649 = call <vilib>:"Add State(s) to Queue__jki_lib_state_machine.vi"("State(s) in Front (\"\")"="Lockin SMO: Set AO Zero Amplitude\nUI: Disable Buttons\nUI: Cleanup", "State(s) in (\"\")"=w1322, "State(s) at Back (\"\")"="Events: Unregister\nData: Cleanup\nExit") -> ("States Out"=w1320:string)  [unwired: 12 in]
        n650 = call <vilib>:"Add State(s) to Queue__jki_lib_state_machine.vi"("State(s) in Front (\"\")"=w1320, "State(s) in (\"\")"=w1326) -> ("States Out"=w1325:string)  [unwired: 13 in]
      }
      frame "---------- Lockin SMO ----------" {
        n651 = call <vilib>:"Add State(s) to Queue__jki_lib_state_machine.vi"("State(s) in (\"\")"=w1331) -> ("States Out"=w1330:string)  [unwired: 14 in]
      }
      frame "Lockin SMO: Set State" {
        # "#lockin:process"
        n652 = Unbundle By Name(w1332) -> ("Lockin.DAQ"=w1338:refnum<class "Instrument.DAQ.lvclass">)
        n653 = case shown="\"start\"" w1334 {
          tunnel: [Set_State-enum."stop" ("State") Set_State-enum."start" ("State") Set_State-enum."reset" ("State") Set_State-enum."start sweep" ("State") Set_State-enum."stop sweep" ("State")] -> w1333
          tunnel: [FALSE ("Trigger") TRUE ("Trigger") w1346 TRUE ("Trigger") TRUE ("Trigger")] -> w1335
          frame "stop", Default {
          }
          frame "start" {
          }
          frame "reset" {
            n654 = local read "Start"() -> (w1346:bool)
          }
          frame "start sweep" {
          }
          frame "stop sweep" {
          }
        }
        n655 = local write "Start"(w1335) -> ()
        n656 = call "DAQ.setstate.vi"("error in (no error)"=w1337, "setState"=w1333, "Instrument.DAQ"=w1338) -> ("error out"=w1336:errorcluster)  [unwired: 7 in, 1 out]
        n657 = call <vilib>:"Add State(s) to Queue__jki_lib_state_machine.vi"("State(s) in (\"\")"=w1341) -> ("States Out"=w1340:string)  [unwired: 14 in]
      }
      frame "Lockin SMO: Set AI Config" {
        # "#lockin:process"
        n658 = Unbundle By Name(w1353) -> ("Lockin.DAQ"=w1358:refnum<class "Instrument.DAQ.lvclass">, "Lockin"=w1354:refnum<class "Instrument.Lockin.lvclass">)
        n659 = Unbundle By Name(w1354) -> ("AI"=w1355:T46)
        n660 = call "DAQ.setAIconfig.vi"("error in (no error)"=w1357, "Simulation mode"="AI Simulation mode", "AI Configuration"=w1355, "Instrument.DAQ"=w1358) -> ("error out"=w1356:errorcluster)  [unwired: 6 in, 1 out]
        n661 = call <vilib>:"Add State(s) to Queue__jki_lib_state_machine.vi"("State(s) in (\"\")"=w1361) -> ("States Out"=w1360:string)  [unwired: 14 in]
      }
      frame "Lockin SMO: Set AO Config" {
        # "#lockin:process"
        n662 = Unbundle By Name(w1363) -> ("Lockin.DAQ"=w1367:refnum<class "Instrument.DAQ.lvclass">, "Lockin"=w1364:refnum<class "Instrument.Lockin.lvclass">)
        n663 = Unbundle By Name(w1364) -> ("AO"=w1362:T44)
        n664 = call "DAQ.setAOconfig.vi"("error in (no error)"=w1366, "AO Configuration"=w1362, "Instrument.DAQ"=w1367) -> ("error out"=w1365:errorcluster)  [unwired: 7 in, 1 out]
        n665 = call <vilib>:"Add State(s) to Queue__jki_lib_state_machine.vi"("State(s) in (\"\")"=w1370) -> ("States Out"=w1369:string)  [unwired: 14 in]
      }
      frame "Lockin SMO: Set Sampling" {
        # "#lockin:process"
        # "Is there a more elegant way to do this?"
        n666 = Unbundle By Name(w1372) -> ("Lockin.DAQ"=w1379:refnum<class "Instrument.DAQ.lvclass">, "Lockin"=w1375:refnum<class "Instrument.Lockin.lvclass">)
        n667 = Unbundle By Name(w1375) -> ("Sampling"=w1373:T11)
        n668 = case shown="\"10178\", Default" w1374 {
          tunnel: [w1383 w1384] -> w1376
          frame "10178", Default {
            w1383 = T48 10178 items=["Finite Samples"=10178, "Continuous Samples"=10123] ("Sample Mode")
          }
          frame "10123" {
            w1384 = T48 10123 items=["Finite Samples"=10178, "Continuous Samples"=10123] ("Sample Mode")
          }
        }
        n669 = call "DAQ.setSampling.vi"("Decimation"="decimating factor", "error in (no error)"=w1378, "Sample Mode"=w1376, "Sampling"=w1373, "Instrument.DAQ"=w1379) -> ("error out"=w1377:errorcluster)  [unwired: 5 in, 1 out]
        n670 = call <vilib>:"Add State(s) to Queue__jki_lib_state_machine.vi"("State(s) in (\"\")"=w1382) -> ("States Out"=w1381:string)  [unwired: 14 in]
      }
      frame "Lockin SMO: Set AO" {
        # "#lockin:process"
        n671 = Unbundle By Name(w1385) -> ("Lockin.DAQ"=w1390:refnum<class "Instrument.DAQ.lvclass">, "Lockin"=w1387:refnum<class "Instrument.Lockin.lvclass">)
        n672 = Unbundle By Name(w1387) -> ("AO"=w1386:T52)
        n673 = call "DAQ.setAO.vi"("error in (no error)"=w1389, "AO Channels"=w1386, "Instrument.DAQ"=w1390) -> ("error out"=w1388:errorcluster)  [unwired: 7 in, 1 out]
        n674 = call <vilib>:"Add State(s) to Queue__jki_lib_state_machine.vi"("State(s) in (\"\")"=w1393) -> ("States Out"=w1392:string)  [unwired: 14 in]
      }
      frame "Lockin SMO: Set AO Zero Amplitude" {
        # "#lockin:process"
        n675 = Unbundle By Name(w1400) -> ("Lockin.DAQ"=w1407:refnum<class "Instrument.DAQ.lvclass">, "Lockin"=w1399:refnum<class "Instrument.Lockin.lvclass">)
        n676 = Unbundle By Name(w1399) -> ("AO"=w1394:T52, "#s"=w1405:i32, "Fs"=w1404:dbl)
        n677 = Divide(x=w1405, y=w1404) -> (x/y=w1397:dbl)
        n678 = Multiply(x=1000.0 ("y"), y=w1397) -> (x*y=w1403:dbl)
        n679 = for {
          tunnel: w1394 -> [w1413] mode=indexing
          tunnel: [w1411] -> w1396 mode=indexing
          n680 = Bundle By Name(cluster=w1413, "Amplitude"=0.0 ("element")) -> (w1411:T53)
        }
        n681 = To Unsigned Long Integer(number=w1403) -> (unsigned 32bit integer=w1402:u32)
        n682 = call "DAQ.setAO.vi"("error in (no error)"=w1406, "AO Channels"=w1396, "Instrument.DAQ"=w1407) -> ("error out"=w1395:errorcluster)  [unwired: 7 in, 1 out]
        n683 = call <userlib>:"Wait (ms)__ogtk.vi"("error in (no error)"=w1395, "milliseconds to wait"=w1402) -> ("error out"=w1401:errorcluster)  [unwired: 8 in, 1 out]
        n684 = call <vilib>:"Add State(s) to Queue__jki_lib_state_machine.vi"("State(s) in (\"\")"=w1410) -> ("States Out"=w1409:string)  [unwired: 14 in]
      }
      frame "Lockin SMO: Set REF" {
        # "#lockin:process"
        n685 = Unbundle By Name(w1416) -> ("Lockin.DAQ"=w1419:refnum<class "Instrument.DAQ.lvclass">, "Lockin"=w1417:refnum<class "Instrument.Lockin.lvclass">)
        n686 = Unbundle By Name(w1417) -> ("REF"=w1414:T38)
        n687 = call "DAQ.setREF.vi"("error in (no error)"=w1415, "Channels: Lockin"=w1414, "Instrument.DAQ"=w1419) -> ("error out"=w1418:errorcluster)  [unwired: 7 in, 1 out]
        n688 = call <vilib>:"Add State(s) to Queue__jki_lib_state_machine.vi"("State(s) in (\"\")"=w1422) -> ("States Out"=w1421:string)  [unwired: 14 in]
      }
      frame "Lockin SMO: Set AI" {
        # "#lockin:process"
        n689 = Unbundle By Name(w1427) -> ("Lockin.DAQ"=w1426:refnum<class "Instrument.DAQ.lvclass">, "Lockin"=w1428:refnum<class "Instrument.Lockin.lvclass">)
        n690 = Unbundle By Name(w1428) -> ("AI"=w1423:T57)
        n691 = call "DAQ.setAI.vi"("error in (no error)"=w1425, "AI Channels"=w1423, "Instrument.DAQ"=w1426) -> ("error out"=w1424:errorcluster)  [unwired: 7 in, 1 out]
        n692 = call <vilib>:"Add State(s) to Queue__jki_lib_state_machine.vi"("State(s) in (\"\")"=w1431) -> ("States Out"=w1430:string)  [unwired: 14 in]
      }
      frame "Lockin SMO: Set Input Gain" {
        # "#lockin:process"
        n693 = Unbundle By Name(w1432) -> ("Lockin.DAQ"=w1437:refnum<class "Instrument.DAQ.lvclass">, "Lockin"=w1435:refnum<class "Instrument.Lockin.lvclass">)
        n694 = Unbundle By Name(w1435) -> ("Input Gain"=w1434:dbl[])
        n695 = call "DAQ.setInputGain.vi"("error in (no error)"=w1433, "setInputGain"=w1434, "Instrument.DAQ"=w1437) -> ("error out"=w1436:errorcluster)  [unwired: 7 in, 1 out]
        n696 = call <vilib>:"Add State(s) to Queue__jki_lib_state_machine.vi"("State(s) in (\"\")"=w1440) -> ("States Out"=w1439:string)  [unwired: 14 in]
      }
      frame "Lockin SMO: Set Output Gain" {
        # "#lockin:process"
        n697 = Unbundle By Name(w1445) -> ("Lockin.DAQ"=w1444:refnum<class "Instrument.DAQ.lvclass">, "Lockin"=w1446:refnum<class "Instrument.Lockin.lvclass">)
        n698 = Unbundle By Name(w1446) -> ("Output Gain"=w1442:dbl[])
        n699 = call "DAQ.setOutputGain.vi"("error in (no error)"=w1443, "setOutputGain"=w1442, "Instrument.DAQ"=w1444) -> ("error out"=w1441:errorcluster)  [unwired: 7 in, 1 out]
        n700 = call <vilib>:"Add State(s) to Queue__jki_lib_state_machine.vi"("State(s) in (\"\")"=w1449) -> ("States Out"=w1448:string)  [unwired: 14 in]
      }
      frame "Lockin SMO: Set Prefilter" {
        # "#lockin:process"
        n701 = Unbundle By Name(w1452) -> ("Lockin.DAQ"=w1454:refnum<class "Instrument.DAQ.lvclass">, "Lockin"=w1455:refnum<class "Instrument.Lockin.lvclass">)
        n702 = Unbundle By Name(w1455) -> ("Prefilter"=w1453:T59)
        n703 = call "DAQ.setPreFilter.vi"("error in (no error)"=w1451, "PreFilter"=w1453, "Instrument.DAQ"=w1454) -> ("error out"=w1450:errorcluster)  [unwired: 7 in, 1 out]
        n704 = call <vilib>:"Add State(s) to Queue__jki_lib_state_machine.vi"("State(s) in (\"\")"=w1458) -> ("States Out"=w1457:string)  [unwired: 14 in]
      }
      frame "Lockin SMO: Calibration" {
        # "#lockin:process"
        n705 = Unbundle By Name(w1466) -> ("Lockin.DAQ"=w1465:refnum<class "Instrument.DAQ.lvclass">)
        n706 = Scan From String(input string=w1461, default 1=PrivateEvents--DAQ.setCalibration."Check" ("setCalibration")) -> (error out=w1459:errorcluster, output 1=w1460:T23)  [unwired: 3 in, 2 out]
        n707 = call <vilib>:"Clear Errors.vi"("error in (no error)"=w1459) -> ()  [unwired: 5 in, 2 out]
        n708 = call "DAQ.setCalibration.vi"("error in (no error)"=w1464, "setCalibration"=w1460, "Instrument.DAQ"=w1465) -> ("error out"=w1463:errorcluster)  [unwired: 7 in, 1 out]
        n709 = call <vilib>:"Add State(s) to Queue__jki_lib_state_machine.vi"("State(s) in (\"\")"=w1469) -> ("States Out"=w1468:string)  [unwired: 14 in]
      }
      frame "Lockin SMO: Auto DAQ" {
        # "#lockin:process"
        n710 = Unbundle By Name(w1473) -> ("Lockin.DAQ"=w1472:refnum<class "Instrument.DAQ.lvclass">)
        n711 = call "DAQ.autoConfigureDAQ.vi"("error in (no error)"=w1471, "Instrument.DAQ"=w1472) -> ("error out"=w1470:errorcluster)  [unwired: 8 in, 1 out]
        n712 = call <vilib>:"Add State(s) to Queue__jki_lib_state_machine.vi"("State(s) in (\"\")"=w1476) -> ("States Out"=w1475:string)  [unwired: 14 in]
      }
      frame "Lockin SMO: Reset Phase" {
        # "#lockin:process"
        n713 = Unbundle By Name(w1480) -> ("Lockin.DAQ"=w1479:refnum<class "Instrument.DAQ.lvclass">)
        n714 = call "DAQ.zeroPhase.vi"("error in (no error)"=w1478, "Instrument.DAQ"=w1479) -> ("error out"=w1477:errorcluster)  [unwired: 8 in, 1 out]
        n715 = call <vilib>:"Add State(s) to Queue__jki_lib_state_machine.vi"("State(s) in (\"\")"=w1483) -> ("States Out"=w1482:string)  [unwired: 14 in]
      }
      frame "Lockin SMO: Measure Offset" {
        # "#lockin:process"
        n716 = Unbundle By Name(w1484) -> ("Lockin.DAQ"=w1487:refnum<class "Instrument.DAQ.lvclass">)
        n717 = call "DAQ.measureOffset.vi"("error in (no error)"=w1486, "Instrument.DAQ"=w1487) -> ("error out"=w1485:errorcluster)  [unwired: 8 in, 1 out]
        n718 = call <vilib>:"Add State(s) to Queue__jki_lib_state_machine.vi"("State(s) in (\"\")"=w1490) -> ("States Out"=w1489:string)  [unwired: 14 in]
      }
      frame "Lockin SMO: Remove Offset" {
        # "#lockin:process"
        n719 = Unbundle By Name(w1492) -> ("Lockin.DAQ"=w1494:refnum<class "Instrument.DAQ.lvclass">)
        n720 = call "DAQ.zeroOffset.vi"("error in (no error)"=w1493, "Instrument.DAQ"=w1494) -> ("error out"=w1491:errorcluster)  [unwired: 8 in, 1 out]
        n721 = call <vilib>:"Add State(s) to Queue__jki_lib_state_machine.vi"("State(s) in (\"\")"=w1497) -> ("States Out"=w1496:string)  [unwired: 14 in]
      }
      frame "---------- 4461----------" {
        n722 = call <vilib>:"Add State(s) to Queue__jki_lib_state_machine.vi"("State(s) in (\"\")"=w1502) -> ("States Out"=w1501:string)  [unwired: 14 in]
      }
      frame "4461: SAMPLING SETUP" {
        # "#todo\n*I think* this \"macro\" needs to\nbe handled by Lockin.DAQ\nor Handle Command"
        # "#macro sorta"
        # "#todo\nshould this be in Lockin.DAQ SMO? or in Handle Command?"
        # "Max Fs"
        n723 = Unbundle By Name(w1508) -> ("Lockin"=w1506:refnum<class "Instrument.Lockin.lvclass">)
        n724 = case shown="Default" "DAQ Type" {
          tunnel: [102400.0 ("upper limit") 204800.0 ("upper limit")] -> w1510
          frame "USB 4431" {
          }
          frame Default {
          }
        }
        n725 = case shown="\"Auto Fs\"" "Sampling Mode" {
          tunnel: [w1519 w1520 w1534] -> w1511
          tunnel: w1506 -> [_ w1522 _]
          tunnel: w1510 -> [_ w1525 w1535]
          tunnel: "Max Fs Refresh Rate (Hz)" -> [_ _ w1530]
          frame "Manual", Default {
            n726 = local read "Sampling"() -> (w1519:T11)
          }
          frame "Auto Fs" {
            # "#todo: owned by Lockin or LockinDAQ?"
            # "#todo: make subVI?"
            # "max Fs"
            n727 = Unbundle By Name(w1522) -> ("AO"=w1526:T52)
            n728 = Index Array(array=w1526) -> (element=w1523:T53)  [unwired: 1 in]
            n729 = Unbundle By Name(w1523) -> ("Frequency"=w1521:dbl)
            n730 = Multiply(x="Auto x*F1", y=w1521) -> (x*y=w1524:dbl)
            n731 = In Range and Coerce(upper limit=w1525, x=w1524, lower limit=1000.0) -> (coerced(x)=w1529:dbl)  [unwired: 1 out]
            n732 = call "Fs and Ns for integer periods.vi"("f integer"=w1521, "Max Fs"=w1529) -> ("Timing out"=w1520:T11)  [unwired: 9 in]
          }
          frame "Max Fs" {
            n733 = Divide(x=w1535, y=w1530) -> (x/y=w1533:dbl)
            n734 = To Long Integer(number=w1533) -> (32bit integer=w1532:i32)
            n735 = Bundle By Name(cluster=T11 {"Fs"=204789.0, "#s"=15753} ("Sampling"), "Fs"=w1535, "#s"=w1532) -> (w1534:T11)
          }
        }
        n736 = call "Coerce Timing.vi"("Max Fs"=w1510, "Sampling in"=w1511) -> ("Sampling out"=w1504:T11)  [unwired: 9 in]
        n737 = Bundle By Name(cluster=w1506, "Sampling"=w1504) -> (w1505:refnum<class "Instrument.Lockin.lvclass">)
        n738 = Bundle By Name(cluster=w1508, "Lockin"=w1505) -> (w1507:T36)
        n739 = local write "Sampling"(w1504) -> ()
        n740 = call <vilib>:"Add State(s) to Queue__jki_lib_state_machine.vi"("State(s) in (\"\")"=w1516) -> ("States Out"=w1515:string)  [unwired: 14 in]
      }
      frame "4461: OUT" {
        # "#todo\nmove to Lockin.DAQ?"
        n741 = Unbundle By Name(w1537) -> ("Lockin"=w1540:refnum<class "Instrument.Lockin.lvclass">)
        n742 = case shown="True" "Enable Output" {
          tunnel: [w1544 w1553] -> w1538
          tunnel: w1540 -> [_ w1556]
          tunnel: w1536 -> [w1544 w1551]
          frame False {
          }
          frame True {
            # "this will act as a self-call\nmeaning after the remote call comes\nin the data on the data bus will get updated\nby other means"
            n743 = Unbundle By Name(w1556) -> ("Results (Dictionary)"=w1552:cluster{"key":string, "value":dbl}[], "Input Gain"=w1546:dbl[])
            n744 = call "Parse Results (single).vi"("Type"="Type", "error in (no error)"=w1551, "Reference Channel"="Reference Channel", "AI Channel"="AI Channel", "Results (Dictionary)"=w1552) -> ("error out"=w1550:errorcluster, "Data"=w1554:dbl)  [unwired: 3 in, 2 out]
            n745 = Decrement(x="AI Channel") -> (x-1=w1545:i32)
            n746 = Index Array(array=w1546, index=w1545) -> (element=w1555:dbl)
            n747 = Multiply(x=w1554, y=w1555) -> (x*y=w1557:dbl)
            "Output (V)" <- w1557
            n748 = call "setAO_DC.vi"("error in (no error)"=w1550, "DC (V)"=w1557, "AO Channel"="Output Channel", "Instrument.Lockin in"=w1556) -> ("error out"=w1553:errorcluster)  [unwired: 6 in, 1 out]
          }
        }
        n749 = call <vilib>:"Add State(s) to Queue__jki_lib_state_machine.vi"("State(s) in (\"\")"=w1542) -> ("States Out"=w1543:string)  [unwired: 14 in]
      }
      frame "4461: FFT" {
        n750 = Unbundle By Name(w1577) -> ("Lockin"=w1576:refnum<class "Instrument.Lockin.lvclass">)
        n751 = Unbundle By Name(w1576) -> ("AI"=w1566:waveform(dbl)[])
        n752 = Bundle By Name(cluster=T31 {"averaging mode"=enum."No averaging", "weighting mode"=enum."Exponential", "number of averages"=10} ("averaging parameters"), "averaging mode"="averaging mode", "weighting mode"="weighting mode", "number of averages"="# averages") -> (w1569:T31)
        n753 = call-poly <vilib>:"FFT Power Spectrum and PSD.vi"("export mode"="export mode", "averaging parameters"=w1569, "restart averaging (F)"="restart", "error in (no error)"=w1565, "dB On (F)"=TRUE, "window"="window", "time signals"=w1566) -> ("error out"=w1578:errorcluster, "averages completed"=→"averages":dbl, "averaging done"=→"done?":bool, "Power Spectrum / PSD"=w1562:cluster{"f0":dbl, "df":dbl, "magnitude":dbl[]}[])  [unwired: 1 in]
        "PS WFGraph" <- w1562
        n754 = control-ref of="PS WFGraph"() -> (w1559:refnum<vi>)
        n755 = for {
          tunnel: [w1585] -> w1564
          tunnel: w1565 -> [w1584]
          tunnel: w1562 -> [_] mode=indexing
          i -> [w1587]
          n756 = property on="PS WFGraph" class="WFGraph (strict)"(error in=w1584, "Active Plot"=w1587) -> (error out=w1588:errorcluster, "Plot.Visible?"=w1586:bool)  [unwired: 1 in, 1 out]
          n757 = property on="PS Chart" class="WFChart (strict)"(error in=w1588, "Active Plot"=w1587, "Plot.Visible?"=w1586) -> (error out=w1585:errorcluster)  [unwired: 1 in, 1 out]
        }
        n758 = call "PS Chart.vi"("error in (no error)"=w1578, "Power Spectrum / PSD"=w1562, "WFGraph (WDT) in"=w1559) -> ("error out"=w1561:errorcluster, "Chart"=→"PS Chart":dbl[][])  [unwired: 7 in]
        n759 = Merge Errors(w1561, w1564) -> (w1560:errorcluster)
        n760 = call <vilib>:"Add State(s) to Queue__jki_lib_state_machine.vi"("State(s) in (\"\")"=w1579) -> ("States Out"=w1583:string)  [unwired: 14 in]
      }
      frame "---------- Notes ----------" {
        n761 = call <vilib>:"Add State(s) to Queue__jki_lib_state_machine.vi"("State(s) in (\"\")"=w1593) -> ("States Out"=w1592:string)  [unwired: 14 in]
      }
      frame "Notes: Controls" {
        n762 = call <vilib>:"Add State(s) to Queue__jki_lib_state_machine.vi"("State(s) in (\"\")"=w1598) -> ("States Out"=w1597:string)  [unwired: 14 in]
      }
      frame "Notes: Notes" {
        # "calculate RMS, Noise bandwidth, etc"
        # "Go to \"4461: SETUP\" if Reset, remote mode,\nor IV/continuous mode buttons are pushed"
        # "Multichannel Lockin v2016/06/02 SW TIMED SINGLE POINT\nREF:\nhttp://www.ni.com/white-paper/3215/en/ Example 9"
        # "TO DO:\n- intelligent decimate to dt setpoint\ncalculate RMS, Noise bandwidth, etc"
        n763 = disable-structure shown="Enabled" {
          frame Disabled {
            n764 = call <vilib>:"Open Config Data.vi"() -> ()  [unwired: 9 in, 3 out]
          }
          frame Enabled {
            # "JKI State Machine™\nhttp://jkisoft.com/state-machine/\nCopyright (C) 2005-2008, JKI <info@jkisoft.com>\nALL RIGHTS RESERVED"
            # "State Syntax:\nStateCategory: State >> Argument\nLine Terminator: Line feed\nExample:\nUI: Help >> About\n\nWhere \"UI\" is the state category\nWhere \"Help\" is the state\nWhere \"About\" is the argument\nOther Examples:\nApp Data: Initialize\nUI: Initialize\nHelp >> About\n\nCommenting:\nTo add a comment use \"//\" or \"#\" and all text to the right will be ignored\n\nCommenting Example:\nUI: Initialize // This initializes the UI\n# This whole line is a comment\n// Another comment line"
          }
        }
        n765 = call <vilib>:"Add State(s) to Queue__jki_lib_state_machine.vi"("State(s) in (\"\")"=w1603) -> ("States Out"=w1602:string)  [unwired: 14 in]
      }
    }
    n766 = call <userlib>:"State History.vi"("Current State"=w9) -> ("History"=→"State History":string)  [unwired: 6 in]
  }
